vi "MAIN.vi"() -> ()   [LabVIEW 2015]
doc: "Use this template to create an application that executes repeatedly until you click the Stop button. This template polls the state of the Stop button and does not use events. Use the Top-Level Application template (not available in the Base package) to create a single-loop application with event handling."
uses:
  Control-CDC data.ctl
  Control-IMU data.ctl
  Control-Operation Test State FTS.ctl
  Lib_Bled112 toolkit/type_def/connection_status_bundle.ctl
  Lib_Bled112 toolkit/type_def/address_type.ctl
  Control-BLED Rx (EVENT-Attribute Client).ctl
  Lib_Bled112 toolkit/type_def/message_type.ctl
  Lib_Bled112 toolkit/type_def/message_class.ctl
  sub/Operation mode.ctl
  sub/Linerity State.ctl
  Cluster Type/Cal information.ctl
  Cluster Type/Device information.ctl
  <vilib>/Utility/miscctls.llb/LVPointTypeDef.ctl
  SUB_Load and Save Controls.llb/RWC_Actions.ctl
  <vilib>/Utility/miscctls.llb/LVRowAndColumnTypeDef.ctl
  Cluster Type/Acclerometer value(90, 180).ctl
  Type definition/write_mode.ctl
  Control-Operation State Mark10.ctl
  <vilib>/event_ctls.llb/eventvkey.ctl
  sub/File Control/File_Control_mode.ctl
  <vilib>/Analysis/baseanly.llb/Mean (DBL).vi
  <vilib>/Utility/config.llb/Read Key (String).vi
  <vilib>/Utility/config.llb/Read Key (I32).vi
  Lib_Bled112 toolkit/ble_functions/ble_write_by_handle_uint8array.vi
  global 3.vi
  global 4.vi
  Global 1.vi
  <vilib>/Utility/config.llb/Write Key (String).vi
  <vilib>/Utility/config.llb/Write Key (U32).vi
  <vilib>/Utility/config.llb/NI_LVConfig.lvlib
  <vilib>/Analysis/NI_AALBase.lvlib
  <vilib>/Utility/sysdir.llb/System Directory Type.ctl
  <vilib>/Utility/NIReport.llb/NI_report.lvclass
  <vilib>/addons/_office/NI_ReportGenerationToolkit.lvlib
  <vilib>/addons/_office/excel.llb/Excel Easy Table (str).vi
  <vilib>/Utility/NIReport.llb/Excel/NI_Excel.lvclass
  <vilib>/addons/_office/_exclsub.llb/font.ctl
panel:
  out "scale A,B check":u8
  out "scale A,B":T1 {"Check sum 2" format="%x"; "Device Type L" format="%x"; "Device Type H" format="%x"; "Check sum" format="%x"; "Scale B" format="%x"; "Scale A" format="%x"; "Manufacturer Lot ID 4" format="%x"; "Manufacturer Lot ID 3" format="%x"; "Manufacturer Lot ID 2" format="%x"; "Manufacturer Lot ID 1" format="%x"; "Day" format="%x"; "Month" format="%x"; "Year" format="%x"; "Device ID 4" format="%x"; "Device ID 3" format="%x"; "Device ID 2" format="%x"; "Device ID 1" format="%x"; "Packet ID" format="%x"}
  out "A3 rx":bool
  in  "A3 tx":bool
  out "A1 rx":bool
  in  "A1 tx":bool
  out "Port-act 1":refnum<visa-resource-name>="COM8"
  out "cal factor B":u8
  out "cal factor A":u8
  out "scale B":dbl format="%.2f"
  out "scale A":dbl format="%.2f"
  in  "PWR OFF":bool
  in  "File Path Done":bool
  in  "Linerity State":T2
  in  "Mode":bool=TRUE
  out "Bat(raw)":u16 format="%04x"
  out "Disconnection ocurrence":refnum<k4>
  out "Test Data table for Load Accuarcy Test":string[][](table)=[["-", "-", "-", "-", "-", "-", "-"], ["-", "-", "-", "-", "-", "-", "-"], ["-", "-", "-", "-", "-", "-", "-"], ["-", "-", "-", "-", "-", "-", "-"], ["-", "-", "-", "-", "-", "-", "-"], ["-", "-", "-", "-", "-", "-", "-"], ["-", "-", "-", "-", "-", "-", "-"], ["-", "-", "-", "-", "-", "-", "-"], ["-", "-", "-", "-", "-", "-", "-"]]
  out "Packet No.":u16
  out "Rx-debug":bool
  out "FTS table index":i32
  out "ms timer 5":u32=38996702
  out "ms timer 4":u32=27271323
  out "ms timer 3":u32=38996702
  in  "Update(ms)":u16=100
  out "ms timer 2":u32=38996702
  out "Rx-ROM":bool
  out "BLE Packet (mon)":u8[](array[numeric])=[119, 32, 48, 163, 32, 0, 45, 32, 53, 143, 30, 162, 83, 32, 86, 151, 32, 67, 185, 208, 89, 94, 66, 75, 91, 193, 107, 187, 98, 158, 102, 165, 208]
  out "Timer-ble log":u32=38996556
  in  "log data1":bool
  out "log ble buf":string
  out "Packet Detect":bool
  out "Disconnected":bool
  out "Rx buf 1":string
  out "Rx Cnt":i32
  out "Rx Packet Structure":T3={"Message Type (Response)"=128, "Payload length"=25, "Command Class (System)"=4, "Message ID"=5, "Connection handle"=0, "Attribute handle"=11, "Attribute type"=1, "Attribute value (data)"=[119, 32, 48, 110, 31, 255, 217, 32, 53, 83, 30, 161, 69, 32, 87, 130, 32, 68, 21, 209]} {"Attribute type" format="%02x" items=["read", "notify", "indicate", "read_by_type", "read_blob", "indicate_rsp_req"]; "Attribute value (data)" format="%02x"; "Attribute handle" format="%04x"; "Connection handle" format="%02x"; "Message ID" format="%02x"; "Message Type (Response)" format="%02x" items=["Command / Response"=0, "Event"=128]; "Command Class (System)" format="%02x" items=["System", "Persistent Store", "Attribute database", "Connection", "Attribute client", "Security Manager", "Generic Access Profile", "Hardware"]}
  out "Device Name":string="GEN4_PERSONA_3rd_jun"
  out "Connection Status":T6={"MAC Address"="F8:B8:54:EF:76:8D", "cnx handle"=0, "cnx flags"=5, "Address Type"=1, "Connection Interval (ms)"=8, "Timeout(ms)"=1000, "Latency"=0, "bonding handle"=255} {"Address Type" items=["Public", "Random"]}
  in  "Log no":string="1" caption="No."
  in  "FTS OP status":T8="Test_Start"
  out "Test profile":string[][](array[string])=[["Load(1)-0lb", "0", "1000", "0", "0"], ["Init(1)-70lb", "70", "1000", "0", "0"], ["Init(2)-140lb", "140", "1000", "0", "0"], ["Init(1)-70lb", "70", "1000", "0", "0"], ["Init(2)-140lb", "140", "1000", "0", "0"], ["Load(1)-0lb", "0", "10000", "1", "1"], ["Load(2)-10lb", "10", "3000", "0", "1"], ["Load(3)-20lb", "20", "3000", "0", "1"], ["Load(4)-40lb", "40", "3000", "0", "1"], ["Load(5)-60lb", "60", "3000", "0", "1"], ["Load(6)-80lb", "80", "3000", "0", "1"]]
  out "log refnum":refnum<file> caption="참조 번호 복제"
  out "ms timer":u32=38996556
  out "Logging No.":u32
  in  "Data Logging":bool caption="Data Logging (Desktop folder)"
  out "RxD":string
  out "Graph timer 2":u32=38996702
  out "Maximize window":bool
  out "Comm err cnt 1":i32
  out "Graph timer 1":u32=38996702
  in  "Setting load":bool=TRUE
  out "ACT-Comm":bool
  in  "Comm con 1":bool
  in  "Port close 1":bool
  in  "Port open 1":bool
  in  "탭-Top":T9(tab)
  out "recall-2":bool
  in  "CDC Graph plot":bool
  in  "Offset Souce":enum32{"Normal", "Raw"}(radio)
  out "CDC Offet":T10 caption="CDC Offset data" {"Right Wing-C, C6/C0" format="%#.9f"; "Right Wing-B, C5/C0" format="%#.9f"; "Right Wing-A, C4/C0" format="%#.9f"; "Left Wing-C, C3/C0" format="%#.9f"; "Left Wing-B, C2/C0" format="%#.9f"; "Left Wing-A, C1/C0" format="%#.9f"}
  in  "Export graph 1":bool
  in  "Clear graph 1":bool
  out "CDC(PCAP02) Graph":waveform(dbl)[](graph)=[{"t0"=timestamp(3566271640.952271 s since 1904-01-01), "dt"=0.10400000000000001, "Y"=[22878.0]}, {"t0"=timestamp(3566271640.952271 s since 1904-01-01), "dt"=0.10400000000000001, "Y"=[16971.0]}, {"t0"=timestamp(3566271640.952271 s since 1904-01-01), "dt"=0.10400000000000001, "Y"=[23489.0]}, {"t0"=timestamp(3566271640.952271 s since 1904-01-01), "dt"=0.10400000000000001, "Y"=[27579.0]}, {"t0"=timestamp(3566271640.952271 s since 1904-01-01), "dt"=0.10400000000000001, "Y"=[25246.0]}, {"t0"=timestamp(3566271640.952271 s since 1904-01-01), "dt"=0.10400000000000001, "Y"=[26279.0]}, {"t0"=timestamp(3566271640.952271 s since 1904-01-01), "dt"=0.10400000000000001, "Y"=[1.0058650970458984]}, {"t0"=timestamp(3566271640.952271 s since 1904-01-01), "dt"=0.10400000000000001, "Y"=[0.9999599456787109]}, {"t0"=timestamp(3566271640.952271 s since 1904-01-01), "dt"=0.10400000000000001, "Y"=[1.0064787864685059]}, {"t0"=timestamp(3566271640.952271 s since 1904-01-01), "dt"=0.10400000000000001, "Y"=[0.9571785926818848]}, {"t0"=timestamp(3566271640.952271 s since 1904-01-01), "dt"=0.10400000000000001, "Y"=[1.0106620788574219]}, {"t0"=timestamp(3566271640.952271 s since 1904-01-01), "dt"=0.10400000000000001, "Y"=[1.0083107948303223]}]
  out "CDC data":T10 caption="CDC Monitoring data" {"Right Wing-C, C6/C0" format="%#.9f"; "Right Wing-B, C5/C0" format="%#.9f"; "Right Wing-A, C4/C0" format="%#.9f"; "Left Wing-C, C3/C0" format="%#.9f"; "Left Wing-B, C2/C0" format="%#.9f"; "Left Wing-A, C1/C0" format="%#.9f"}
  in  "Offset 1":bool
  out "FTS 42 Rx":bool
  out "IMU Offet":T11 caption="IMU Offset data" {"Accelerometer Z" format="%#.9f"; "Accelerometer Y" format="%#.9f"; "Accelerometer X" format="%#.9f"; "Gyroscope Z" format="%#.9f"; "Gyroscope Y" format="%#.9f"; "Gyroscope X" format="%#.9f"}
  out "IMU Graph":waveform(dbl)[](graph)=[{"t0"=timestamp(3566271136.852438 s since 1904-01-01), "dt"=0.108, "Y"=[-1.063125]}, {"t0"=timestamp(3566271136.852438 s since 1904-01-01), "dt"=0.108, "Y"=[0.118125]}, {"t0"=timestamp(3566271136.852438 s since 1904-01-01), "dt"=0.108, "Y"=[0.20125]}, {"t0"=timestamp(3566271136.852438 s since 1904-01-01), "dt"=0.108, "Y"=[-0.014029999999999999]}, {"t0"=timestamp(3566271136.852438 s since 1904-01-01), "dt"=0.108, "Y"=[-0.00366]}, {"t0"=timestamp(3566271136.852438 s since 1904-01-01), "dt"=0.108, "Y"=[1.0149789999999999]}]
  in  "Clear graph 2":bool
  in  "Export graph2":bool
  out "IMU data":T11 caption="IMU Monitoring data" {"Accelerometer Z" format="%#.9f"; "Accelerometer Y" format="%#.9f"; "Accelerometer X" format="%#.9f"; "Gyroscope Z" format="%#.9f"; "Gyroscope Y" format="%#.9f"; "Gyroscope X" format="%#.9f"}
  in  "Offset 2":bool
  out "Full ROM data":bool
  in  "Flash Map":enum32{"Data Map", "Raw Data"}(tab)
  out "ROM Table":string[][](table)=[["Serial number", "-", "-"], ["YEAR", "-", "-"], ["Month", "-", "-"], ["Day", "-", "-"], ["Device ID", "-", "-"], ["Manufacturer ID", "-", "-"], ["Cal_Scale A", "-", "-"], ["Cal_Scale B", "-", "-"], ["Cal_Acc. X", "-", "-"], ["Cal_Acc. Y", "-", "-"], ["Cal_Acc. Z", "-", "-"], ["Cal_Gy. X", "-", "-"], ["Cal_Gy. Y", "-", "-"], ["Cal_Gy. Z", "-", "-"], ["Cal_Vol H", "-", "-"], ["Cal_Vol L", "-", "-"], ["Cal_CDC Off 1", "-", "-"], ["Cal_CDC Off 2", "-", "-"], ["Cal_CDC Off 3", "-", "-"], ["Cal_CDC Off 4", "-", "-"], ["Cal_CDC Off 5", "-", "-"], ["Cal_CDC Off 6", "-", "-"], ["Cal_CDC Off 7", "-", "-"], ["Cal_CDC Off 8", "-", "-"], ["Firmware Revision", "-", "-"], ["Operative Side", "-", "-"], ["Cal_Compart. A_10", "-", "-"], ["Cal_Compart. B_10", "-", "-"], ["Reserved", "-", "-"], ["Cal_Compart. A_11", "-", "-"], ["Cal_Compart. B_11", "-", "-"], ["Cal_Compart. A_12", "-", "-"], ["Cal_Compart. B_12", "-", "-"], ["Cal_Compart. A_13", "-", "-"], ["Cal_Compart. B_13", "-", "-"], ["Cal_Compart. A_14", "-", "-"], ["Cal_Compart. B_14", "-", "-"], ["Cal_Compart. A_16", "-", "-"], ["Cal_Compart. B_16", "-", "-"], ["Reserved", "-", "-"], ["Acc. X_0 value", "-", "-"], ["Acc. Y_0 value", "-", "-"], ["Acc. Z_0 value", "-", "-"], ["Acc. X_45 value", "-", "-"], ["Acc. Y_45 value", "-", "-"], ["Acc. Z_45 value", "-", "-"], ["Reserved", "-", "-"], ["Acc. X_90 value", "-", "-"], ["Acc. Y_90 value", "-", "-"], ["Acc. Z_90 value", "-", "-"], ["Acc. X_180 value", "-", "-"], ["Acc. Y_180 value", "-", "-"], ["Acc. Z_180 value", "-", "-"], ["Second counter", "-", "-"], ["Reserved", "-", "-"], ["", "", ""], ["", "", ""], ["", "", ""], ["", "", ""], ["", "", ""], ["", "", ""], ["", "", ""], ["", "", ""], ["", "", ""], ["", "", ""], ["", "", ""], ["", "", ""], ["", "", ""], ["", "", ""], ["", "", ""]]
  out "Rx ROM-log":string
  out "ROM Data":T12(array[cluster]) {"Index" format="%02x"; "ROM Data" format="%02x"}
  in  "Re-call":bool
  in  "Operation Mode":T13
  in  "Mode Selection":bool
  in  "Data Log":string
  out "Data_mon(h)":string
  in  "Data(h)":string="\u0001"
  in  "Send":bool
  in  "Handle":u8=15 format="%02x"
  in  "Mode Protocol":enum32{"Normal", "Debugging 1", "Debugging 2"}(tab)
  out "data out":u8[](array[numeric])
  in  "Reset Avg":bool caption="Reset"
  out "BLE RSSI Avg(dBm)":dbl format="%.1f"
  out "BLE Interval Time Avg(ms)":dbl format="%.1f"
  in  "File path":path
  in  "All Graph data save":bool
  in  "Set Inverval Time":bool
  in  "Grahp Clear":bool
  out "BLE RSSI buf":i16(graph)=-63
  out "BLE RSSI Graph":dbl(graph)=-65.56666666666666
  out "BLE RSSI (dBm)":dbl format="%.1f"
  out "BLE AVG-Interval Graph":dbl(graph)=11.355
  out "BLE Interval Time(ms)":dbl format="%.1f"
  out "BLE Interval buf":u32(graph)=11
  in  "Interval Time":enum16{"10ms", "33ms", "50ms"}(ring)
  out "second counter Rx":bool
  out "42 Rx":bool
  out "42 Tx":bool
  out "Battery cal Rx":bool
  out "Error":bool
  in  "battery cal Tx":bool
  out "battery cal complete boolean":bool
  out "Battery(V)":dbl format="%#_3g"
  out "inspection boolean":bool
  out "Linearity monitoring graph":cluster{dbl[], dbl[]}(graph)
  in  "ADC Linearity Start":bool
  out "battery cal value":dbl[](array[numeric])
  out "Status":string
  out "x/y":dbl
  out "Cal information":T14 {"Check sum" format="%x"; "Voltage L 2.8V" format="%x"; "Voltage H 2.8V" format="%x"; "Voltage L 3.1V" format="%x"; "Acc Z_L_Cal" format="%x"; "Voltage H 3.1V" format="%x"; "Gyro Z_L_Cal" format="%x"; "Gyro Z_H_Cal" format="%x"; "Gyro Y_L_Cal" format="%x"; "Gyro Y_H_Cal" format="%x"; "Gyro X_L_Cal" format="%x"; "Gyro X_H_Cal" format="%x"; "Acc Z_H_Cal" format="%x"; "Acc Y_L_Cal" format="%x"; "Acc Y_H_Cal" format="%x"; "Acc X_L_Cal" format="%x"; "Acc X_H_Cal" format="%x"; "Packet ID" format="%x"}
  out "cluster":T14 {"Check sum" format="%x"; "Voltage L 2.8V" format="%x"; "Voltage H 2.8V" format="%x"; "Voltage L 3.1V" format="%x"; "Acc Z_L_Cal" format="%x"; "Voltage H 3.1V" format="%x"; "Gyro Z_L_Cal" format="%x"; "Gyro Z_H_Cal" format="%x"; "Gyro Y_L_Cal" format="%x"; "Gyro Y_H_Cal" format="%x"; "Gyro X_L_Cal" format="%x"; "Gyro X_H_Cal" format="%x"; "Acc Z_H_Cal" format="%x"; "Acc Y_L_Cal" format="%x"; "Acc Y_H_Cal" format="%x"; "Acc X_L_Cal" format="%x"; "Acc X_H_Cal" format="%x"; "Packet ID" format="%x"}
  out "FTS start":bool
  out "FTS device out":bool
  out "scale A,B Rx":bool
  out "scale A.B Tx":bool
  out "second counter Tx":bool
  in  "Cal/Test select":bool=TRUE
  in  "Head Up":bool
  in  "Load(lb)":dbl=10.0 min=0.0 max=150.0 step=0.1
  in  "Test name":string="Noname"
  out "Load Graph":cluster{dbl[], dbl[]}(graph)
  out "Mark10 Gauge (lb)":dbl format="%.2f"
  out "Test Status":string
  out "Test Data table":string[][](table)=[["-", "-", "-", "-", "-", "-", "-"], ["-", "-", "-", "-", "-", "-", "-"], ["-", "-", "-", "-", "-", "-", "-"], ["-", "-", "-", "-", "-", "-", "-"], ["-", "-", "-", "-", "-", "-", "-"], ["-", "-", "-", "-", "-", "-", "-"], ["-", "-", "-", "-", "-", "-", "-"], ["-", "-", "-", "-", "-", "-", "-"], ["-", "-", "-", "-", "-", "-", "-"]]
  in  "Test Start":bool
  in  "Port-FTS":refnum<visa-resource-name>="COM6" caption="FTS \nCOM port"
  in  "FTS Testing":bool
  out "FTS comm.":bool
  in  "Force Set":bool
  out "FTS 42 Tx":bool
  out "88 rx":bool
  out "83 rx":bool
  in  "88 tx":bool
  in  "83 tx":bool
  out "81 rx":bool
  in  "Save":bool
  in  "ROM Table 2":string[][](table)=[["Serial number", "1", "MAX Value: 4294967295 (FFFFFFFFh)"], ["YEAR", "2", "Year: 2002, MAX Value: 255 (FFh)"], ["Month", "3", "Month:  3, MAX Value: 255 (FFh)"], ["Day", "4", "Day:  4, MAX Value: 255 (FFh)"], ["Device ID", "5", "-"], ["Manufacturer ID", "6", "MAX Value: 4294967295 (FFFFFFFFh)"], ["Cal_Scale A", "7", "MAX Value: 255 (FF)"], ["Cal_Scale B", "8", "MAX Value: 255 (FF)"], ["Cal_Acc. X", "9", "-"], ["Cal_Acc. Y", "10", "-"], ["Cal_Acc. Z", "11", "-"], ["Cal_Gy. X", "12", "-"], ["Cal_Gy. Y", "13", "-"], ["Cal_Gy. Z", "14", "-"], ["Cal_Vol H", "2910", "-"], ["Cal_Vol L", "16", "-"], ["Cal_CDC Off 1", "17", "-"], ["Cal_CDC Off 2", "18", "-"], ["Cal_CDC Off 3", "19", "-"], ["Cal_CDC Off 4", "20", "-"], ["Cal_CDC Off 5", "21", "-"], ["Cal_CDC Off 6", "22", "-"], ["Cal_CDC Off 7", "23", "-"], ["Cal_CDC Off 8", "24", "-"], ["Firmware Revision", "25", "-"], ["Operative Side", "26", "-"], ["Cal_Compart. A_10", "27", "-"], ["Cal_Compart. B_10", "28", "-"], ["Reserved", "29", "-"], ["Cal_Compart. A_11", "30", "-"], ["Cal_Compart. B_11", "31", "-"], ["Cal_Compart. A_12", "32", "-"], ["Cal_Compart. B_12", "33", "-"], ["Cal_Compart. A_13", "34", "-"], ["Cal_Compart. B_13", "35", "-"], ["Cal_Compart. A_14", "36", "-"], ["Cal_Compart. B_14", "37", "-"], ["Cal_Compart. A_16", "38", "-"], ["Cal_Compart. B_16", "39", "-"], ["Reserved", "40", "-"], ["Acc. X_0 value", "41", "-"], ["Acc. Y_0 value", "42", "-"], ["Acc. Z_0 value", "43", "-"], ["Acc. X_45 value", "44", "-"], ["Acc. Y_45 value", "45", "-"], ["Acc. Z_45 value", "46", "-"], ["Reserved", "47", "-"], ["Acc. X_90 value", "48", "-"], ["Acc. Y_90 value", "49", "-"], ["Acc. Z_90 value", "50", "-"], ["Acc. X_180 value", "51", "-"], ["Acc. Y_180 value", "52", "-"], ["Acc. Z_180 value", "53", "-"], ["Second counter", "17454", "-"], ["Reserved", "8", "-"], ["", "", ""], ["", "", ""], ["", "", ""], ["", "", ""], ["", "", ""], ["", "", ""], ["", "", ""], ["", "", ""], ["", "", ""], ["", "", ""], ["", "", ""], ["", "", ""], ["", "", ""], ["", "", ""], ["", "", ""]] caption="ROM Table"
  out "x-y":u8 format="%x"
  out "81 checksum":u8
  out "91 checksum":u8
  out "83 checksum":u8
  out "88 checksum":u8
  out "bat cal_check sum":u8
  out "sec coun_check sum":u8
  in  "91 tx":bool
  out "91 rx":bool
  out "A3 checksum":u8
  out "A1 checksum":u8
  out "98 checksum":u8
  out "94 checksum":u8
  out "92 checksum":u8
  in  "92 tx":bool
  out "92 rx":bool
  in  "94 tx":bool
  out "94 rx":bool
  in  "98 tx":bool
  out "98 rx":bool
  out "Rx-mon":bool
  out "Comm con status 1":bool caption="Status"
  out "*Board ID1":string="None...." caption="S/N"
  in  "Port-set 1":refnum<visa-resource-name>="COM8" caption="COM port"
  in  "stop":bool=TRUE
  out "Data trx(led)":bool
  in  "Setting load(led)":bool
  out "status string":string="Ready (available after the communication connection)"
  # "GEN4 PP4 - GUI Program"
  # "Ver. 170823A"
  # "Comm. Connection"
  # "(Connection)"
  # "Serial port"
  # "Reserved"
  # "Gyroscope X"
  # "Gyroscope Y"
  # "Gyro. (dps)"
  # "Gyroscope Z"
  # "Accelerometer X"
  # "Accelerometer Y"
  # "Acc. (g)"
  # "Accelerometer Z"
  # "Unless otherwise specified, Maximum value is 65535(FFFFh)."
  # "* Normal Operation Mode\nHandler : 0x000B\nWrite : 0x69 0x6D 0x74"
  # "* Debugging Mode 1\nHandler : 0x000B\nWrite : 0x4A 0x73 0x50"
  # "* Debugging Mode 2\nHandler : 0x000B\nWrite : 0x4E 0x46 0x54"
  # "Battery Calibration"
  # "ESM301: 115200bps\nMARK10: 9600bps"
  # "Unless otherwise specified, Maximum value is 65535 (FFFFh)."
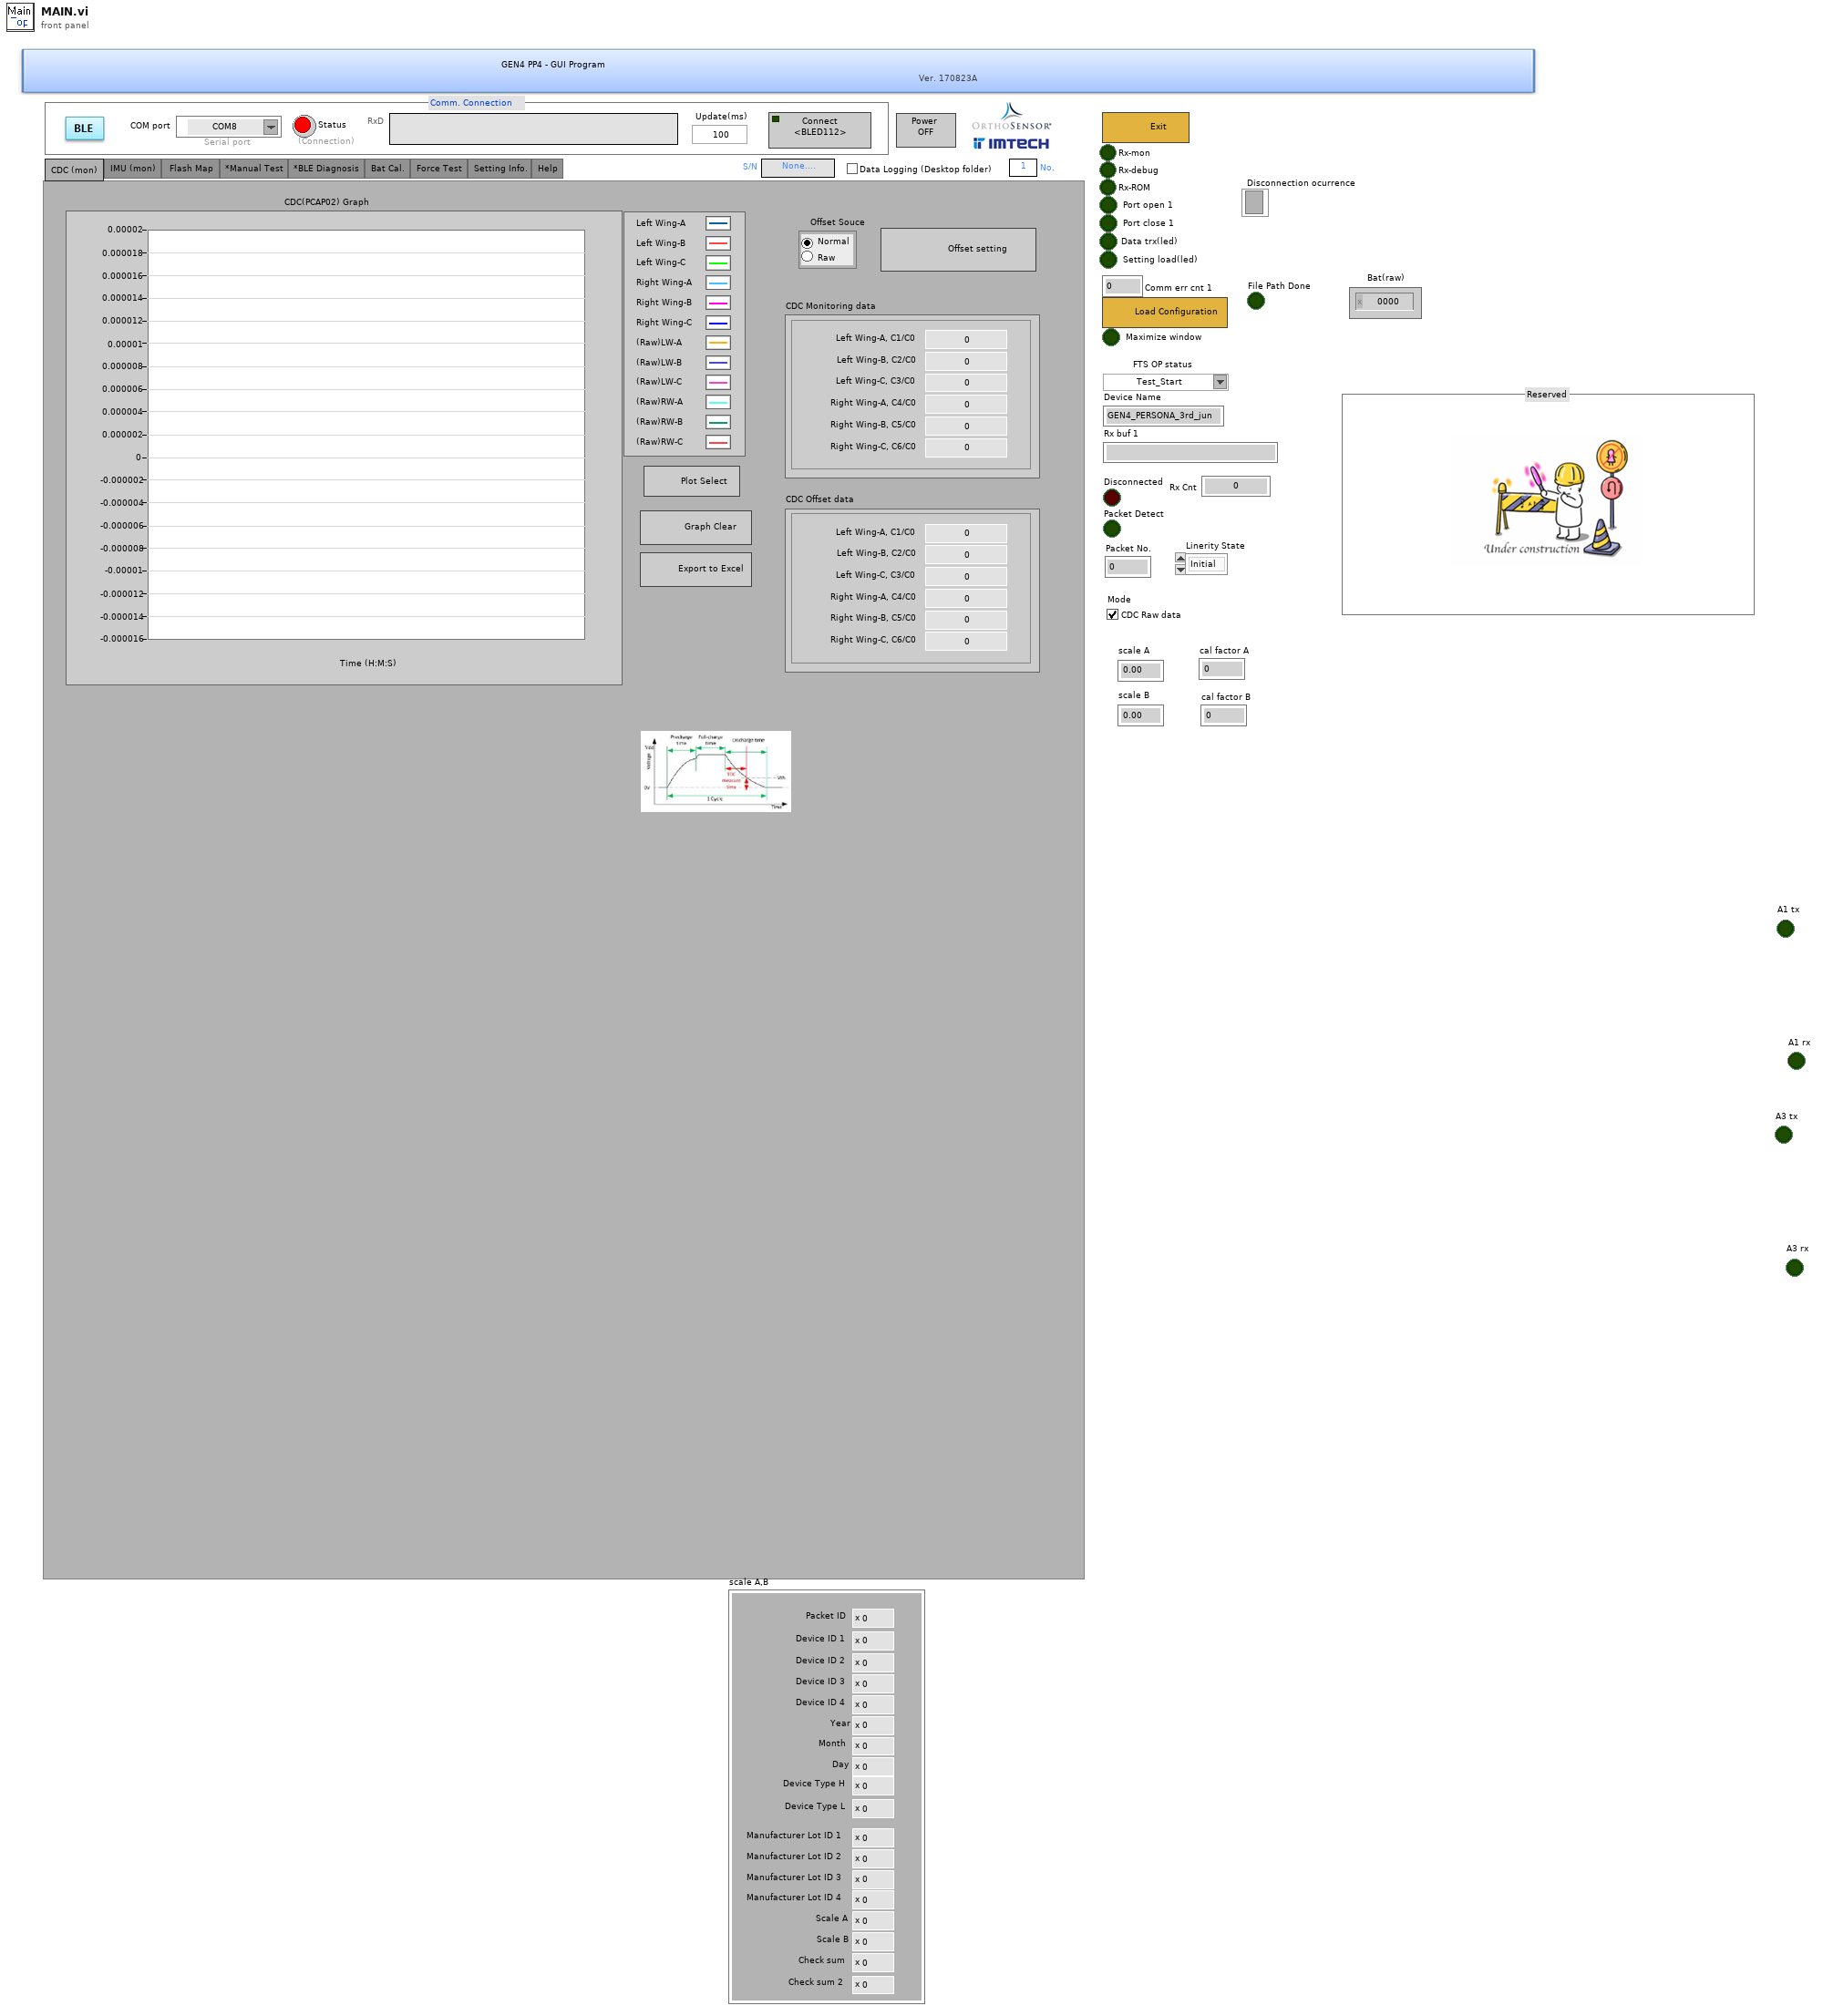
[diagram p1: front panel]
types:
  T1 = typedef "Device information.ctl" = cluster{"Packet ID":u8, "Device ID 1":u8, "Device ID 2":u8, "Device ID 3":u8, "Device ID 4":u8, "Year":u8, "Month":u8, "Day":u8, "Device Type H":u8, "Device Type L":u8, "Manufacturer Lot ID 1":u8, "Manufacturer Lot ID 2":u8, "Manufacturer Lot ID 3":u8, "Manufacturer Lot ID 4":u8, "Scale A":u8, "Scale B":u8, "Check sum":u8, "Check sum 2":u8}
  T2 = typedef "Linerity State.ctl" = enum16{"Initial", "Measurement", "End"}
  T3 = typedef "Control-BLED Rx (EVENT-Attribute Client).ctl" = cluster{"Message Type (Response)":T4, "Payload length":u8, "Command Class (System)":T5, "Message ID":u8, "Connection handle":u8, "Attribute handle":u16, "Attribute type":T5, "Attribute value (data)":u8[]}
  T4 = typedef "message_type.ctl" = u8
  T5 = typedef "message_class.ctl" = u8
  T6 = typedef "connection_status_bundle.ctl" = cluster{"MAC Address":string, "cnx handle":u8, "cnx flags":u8, "Address Type":T7, "Connection Interval (ms)":u16, "Timeout(ms)":u16, "Latency":u16, "bonding handle":u8}
  T7 = typedef "address_type.ctl" = u8
  T8 = typedef "Control-Operation Test State FTS.ctl" = string
  T9 = enum32{"CDC (mon)", "IMU (mon)", "Flash Map ", "*Manual Test", "*BLE Diagnosis", "Bat Cal.", "Force Test", "Setting Info.", "Help"}
  T10 = typedef "Control-CDC data.ctl" = cluster{"Left Wing-A, C1/C0":dbl, "Left Wing-B, C2/C0":dbl, "Left Wing-C, C3/C0":dbl, "Right Wing-A, C4/C0":dbl, "Right Wing-B, C5/C0":dbl, "Right Wing-C, C6/C0":dbl}
  T11 = typedef "Control-IMU data.ctl" = cluster{"Gyroscope X":dbl, "Gyroscope Y":dbl, "Gyroscope Z":dbl, "Accelerometer X":dbl, "Accelerometer Y":dbl, "Accelerometer Z":dbl}
  T12 = cluster{"RxOK":bool, "ROM Data":u8[], "Index":u8}[]
  T13 = typedef "Operation mode.ctl" = enum16{"Normal Operation", "Debugging 1", "Debugging 2"}
  T14 = typedef "Cal information.ctl" = cluster{"Packet ID":u8, "Acc X_H_Cal":u8, "Acc X_L_Cal":u8, "Acc Y_H_Cal":u8, "Acc Y_L_Cal":u8, "Acc Z_H_Cal":u8, "Acc Z_L_Cal":u8, "Gyro X_H_Cal":u8, "Gyro X_L_Cal":u8, "Gyro Y_H_Cal":u8, "Gyro Y_L_Cal":u8, "Gyro Z_H_Cal":u8, "Gyro Z_L_Cal":u8, "Voltage H 3.1V":u8, "Voltage L 3.1V":u8, "Voltage H 2.8V":u8, "Voltage L 2.8V":u8, "Check sum":u8}
  T15 = enum8{"Enabled", "Disabled", "Disabled and Grayed Out"}
  T16 = typedef "RWC_Actions.ctl" = enum16{"Read", "Write", "Read and Create"}
  T17 = enum16{"Always On", "Always Off", "Off While Running"}
  T18 = typedef "LVPointTypeDef.ctl" = cluster{"Horizontal":i16, "Vertical":i16}
  T19 = cluster{"RxOK":bool, "ROM Data":u8[], "Index":u8}
  T20 = typedef "LVRowAndColumnTypeDef.ctl" = cluster{"Row":i32, "Column":i32}
  T21 = enum16{"Standard Report", "HTML", "Word", "Excel"}
  T22 = enum16{"maximized", "minimized", "normal", "no change"}
  T23 = typedef "NI_ReportGenerationToolkit.lvlib/font.ctl" = cluster{"font name":string, "font size":dbl, "bold":u16, "italic":u16, "underline":u16, "strike through":u16, "font color":u32}
  T24 = cluster{"on/off":bool, "weight":i32, "color":u32}
  T25 = typedef "Acclerometer value(90, 180).ctl" = cluster{"Packet ID":u8, "Acc. X_90 val_H":u8, "Acc. X_90 val_L":u8, "Acc. Y_90 val_H":u8, "Acc. Y_90 val_L":u8, "Acc. Z_90 val_H":u8, "Acc. Z_90 val_L":u8, "Acc. X_180 val_H":u8, "Acc. X_180 val_L":u8, "Acc. Y_180 val_H":u8, "Acc. Y_180 val_L":u8, "Acc. Z_180 val_H":u8, "Acc. Z_180 val_L":u8, "second counter_1":u8, "second counter_2":u8, "Reserved_1":u8, "Reserved_2":u8, "Check sum":u8}
  T26 = typedef "write_mode.ctl" = enum16{"Save Flash", "Visa save", "Interval Change"}
  T27 = typedef "Control-Operation State Mark10.ctl" = string
  T28 = typedef "eventvkey.ctl" = enum16{"ASCII", "Enter", "Return", "Shift", "Ctrl", "Alt", "Cmd", "Opt", "Caps", "NumLock", "Clear", "Break", "Up", "Down", "Left", "Right", "Insert", "Delete", "Home", "End", "PageUp", "PageDown", "Escape", "Help", "Pause", "ScrollLock", "F1", "F2", "F3", "F4", "F5", "F6", "F7", "F8", "F9", "F10", "F11", "F12", "F13", "F14", "F15", "F16", "F17", "F18", "F19", "F20", "F21", "F22", "F23", "F24", "Play", "VolumeUp", "VolumeDown", "Mute", "Two Byte Char"}
  T29 = typedef "File_Control_mode.ctl" = enum16{"Open", "Write", "Close"}
  T30 = cluster{"LWA":dbl[], "LWB":dbl[], "LWC":dbl[], "RWA":dbl[], "RWB":dbl[], "RWC":dbl[], "Bat":u16[]}
  T31 = enum16{"open", "replace", "create", "open or create", "replace or create", "replace or create with confirmation"}
  T32 = typedef "NI_LVConfig.lvlib/Config Data RefNum.ctl" = refnum<k1>
  T33 = typedef "System Directory Type.ctl" = i32
  T34 = typedef "PCAP zero information.ctl" = cluster{"Packet ID":u8, "Sensor 1_H":u8, "Sensor 1_L":u8, "Sensor 2_H":u8, "Sensor 2_L ":u8, "Sensor 3_H":u8, "Sensor 3_L":u8, "Sensor 4_H":u8, "Sensor 4_L":u8, "Sensor 5_H":u8, "Sensor 5_L":u8, "Sensor 6_H":u8, "Sensor 6_L":u8, "Sensor 7_H":u8, "Sensor 7_L":u8, "Sensor 8_H":u8, "Sensor 8_L":u8, "Check sum":u8}
  T35 = typedef "add data1.ctl" = cluster{"Packet ID":u8, "Firmware Revision":u8, "Operative Side":u8, "Cal_Compart. A_10_1":u8, "Cal_Compart. A_10_2":u8, "Cal_Compart. A_10_3":u8, "Cal_Compart. A_10_4":u8, "Cal_Compart. B_10_1":u8, "Cal_Compart. B_10_2":u8, "Cal_Compart. B_10_3":u8, "Cal_Compart. B_10_4":u8, "Reserved_1":u8, "Reserved_2":u8, "Reserved_3":u8, "Reserved_4":u8, "Reserved_5":u8, "Reserved_6":u8, "Check sum":u8}
  T36 = typedef "add data3.ctl" = cluster{"Packet ID":u8, "Cal_Compart. A_13_1":u8, "Cal_Compart. A_13_2":u8, "Cal_Compart. A_13_3":u8, "Cal_Compart. A_13_4":u8, "Cal_Compart. B_13_1":u8, "Cal_Compart. B_13_2":u8, "Cal_Compart. B_13_3":u8, "Cal_Compart. B_13_4":u8, "Cal_Compart. A_14_1":u8, "Cal_Compart. A_14_2":u8, "Cal_Compart. A_14_3":u8, "Cal_Compart. A_14_4":u8, "Cal_Compart. B_14_1":u8, "Cal_Compart. B_14_2":u8, "Cal_Compart. B_14_3":u8, "Cal_Compart. B_14_4":u8, "Check sum":u8}
  T37 = typedef "add data4.ctl" = cluster{"Packet ID":u8, "Cal_Compart. A_16_1":u8, "Cal_Compart. A_16_2":u8, "Cal_Compart. A_16_3":u8, "Cal_Compart. A_16_4":u8, "Cal_Compart. B_16_1":u8, "Cal_Compart. B_16_2":u8, "Cal_Compart. B_16_3":u8, "Cal_Compart. B_16_4":u8, "Reserved_1":u8, "Reserved_2":u8, "Reserved_3":u8, "Reserved_4":u8, "Reserved_5":u8, "Reserved_6":u8, "Reserved_7":u8, "Reserved_8":u8, "Check sum":u8}
  T38 = typedef "Acclerometer value(0, 45).ctl" = cluster{"Packet ID":u8, "Acc. X_0 val_H":u8, "Acc. X_0 val_L":u8, "Acc. Y_0 val_H":u8, "Acc. Y_0 val_L":u8, "Acc. Z_0 val_H":u8, "Acc. Z_0 val_L":u8, "Acc. X_45 val_H":u8, "Acc. X_45 val_L":u8, "Acc. Y_45 val_H":u8, "Acc. Y_45 val_L":u8, "Acc. Z_45 val_H":u8, "Acc. Z_45 val_L":u8, "Reserved_1":u8, "Reserved_2":u8, "Reserved_3":u8, "Reserved_4":u8, "Check sum":u8}
  T39 = typedef "add data2.ctl" = cluster{"Packet ID":u8, "Cal_Compart. A_11_1":u8, "Cal_Compart. A_11_2":u8, "Cal_Compart. A_11_3":u8, "Cal_Compart. A_11_4":u8, "Cal_Compart. B_11_1":u8, "Cal_Compart. B_11_2":u8, "Cal_Compart. B_11_3":u8, "Cal_Compart. B_11_4":u8, "Cal_Compart. A_12_1":u8, "Cal_Compart. A_12_2":u8, "Cal_Compart. A_12_3":u8, "Cal_Compart. A_12_4":u8, "Cal_Compart. B_12_1":u8, "Cal_Compart. B_12_2":u8, "Cal_Compart. B_12_3":u8, "Cal_Compart. B_12_4":u8, "Check sum":u8}
  T40 = typedef "Control-BLED Rx (EVENT-Connection status).ctl" = cluster{"Message Type (Response)":T4, "Payload length":u8, "Command Class (System)":T5, "Message ID":u8, "Connection handle":u8, "flags":u8, "Bluetooth address":u8[], "address type":T5, "conn_interval(ms)":dbl, "timeout(ms)":dbl, "latency":u16, "bonding(0xFF)":u8}
  T41 = typedef "Control-BLED Rx (Get RSSI).ctl" = cluster{"Message Type (Response)":T4, "Payload length":u8, "Message class":u8, "Message ID":u8, "connection":u8, "rssi":i16}
  T42 = typedef "LVRectTypeDef.ctl" = cluster{"Left":i16, "Top":i16, "Right":i16, "Bottom":i16}
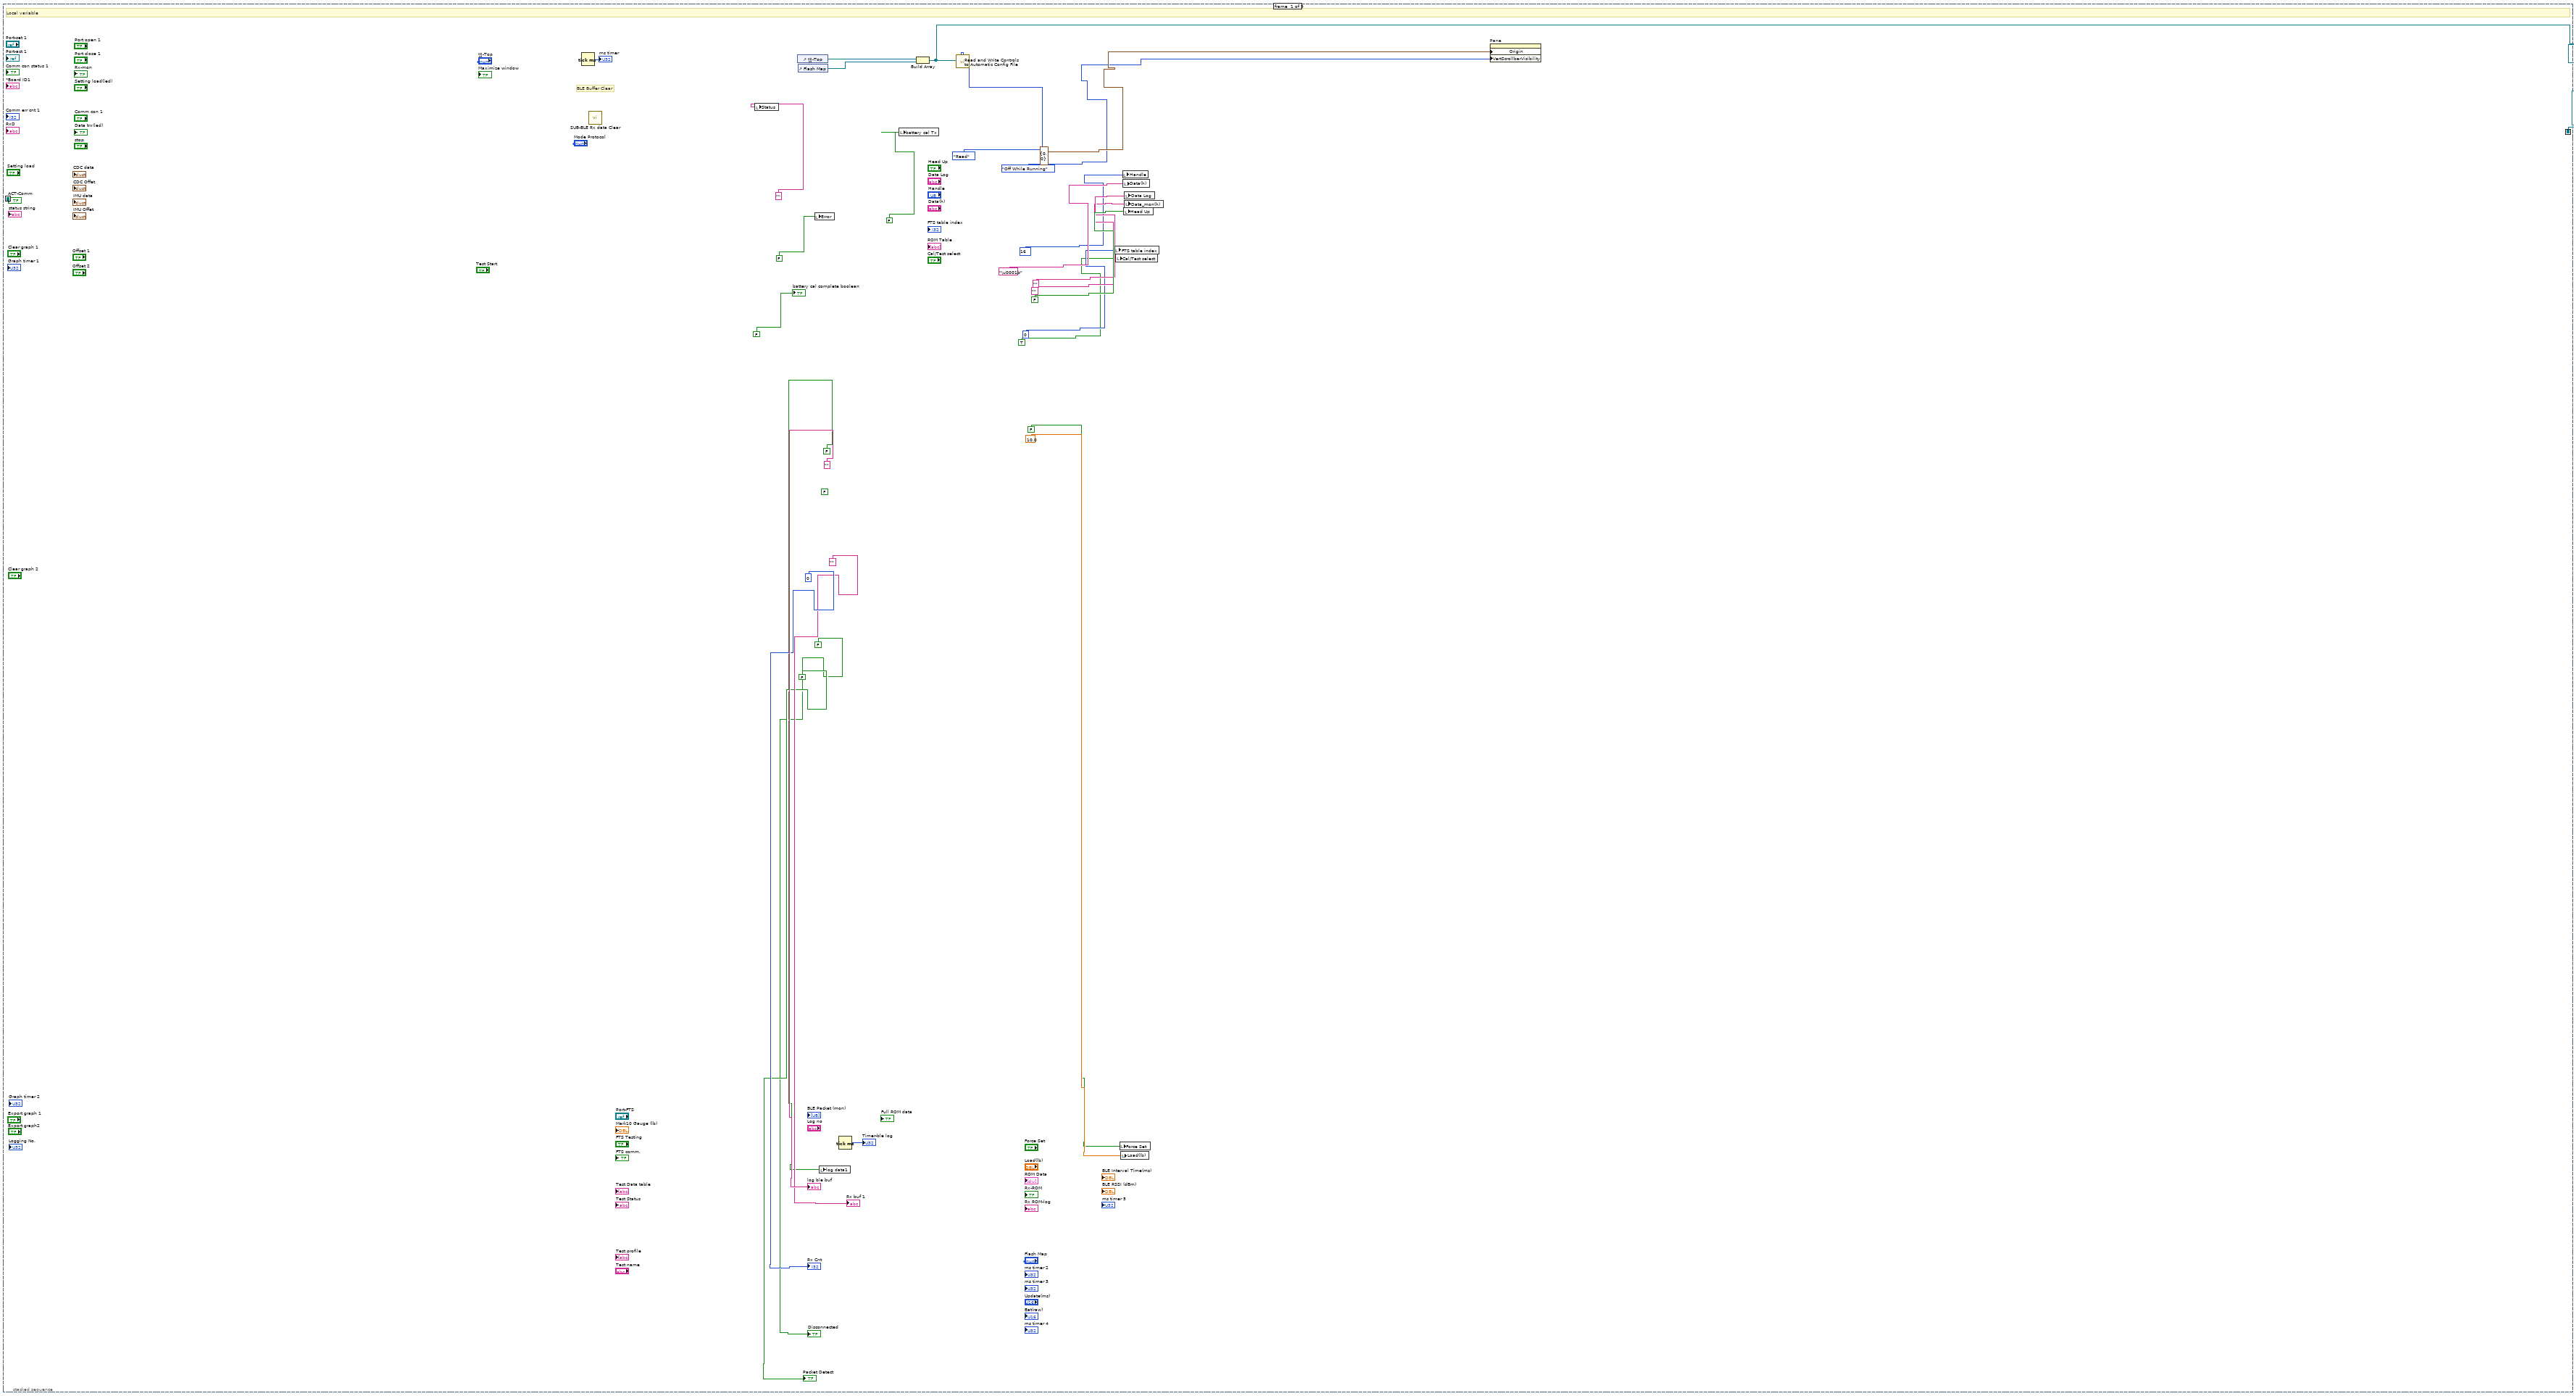
[diagram p2: hidden frame]
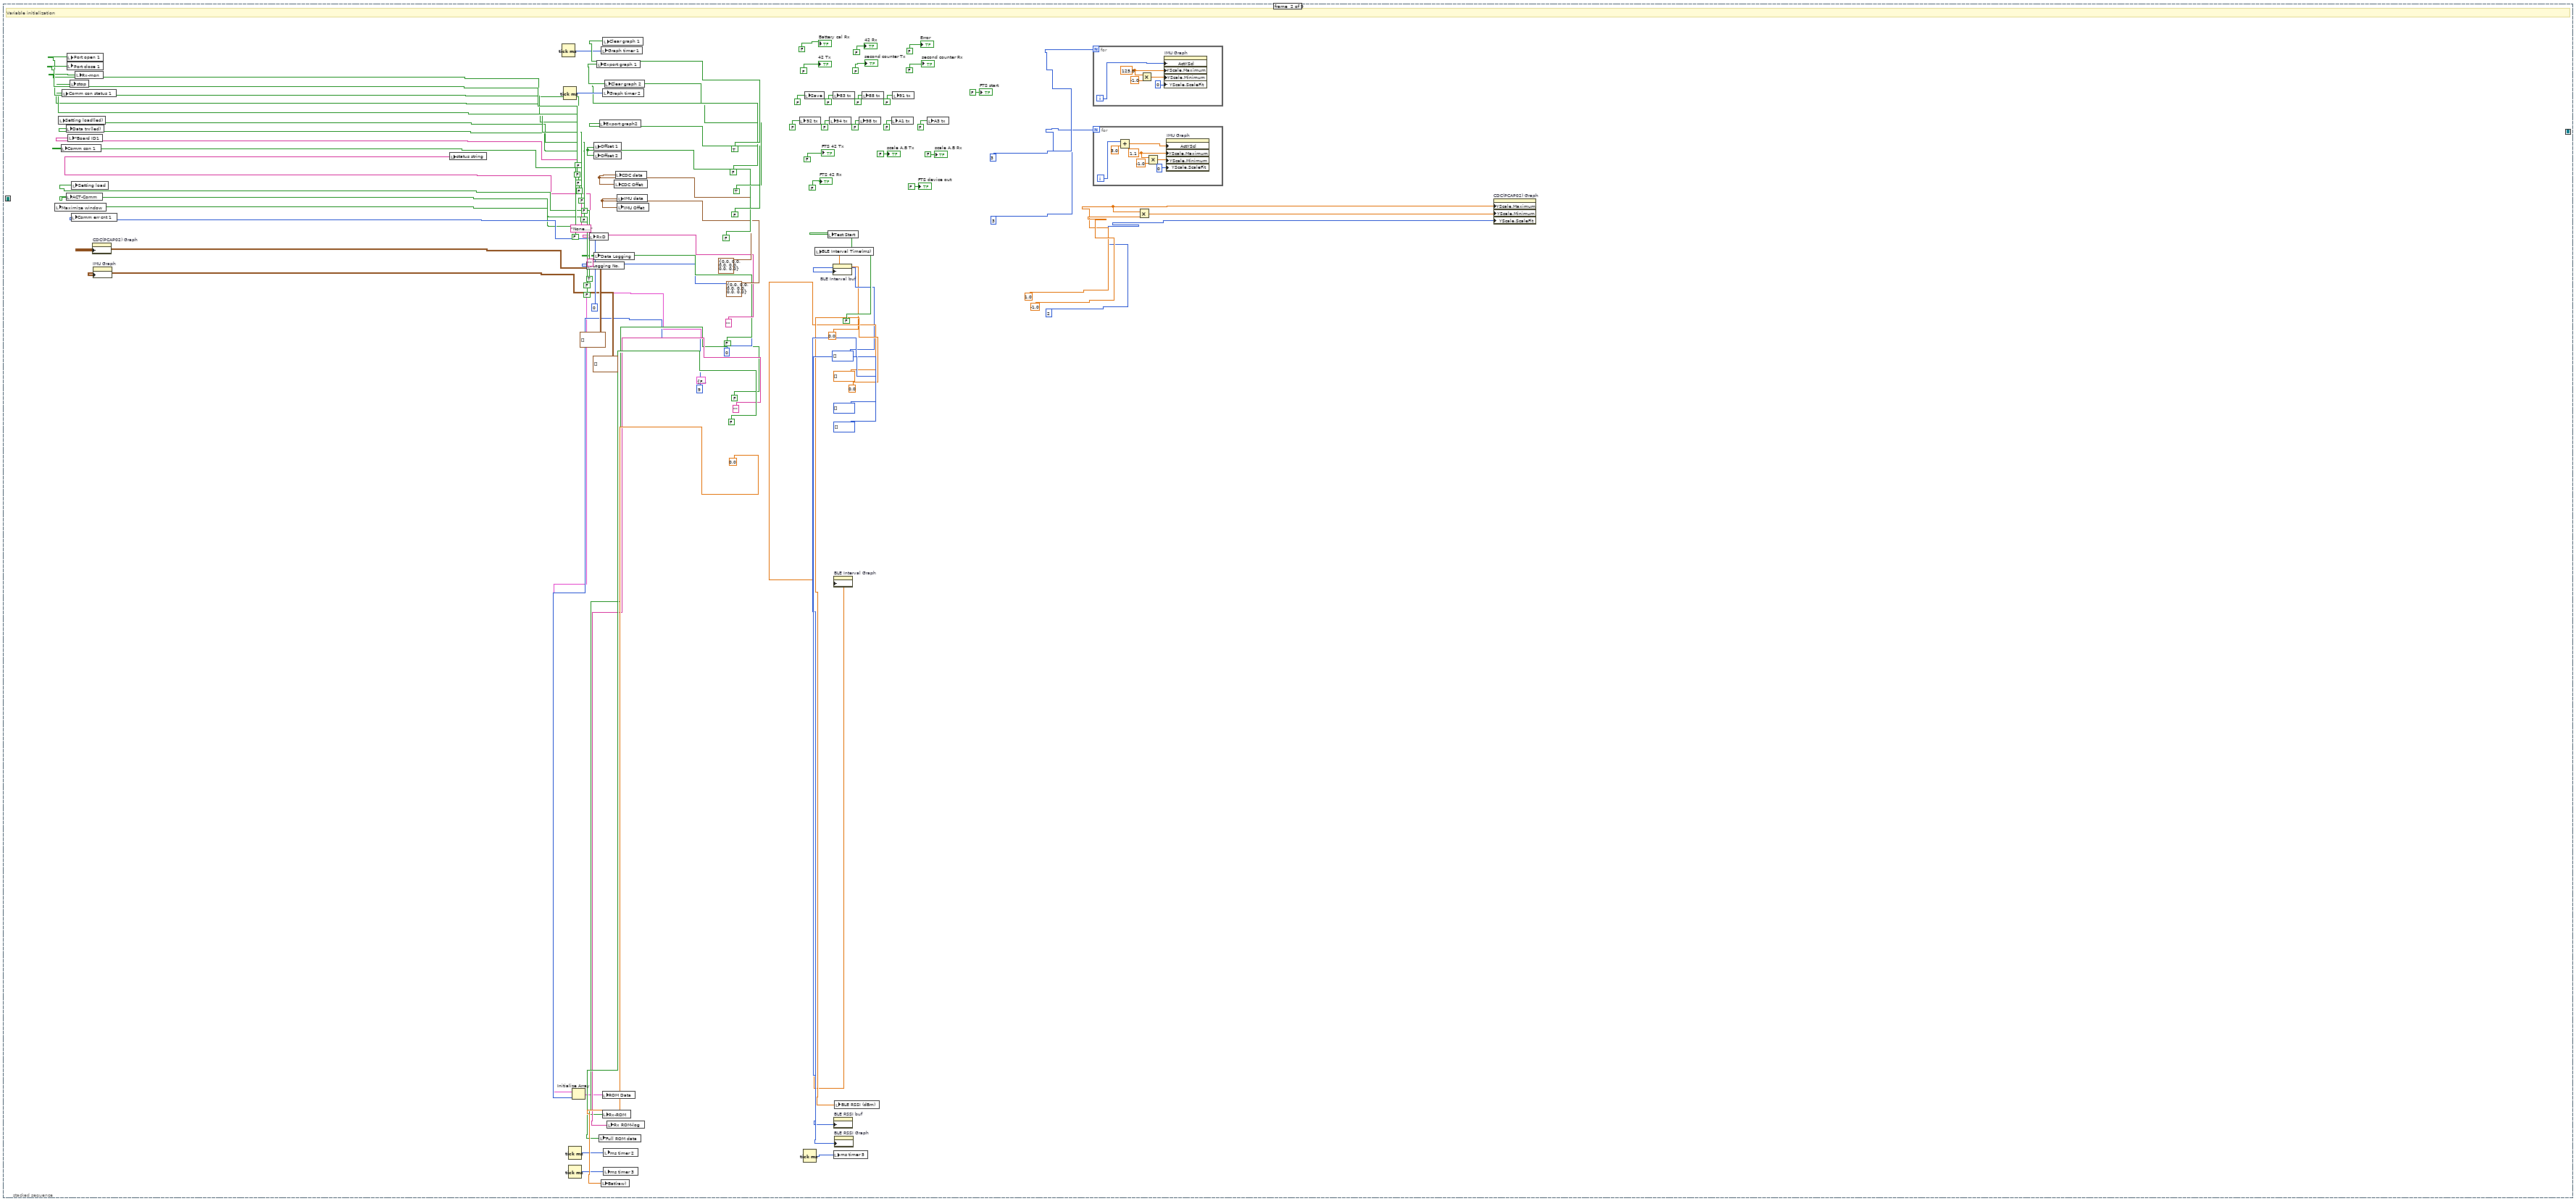
[diagram p3: hidden frame]
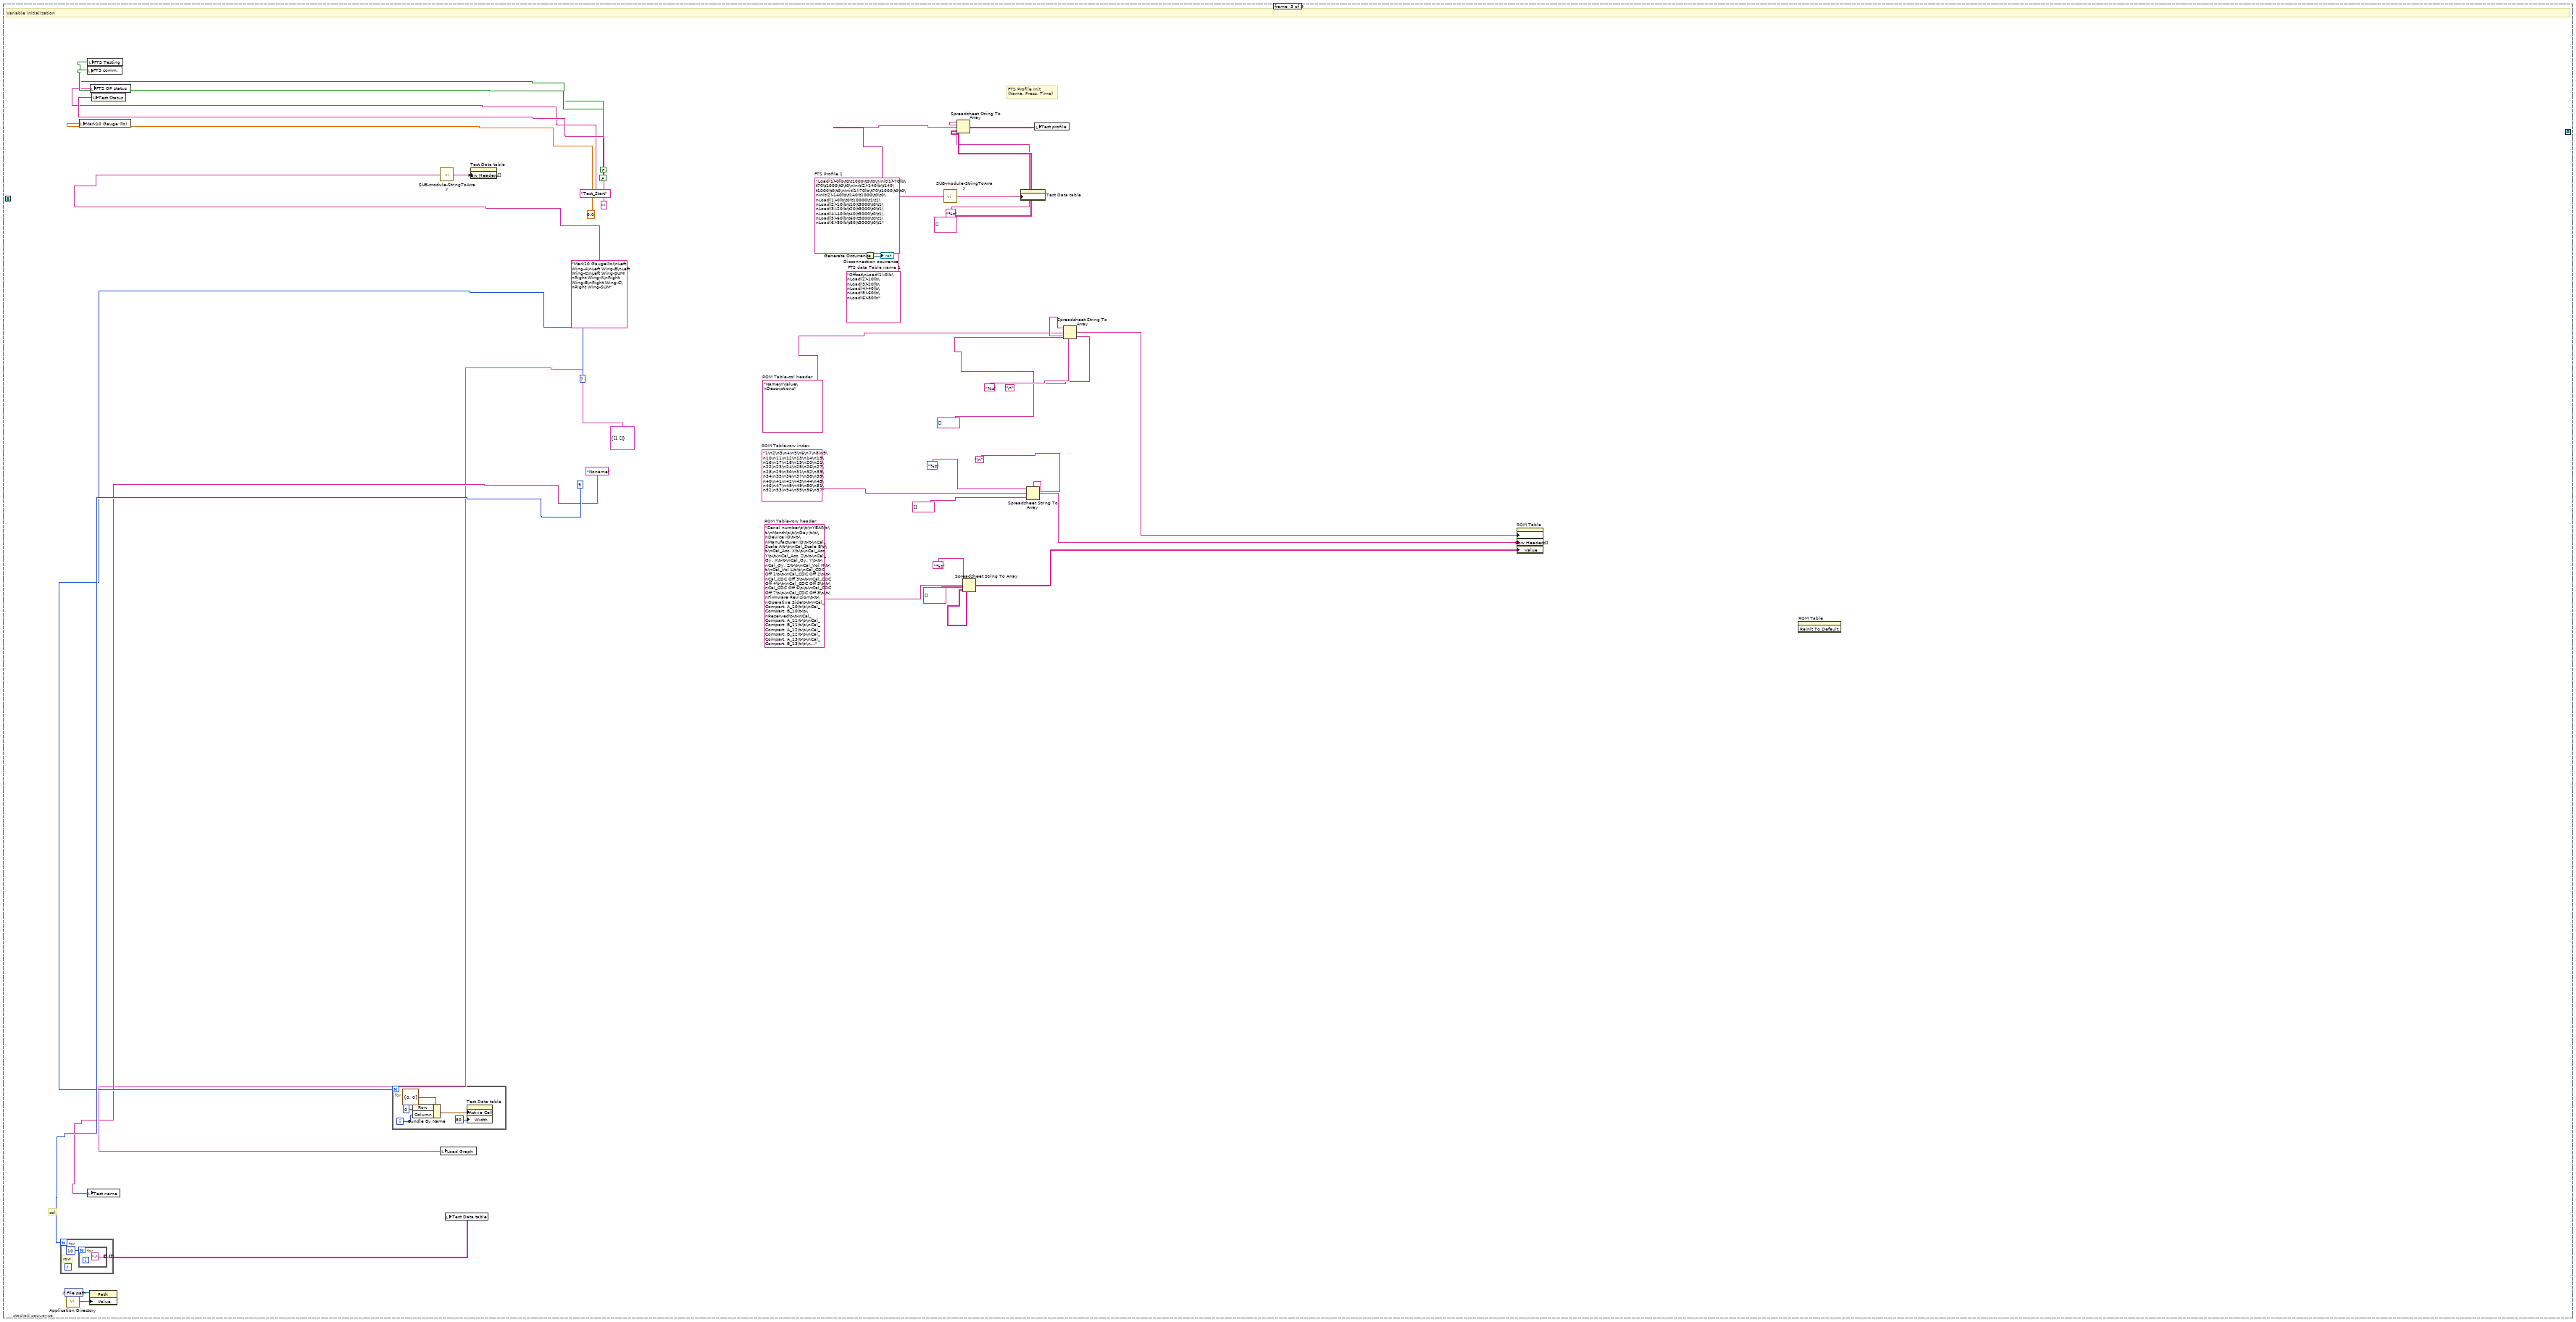
[diagram p4: hidden frame]
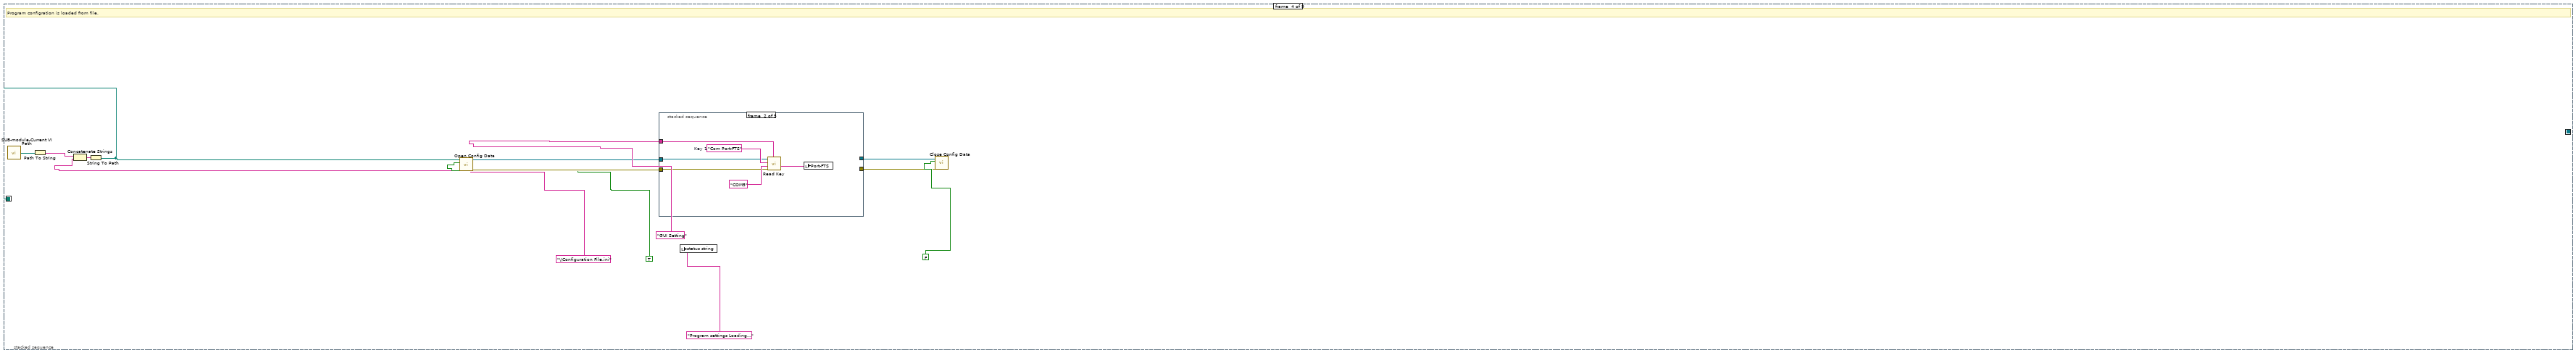
[diagram p5: hidden frame]
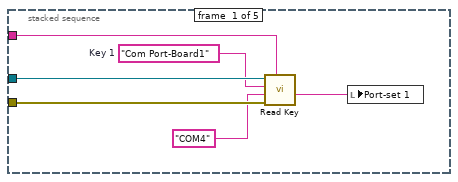
[diagram p6: hidden frame]
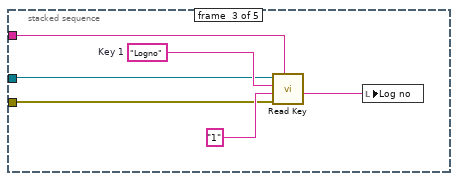
[diagram p7: hidden frame]
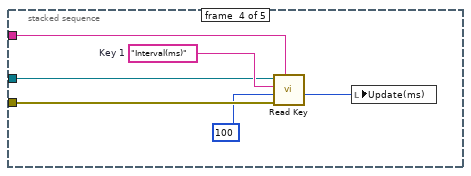
[diagram p8: hidden frame]
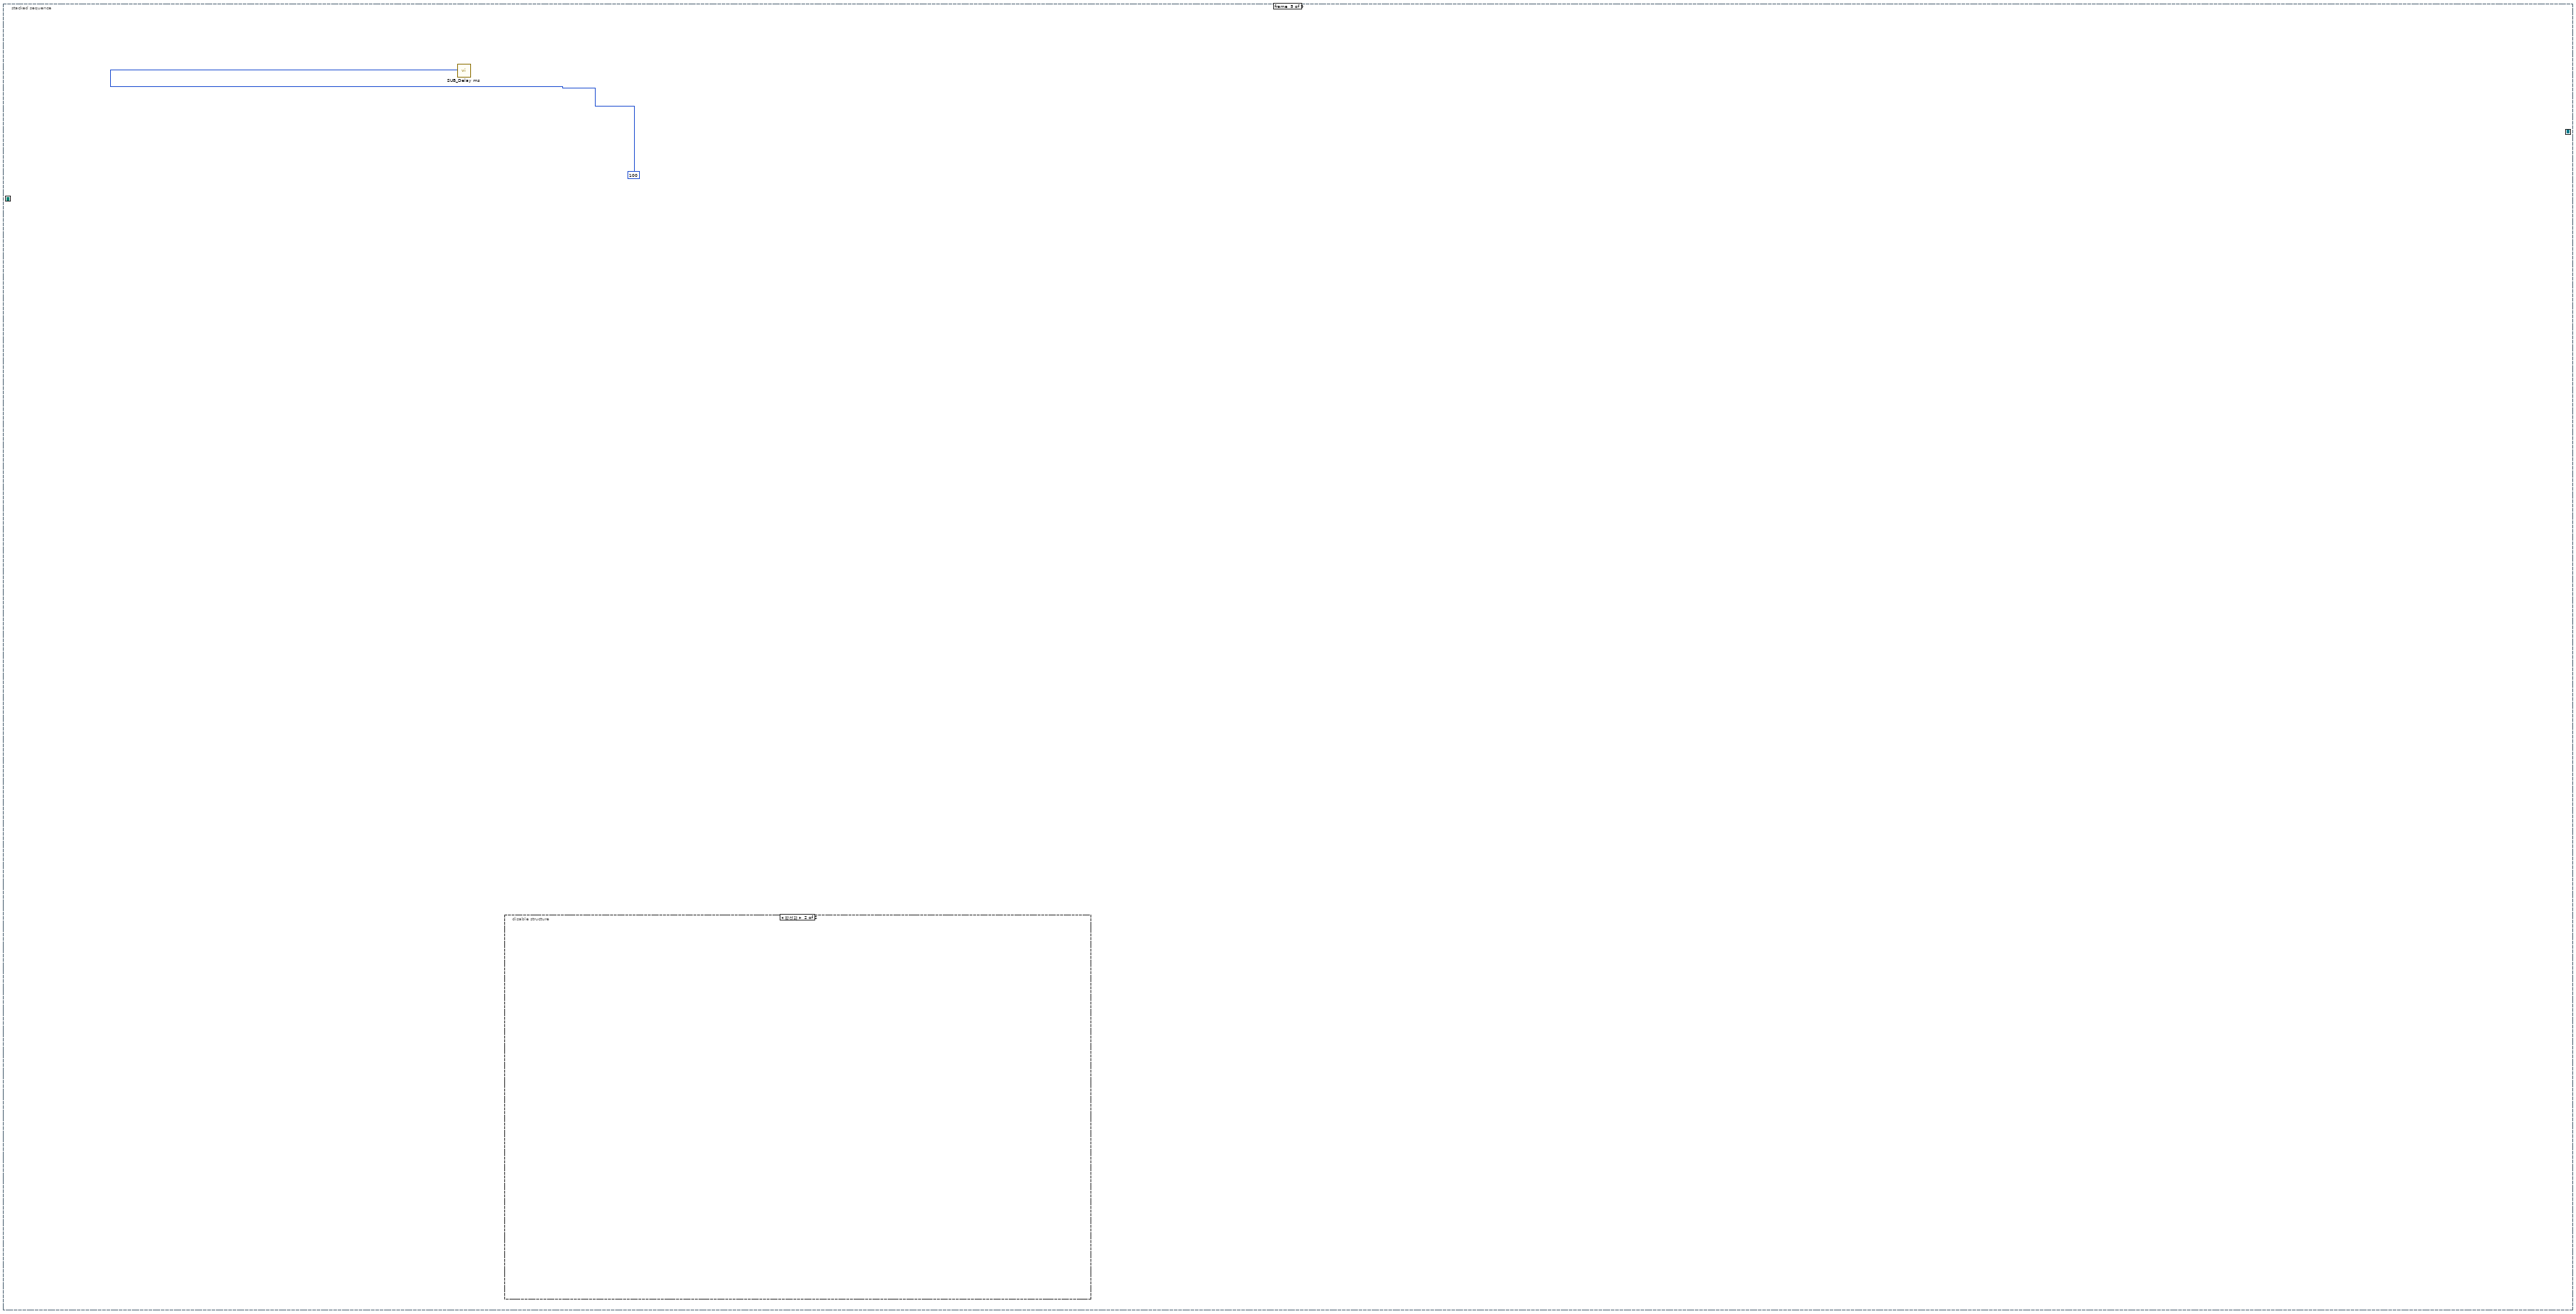
[diagram p10: hidden frame]
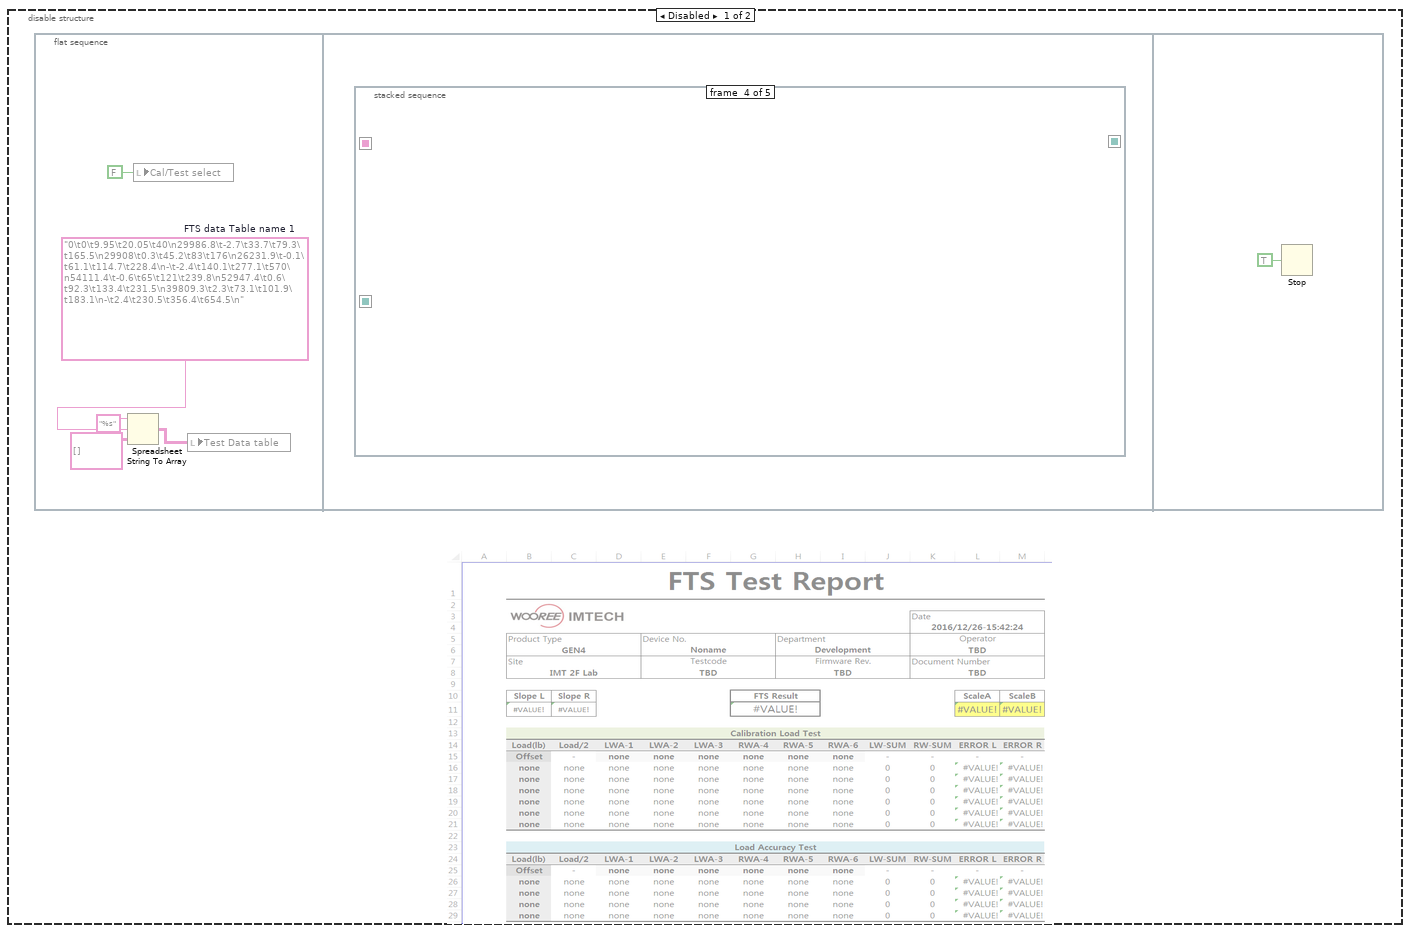
[diagram p11: hidden frame]
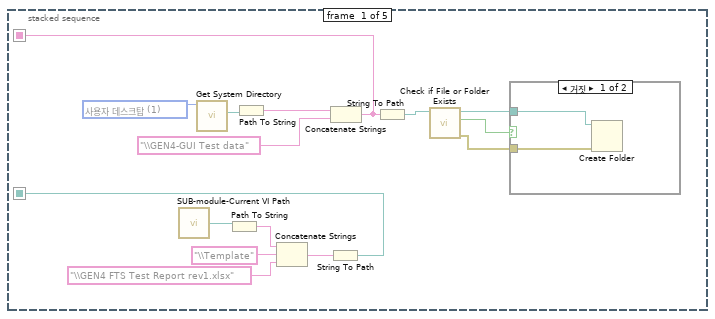
[diagram p12: hidden frame]
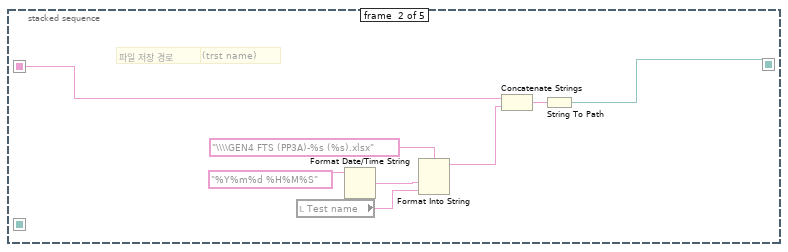
[diagram p14: hidden frame]
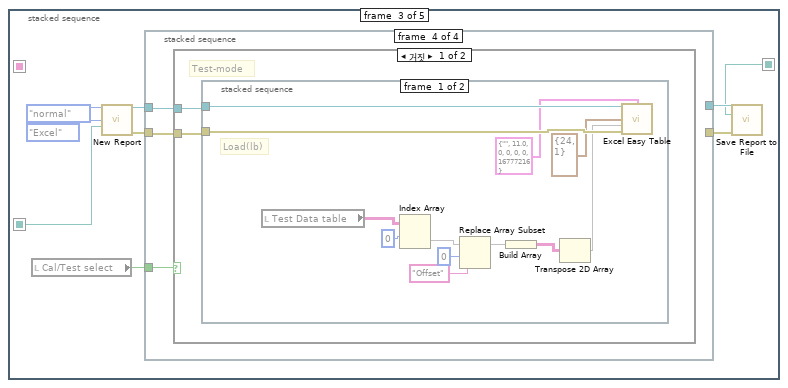
[diagram p15: hidden frame]
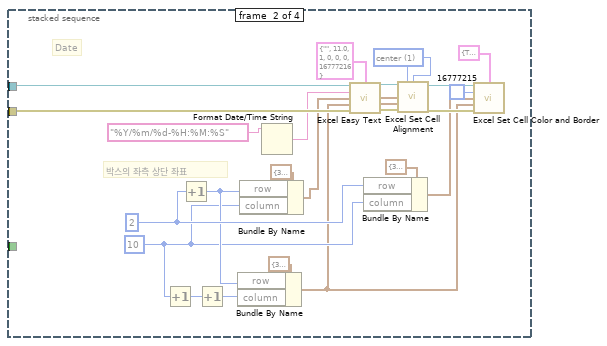
[diagram p17: hidden frame]
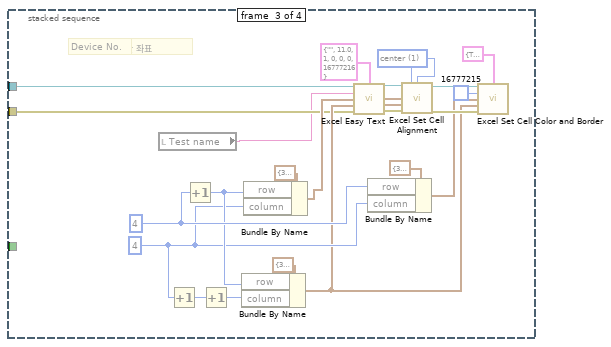
[diagram p18: hidden frame]
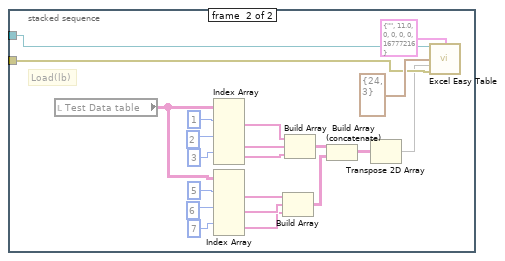
[diagram p19: hidden frame]
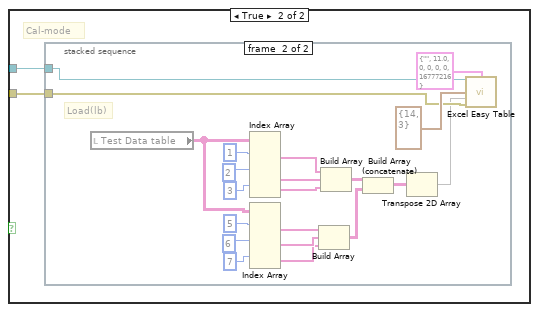
[diagram p20: hidden frame]
diagram:
  n1 = stacked-sequence {
    seq-local: [_ _ _ w167 _ _ _ _ _] -> [_ _ _ _ _ _ _ w2772 _]
    seq-local: [w33 _ _ _ _ _ _ _ _] -> [_ _ _ _ _ _ _ w2768 _]
    frame #0 {
      (unwired) FALSE ("Rx OK")
      # "BLE Buffer Clear"
      # "Local variable"
      n2 = Tick Count (ms)() -> (millisecond timer value=→"ms timer":u32)
      n3 = call "SUB-BLE Rx data Clear.vi"() -> ()  [unwired: 6 in]
      n4 = local write "Status"("" ("문자열")) -> ()
      n5 = control-ref of="탭-Top"() -> (w31:refnum<vi>)
      n6 = control-ref of="Flash Map"() -> (w16:refnum<vi>)
      n7 = local write "Error"(FALSE ("불리언 2")) -> ()
      n8 = local write "log data1"(FALSE ("log data1")) -> ()
      n9 = Tick Count (ms)() -> (millisecond timer value=→"Timer-ble log":u32)
      n10 = local write "battery cal Tx"(FALSE ("불리언 2")) -> ()
      n11 = Build Array(w31, w16) -> (w33:refnum<vi>[])
      n12 = call "Read and Write Controls to Automatic Config File.vi"("Action"=RWC_Actions."Read", "Control References"=w33) -> ()  [unwired: 9 in, 1 out]
      n13 = local write "FTS table index"(0 ("FTS table index")) -> ()
      n14 = local write "Cal/Test select"(TRUE ("Cal select")) -> ()
      n15 = local write "Force Set"(FALSE ("Force Set")) -> ()
      n16 = local write "Load(lb)"(10.0 ("Load(lb)")) -> ()
      n17 = local write "Handle"(u16 16 ("Handle")) -> ()
      n18 = local write "Data(h)"("\u0001þ" ("Data")) -> ()
      n19 = local write "Head Up"(FALSE ("Head Up")) -> ()
      n20 = local write "Data Log"("" ("Data Log")) -> ()
      n21 = local write "Data_mon(h)"("" ("Data_mon")) -> ()
      n22 = property on="Pane" class="Pane"("Origin"=T18 {"Horizontal"=0, "Vertical"=0} ("원점"), "VertScrollbarVisibility"=T17."Off While Running" ("수직 스크롤 막대 보이기")) -> ()  [unwired: 2 in, 2 out]
      "Rx Cnt" <- 0 ("Rx Cnt")
      "Rx buf 1" <- "" ("Rx 문자열 1")
      "Disconnected" <- FALSE ("Disconnected")
      "Packet Detect" <- FALSE ("Packet Detect")
      "log ble buf" <- "" ("log ble buf")
      "battery cal complete boolean" <- FALSE ("불리언 2")
    }
    frame #1 {
      w78 = 1.0 ("Y 스케일.범위:최대값")
      w84 = T11 {"Gyroscope X"=0.0, "Gyroscope Y"=0.0, "Gyroscope Z"=0.0, "Accelerometer X"=0.0, "Accelerometer Y"=0.0, "Accelerometer Z"=0.0} ("IMU data")
      w85 = T10 {"Left Wing-A, C1/C0"=0.0, "Left Wing-B, C2/C0"=0.0, "Left Wing-C, C3/C0"=0.0, "Right Wing-A, C4/C0"=0.0, "Right Wing-B, C5/C0"=0.0, "Right Wing-C, C6/C0"=0.0} ("CDC data")
      w86 = FALSE ("Offset 1")
      # "Variable initialization"
      n23 = local write "Maximize window"(FALSE ("창크게")) -> ()
      n24 = local write "Setting load(led)"(FALSE ("Power On Flag")) -> ()
      n25 = local write "Comm con 1"(FALSE ("포트 연결")) -> ()
      n26 = local write "Comm con status 1"(FALSE ("Connected")) -> ()
      n27 = local write "Data trx(led)"(FALSE ("Rx")) -> ()
      n28 = local write "ACT-Comm"(FALSE ("ACT-RS422")) -> ()
      n29 = local write "Port open 1"(FALSE) -> ()
      n30 = local write "Port close 1"(FALSE) -> ()
      n31 = local write "*Board ID1"("None...." ("*Board ID")) -> ()
      n32 = local write "stop"(FALSE ("stop")) -> ()
      n33 = local write "Comm err cnt 1"(0 ("통신에러카운트")) -> ()
      n34 = local write "Setting load"(TRUE ("설정값 불러오기")) -> ()
      n35 = local write "Rx-mon"(FALSE) -> ()
      n36 = property on="CDC(PCAP02) Graph" class="WFChart (엄격한)"("History Data"=waveform(dbl)[][] [] ("히스토리 데이터")) -> ()  [unwired: 2 in, 2 out]
      n37 = property on="IMU Graph" class="WFChart (엄격한)"("History Data"=waveform(dbl)[][] [] ("히스토리 데이터")) -> ()  [unwired: 2 in, 2 out]
      n38 = local write "status string"("" ("status string")) -> ()
      n39 = Tick Count (ms)() -> (millisecond timer value=w95:u32)
      n40 = Tick Count (ms)() -> (millisecond timer value=w88:u32)
      n41 = Tick Count (ms)() -> (millisecond timer value=w70:u32)
      n42 = Tick Count (ms)() -> (millisecond timer value=w71:u32)
      n43 = Initialize Array(T19 {"RxOK"=FALSE, "ROM Data"=[], "Index"=0} ("클러스터"), 9 ("차원 크기")) -> (w66:T12)
      n44 = local write "Logging No."(u32 0 ("Logging No.")) -> ()
      n45 = local write "RxD"("" ("RxD")) -> ()
      n46 = local write "Offset 1"(w86) -> ()
      n47 = local write "Offset 2"(w86) -> ()
      n48 = local write "Data Logging"(FALSE ("Data Logging")) -> ()
      n49 = local write "Export graph 1"(FALSE ("그래프 반출")) -> ()
      n50 = local write "Full ROM data"(FALSE ("Full ROM data")) -> ()
      n51 = local write "Export graph2"(FALSE ("그래프 반출")) -> ()
      n52 = local write "Graph timer 1"(w95) -> ()
      n53 = local write "Bat(raw)"(0.0 ("Bat(raw)")) -> ()
      n54 = local write "ROM Data"(w66) -> ()
      n55 = local write "Rx-ROM"(FALSE ("Rx-ROM")) -> ()
      n56 = local write "Clear graph 1"(TRUE ("그래프 지우기")) -> ()
      n57 = local write "Graph timer 2"(w88) -> ()
      n58 = local write "ms timer 2"(w70) -> ()
      n59 = local write "ms timer 3"(w71) -> ()
      n60 = local write "Clear graph 2"(TRUE ("그래프 지우기")) -> ()
      n61 = local write "Rx ROM-log"("" ("문자열-Rx ROM")) -> ()
      n62 = local write "CDC Offet"(w85) -> ()
      n63 = local write "CDC data"(w85) -> ()
      n64 = local write "IMU data"(w84) -> ()
      n65 = local write "IMU Offet"(w84) -> ()
      n66 = local write "92 tx"(FALSE ("92 tx")) -> ()
      n67 = Tick Count (ms)() -> (millisecond timer value=w63:u32)
      n68 = local write "Save"(FALSE ("Save")) -> ()
      n69 = local write "BLE Interval Time(ms)"(0.0 ("BLE Interval Time(ms)")) -> ()
      n70 = local write "Test Start"(FALSE ("Test Start")) -> ()
      n71 = local write "94 tx"(FALSE ("94 tx")) -> ()
      n72 = local write "83 tx"(FALSE ("83 tx")) -> ()
      n73 = property on="BLE Interval buf" class="WFChart (엄격한)"("History Data"=u32[] [] ("히스토리 데이터")) -> ()  [unwired: 2 in, 2 out]
      n74 = local write "ms timer 5"(w63) -> ()
      n75 = property on="BLE Interval Graph" class="WFChart (엄격한)"("History Data"=dbl[] [] ("히스토리 데이터")) -> ()  [unwired: 2 in, 2 out]
      n76 = property on="BLE RSSI buf" class="WFChart (엄격한)"("History Data"=i16[] [] ("히스토리 데이터")) -> ()  [unwired: 2 in, 2 out]
      n77 = local write "BLE RSSI (dBm)"(0.0 ("BLE RSSI (dBm)")) -> ()
      n78 = property on="BLE RSSI Graph" class="WFChart (엄격한)"("History Data"=i16[] [] ("히스토리 데이터")) -> ()  [unwired: 2 in, 2 out]
      n79 = local write "98 tx"(FALSE ("98 tx")) -> ()
      n80 = local write "88 tx"(FALSE ("88 tx")) -> ()
      n81 = local write "A1 tx"(FALSE ("A1 tx")) -> ()
      n82 = local write "91 tx"(FALSE ("91 tx")) -> ()
      n83 = local write "A3 tx"(FALSE ("A3 tx")) -> ()
      n84 = for {
        N: 3 -> [_]
        i -> [w116]
        w117 = 125.0 ("Y 스케일.범위:최대값")
        n85 = Multiply(x=w117, y=-1.0 ("Y 스케일.범위:최대값")) -> (x*y=w119:dbl)
        n86 = property on="IMU Graph" class="WFChart (엄격한)"("ActYScl"=w116, "YScale.Maximum"=w117, "YScale.Minimum"=w119, "YScale.ScaleFit"=u8 0 ("Y 스케일.스케일 맞춤")) -> ()  [unwired: 2 in, 2 out]
      }
      n87 = for {
        N: 3 -> [_]
        i -> [w111]
        w112 = 1.1 ("Y 스케일.범위:최대값")
        n88 = Add(x=w111, y=3.0 ("Y 스케일.범위:최대값")) -> (x+y=w109:dbl)
        n89 = Multiply(x=w112, y=-1.0 ("Y 스케일.범위:최대값")) -> (x*y=w114:dbl)
        n90 = property on="IMU Graph" class="WFChart (엄격한)"("ActYScl"=w109, "YScale.Maximum"=w112, "YScale.Minimum"=w114, "YScale.ScaleFit"=u8 0 ("Y 스케일.스케일 맞춤")) -> ()  [unwired: 2 in, 2 out]
      }
      n91 = Multiply(x=w78, y=-1.0 ("Y 스케일.범위:최대값")) -> (x*y=w77:dbl)
      n92 = property on="CDC(PCAP02) Graph" class="WFChart (엄격한)"("YScale.Maximum"=w78, "YScale.Minimum"=w77, "YScale.ScaleFit"=u8 2 ("Y 스케일.스케일 맞춤")) -> ()  [unwired: 2 in, 2 out]
      "second counter Tx" <- FALSE ("불리언 4")
      "Battery cal Rx" <- FALSE ("불리언 5")
      "42 Tx" <- FALSE ("불리언 6")
      "42 Rx" <- FALSE ("불리언 7")
      "Error" <- FALSE ("불리언 4")
      "second counter Rx" <- FALSE ("불리언 4")
      "scale A.B Tx" <- FALSE ("scale A.B Tx")
      "scale A,B Rx" <- FALSE ("scale A,B Rx")
      "FTS 42 Tx" <- FALSE ("불리언 6")
      "FTS 42 Rx" <- FALSE ("불리언 7")
      "FTS device out" <- FALSE ("FTS device out")
      "FTS start" <- FALSE ("FTS start")
    }
    frame #2 {
      w125 = "Serial number\t-\t-\nYEAR\t-\t-\nMonth\t-\t-\nDay\t-\t-\nDevice ID\t-\t-\nManufacturer ID\t-\t-\nCal_Scale A\t-\t-\nCal_Scale B\t-\t-\nCal_Acc. X\t-\t-\nCal_Acc. Y\t-\t-\nCal_Acc. Z\t-\t-\nCal_Gy. X\t-\t-\nCal_Gy. Y\t-\t-\nCal_Gy. Z\t-\t-\nCal_Vol H\t-\t-\nCal_Vol L\t-\t-\nCal_CDC Off 1\t-\t-\nCal_CDC Off 2\t-\t-\nCal_CDC Off 3\t-\t-\nCal_CDC Off 4\t-\t-\nCal_CDC Off 5\t-\t-\nCal_CDC Off 6\t-\t-\nCal_CDC Off 7\t-\t-\nCal_CDC Off 8\t-\t-\nFirmware Revision\t-\t-\nOperative Side\t-\t-\nCal_Compart. A_10\t-\t-\nCal_Compart. B_10\t-\t-\nReserved\t-\t-\nCal_Compart. A_11\t-\t-\nCal_Compart. B_11\t-\t-\nCal_Compart. A_12\t-\t-\nCal_Compart. B_12\t-\t-\nCal_Compart. A_13\t-\t-\nCal_Compart. B_13\t-\t-\nCal_Compart. A_14\t-\t-\nCal_Compart. B_14\t-\t-\nCal_Compart. A_16\t-\t-\nCal_Compart. B_16\t-\t-\nReserved\t-\t-\nAcc. X_0 value\t-\t-\nAcc. Y_0 value\t-\t-\nAcc. Z_0 value\t-\t-\nAcc. X_45 value\t-\t-\nAcc. Y_45 value\t-\t-\nAcc. Z_45 value\t-\t-\nReserved\t-\t-\nAcc. X_90 value\t-\t-\nAcc. Y_90 value\t-\t-\nAcc. Z_90 value\t-\t-\nAcc. X_180 value\t-\t-\nAcc. Y_180 value\t-\t-\nAcc. Z_180 value\t-\t-\nSecond counter\t-\t-\nReserved\t-\t-\n\n\n\n\n\n\n\n\n\n\n\n\n\n\n\n"  # ROM Table-row header
      w132 = "1\n2\n3\n4\n5\n6\n7\n8\n9\n10\n11\n12\n13\n14\n15\n16\n17\n18\n19\n20\n21\n22\n23\n24\n25\n26\n27\n28\n29\n30\n31\n32\n33\n34\n35\n36\n37\n38\n39\n40\n41\n42\n43\n44\n45\n46\n47\n48\n49\n50\n51\n52\n53\n54\n55\n56\n57"  # ROM Table-row index
      w136 = "Name\nValue\nDescriptions"  # ROM Table-col header
      w139 = "Load(1)-0lb\t0\t1000\t0\t0\nInit(1)-70lb\t70\t1000\t0\t0\nInit(2)-140lb\t140\t1000\t0\t0\nInit(1)-70lb\t70\t1000\t0\t0\nInit(2)-140lb\t140\t1000\t0\t0\nLoad(1)-0lb\t0\t10000\t1\t1\nLoad(2)-10lb\t10\t3000\t0\t1\nLoad(3)-20lb\t20\t3000\t0\t1\nLoad(4)-40lb\t40\t3000\t0\t1\nLoad(5)-60lb\t60\t3000\t0\t1\nLoad(6)-80lb\t80\t3000\t0\t1"  # FTS Profile 1
      w144 = "Offset\nLoad(1)-0lb\nLoad(2)-10lb\nLoad(3)-20lb\nLoad(4)-40lb\nLoad(5)-60lb\nLoad(6)-80lb"  # FTS data Table name 1
      # "FTS Profile Init\n(Name, Press, Time)"
      # "col"
      # "Variable initialization"
      n93 = for {
        N: 9 -> [_]
        tunnel: [w155] -> w146 mode=indexing
        # "row"
        n94 = for {
          N: 10 -> [_]
          tunnel: ["-"] -> w155 mode=indexing
        }
      }
      n95 = control-ref of="File path"() -> (w123:refnum<vi>)
      n96 = call <vilib>:"Application Directory.vi"() -> ("Application Directory"=w122:path)
      n97 = local write "Mark10 Gauge (lb)"(0.0 ("Mark10 Gauge")) -> ()
      n98 = local write "FTS comm."(FALSE ("FTS 수신 정상")) -> ()
      n99 = local write "Test name"("Noname" ("Test name")) -> ()
      n100 = local write "FTS Testing"(FALSE ("FTS 시험 진행")) -> ()
      n101 = property class="Path"(reference=w123, "Value"=w122) -> ()  [unwired: 1 in, 2 out]
      n102 = local write "FTS OP status"(T8 "Test_Start" ("FTS OP status")) -> ()
      n103 = local write "Test Status"("" ("Force Test Status")) -> ()
      n104 = for {
        N: 7 -> [_]
        i -> [w159]
        n105 = Bundle By Name(cluster=T20 {"Row"=0, "Column"=0} ("활성 셀:활성 셀"), "Row"=0, "Column"=w159) -> (w161:T20)
        n106 = property on="Test Data table" class="Tbl (엄격한)"("Active Cell"=w161, "Width"=u32 80 ("활성 셀:셀 크기:폭")) -> ()  [unwired: 2 in, 2 out]
      }
      n107 = call "SUB-module-StringToArray.vi"("String"="Mark10 Gauge(lb)\nLeft Wing-A\nLeft Wing-B\nLeft Wing-C\nLeft Wing-SUM\nRight Wing-A\nRight Wing-B\nRight Wing-C\nRight Wing-SUM" ("문자열")) -> ("Arrary"=w141:string[])
      n108 = local write "Load Graph"(cluster{dbl[], dbl[]} {[], []} ("Load Graph")) -> ()
      n109 = local write "Test Data table"(w146) -> ()
      n110 = property on="Test Data table" class="Tbl (엄격한)"("Row Headers[]"=w141) -> ()  [unwired: 2 in, 2 out]
      n111 = Generate Occurrence() -> (→"Disconnection ocurrence":refnum<k4>)
      n112 = call "SUB-module-StringToArray.vi"("String"=w144) -> ("Arrary"=w143:string[])
      n113 = Spreadsheet String To Array(format string="%s" ("포맷 문자열"), spreadsheet string=w139, array type (2D Dbl)=string[][] [] ("배열 타입(2D Dbl)")) -> (array=w150:string[][])  [unwired: 1 in]
      n114 = Spreadsheet String To Array(format string="%s" ("포맷 문자열"), spreadsheet string=w125, array type (2D Dbl)=string[][] [] ("배열 타입(2D Dbl)")) -> (array=w126:string[][])  [unwired: 1 in]
      n115 = property on="Test Data table" class="Tbl (엄격한)"("Column Headers[]"=w143) -> ()  [unwired: 2 in, 2 out]
      n116 = Spreadsheet String To Array(delimiter (Tab)="\n", format string="%s" ("포맷 문자열"), spreadsheet string=w132, array type (2D Dbl)=string[] [] ("배열 타입(2D Dbl)")) -> (array=w131:string[])
      n117 = local write "Test profile"(w150) -> ()
      n118 = Spreadsheet String To Array(delimiter (Tab)="\n", format string="%s" ("포맷 문자열"), spreadsheet string=w136, array type (2D Dbl)=string[] [] ("배열 타입(2D Dbl)")) -> (array=w135:string[])
      n119 = property on="ROM Table" class="Tbl (엄격한)"("Column Headers[]"=w135, "Row Headers[]"=w131, "Value"=w126) -> ()  [unwired: 2 in, 2 out]
      n120 = invoke on="ROM Table" class="Tbl (엄격한)" method="Reinit To Default"() -> ()  [unwired: 3 in, 3 out]
    }
    frame #3 {
      # "Program configration is loaded from file."
      n121 = call "SUB-module-Current VI Path.vi"() -> ("현재 VI 경로"=w168:path)
      n122 = Path To String(path=w168) -> (string=w170:string)
      n123 = Concatenate Strings(w170, "\\Configuration File.ini") -> (w169:string)
      n124 = String To Path(string=w169) -> (path=w167:path)
      n125 = call <vilib>:"Open Config Data.vi"("create file if necessary (T)"=TRUE, "configuration file path"=w167) -> ("error out"=w174:errorcluster, "refnum"=w173:T32)  [unwired: 7 in, 1 out]
      n126 = stacked-sequence {
        tunnel: w173 -> [w181 w183 w189 w196 w201]
        tunnel: w174 -> [w180 w182 w188 w195 w200]
        tunnel: "GUI Setting" ("section") -> [w179 w184 w190 w197 _]
        tunnel: [_ _ _ _ w201] -> w165
        tunnel: [_ _ _ _ w200] -> w164
        frame #0 {
          w178 = "Com Port-Board1"  # Key 1
          n127 = call-poly <vilib>:"Read Key.vi"("section"=w179, "error in (no error)"=w180, "default value"="COM4" ("output string"), "key"=w178, "refnum"=w181) -> ("value"=w177:string)  [unwired: 3 in, 3 out]
          n128 = local write "Port-set 1"(w177) -> ()
        }
        frame #1 {
          w187 = "Com Port-FTS"  # Key 1
          n129 = call-poly <vilib>:"Read Key.vi"("section"=w184, "error in (no error)"=w182, "default value"="COM5" ("output string"), "key"=w187, "refnum"=w183) -> ("value"=w186:string)  [unwired: 3 in, 3 out]
          n130 = local write "Port-FTS"(w186) -> ()
        }
        frame #2 {
          w193 = "Logno"  # Key 1
          n131 = call-poly <vilib>:"Read Key.vi"("section"=w190, "error in (no error)"=w188, "default value"="1" ("output string"), "key"=w193, "refnum"=w189) -> ("value"=w192:string)  [unwired: 3 in, 3 out]
          n132 = local write "Log no"(w192) -> ()
        }
        frame #3 {
          w199 = "Interval(ms)"  # Key 1
          n133 = call-poly <vilib>:"Read Key.vi"("section"=w197, "error in (no error)"=w195, "default value"=100, "key"=w199, "refnum"=w196) -> ("value"=w198:i32)  [unwired: 3 in, 3 out]
          n134 = local write "Update(ms)"(w198) -> ()
        }
        frame #4 {
        }
      }
      n135 = local write "status string"("Program settings Loading..." ("status string")) -> ()
      n136 = call <vilib>:"Close Config Data.vi"("error in (no error)"=w164, "write file if changed (T)"=FALSE ("write configuration file? (T)"), "refnum"=w165) -> ()  [unwired: 9 out]
    }
    frame #4 {
      n137 = call "SUB_Delay ms.vi"("delay(ms)"=u32 100 ("ms 타이머 값")) -> ()  [unwired: 3 in]
      n138 = disable-structure shown="활성화" {
        frame Disabled {
          n139 = flat-sequence {
            frame #0 {
              w205 = "0\t0\t9.95\t20.05\t40\n29986.8\t-2.7\t33.7\t79.3\t165.5\n29908\t0.3\t45.2\t83\t176\n26231.9\t-0.1\t61.1\t114.7\t228.4\n-\t-2.4\t140.1\t277.1\t570\n54111.4\t-0.6\t65\t121\t239.8\n52947.4\t0.6\t92.3\t133.4\t231.5\n39809.3\t2.3\t73.1\t101.9\t183.1\n-\t2.4\t230.5\t356.4\t654.5\n"  # FTS data Table name 1
              n140 = Spreadsheet String To Array(format string="%s" ("포맷 문자열"), spreadsheet string=w205, array type (2D Dbl)=string[][] [] ("배열 타입(2D Dbl)")) -> (array=w204:string[][])  [unwired: 1 in]
              n141 = local write "Cal/Test select"(FALSE ("Cal/Test select")) -> ()
              n142 = local write "Test Data table"(w204) -> ()
            }
            frame #1 {
              n143 = stacked-sequence {
                seq-local: [_ w226 _ _ _] -> [_ _ w235 _ _]
                seq-local: [w214 _ _ _ _] -> [_ w225 _ _ _]
                seq-local: [w208 _ _ _ _] -> [_ _ w234 _ _]
                frame #0 {
                  w222 = T33 1 items=["사용자 홈"=0, "사용자 데스크탑"=1, "사용자 문서"=2, "사용자 어플리케이션 데이터"=3, "사용자 환경"=4, "사용자 임시"=5, "퍼블릭 문서"=6, "퍼블릭 어플리케이션 데이터"=7, "퍼블릭 환경"=8, "퍼블릭 캐시"=13, "시스템 코어 라이브러리"=9, "시스템 설치된 라이브러리"=10, "어플리케이션 파일"=11, "부팅 볼륨 루트"=12] ("system directory type")
                  n144 = call "SUB-module-Current VI Path.vi"() -> ("현재 VI 경로"=w211:path)
                  n145 = call <vilib>:"Get System Directory.vi"("system directory type"=w222) -> ("system directory"=w221:path)  [unwired: 10 in]
                  n146 = Path To String(path=w211) -> (string=w210:string)
                  n147 = Path To String(path=w221) -> (string=w220:string)
                  n148 = Concatenate Strings(w210, "\\Template" ("이름 또는 상대 경로"), "\\GEN4 FTS Test Report rev1.xlsx" ("이름 또는 상대 경로")) -> (w209:string)
                  n149 = String To Path(string=w209) -> (path=w208:path)
                  n150 = Concatenate Strings(w220, "\\GEN4-GUI Test data" ("상태")) -> (w214:string)
                  n151 = String To Path(string=w214) -> (path=w218:path)
                  n152 = call <vilib>:"Check if File or Folder Exists.vi"("path"=w218) -> ("error out"=w215:errorcluster, "file or folder exists?"=w217:bool, "dup path"=w216:path)  [unwired: 8 in]
                  n153 = case shown="거짓" w217 {
                    tunnel: w216 -> [w224 _]
                    tunnel: w215 -> [w223 _]
                    frame False {
                      n154 = Create Folder(path (use dialog)=w224, error in=w223) -> ()  [unwired: 1 in, 3 out]
                    }
                    frame True {
                    }
                  }
                }
                frame #1 {
                  # "* 파일명(rev)-date (trst name)"
                  # "파일 저장 경로"
                  n155 = local read "Test name"() -> (w231:string)
                  n156 = Format Date/Time String(time format string (%c)="%Y%m%d %H%M%S" ("상태")) -> (date/time string=w230:string)  [unwired: 2 in]
                  n157 = Format Into String(format string="\\\\GEN4 FTS (PP3A)-%s (%s).xlsx" ("상태"), w230, w231) -> (resulting string=w227:string)  [unwired: 2 in, 1 out]
                  n158 = Concatenate Strings(w225, w227) -> (w232:string)
                  n159 = String To Path(string=w232) -> (path=w226:path)
                }
                frame #2 {
                  n160 = local read "Cal/Test select"() -> (w233:bool)
                  n161 = call <vilib>:"New Report.vi"("window state (normal)"=T22."normal", "report type"=T21."Excel", "template (empty)"=w234) -> ("report out"=w238:refnum<class "NI_report.lvclass">, "error out"=w239:errorcluster)  [unwired: 11 in]
                  n162 = stacked-sequence {
                    tunnel: w238 -> [w243 w268 w270 w295]
                    tunnel: w239 -> [w242 w267 w271 w294]
                    tunnel: [w243 _ _ _] -> w241
                    tunnel: [w242 _ _ _] -> w240
                    tunnel: w233 -> [_ _ _ w293]
                    frame #0 {
                    }
                    frame #1 {
                      w246 = 10 ("column")
                      w253 = 2 ("row")
                      w260 = 1 items=["top", "center", "bottom"] ("vertical alignment (top)")
                      # "Date"
                      # "박스의 좌측 상단 좌표"
                      n163 = Increment(x=w246) -> (x+1=w245:i32)
                      n164 = Increment(x=w253) -> (x+1=w248:i32)
                      n165 = Increment(x=w245) -> (x+1=w247:i32)
                      n166 = Bundle By Name(cluster=cluster{"row":i32, "column":i32} {"row"=3, "column"=10} ("start (-1, -1)"), "row"=w248, "column"=w247) -> (w244:cluster{"row":i32, "column":i32})
                      n167 = Bundle By Name(cluster=cluster{"row":i32, "column":i32} {"row"=3, "column"=10} ("start (-1, -1)"), "row"=w248, "column"=w246) -> (w254:cluster{"row":i32, "column":i32})
                      n168 = Format Date/Time String(time format string (%c)="%Y/%m/%d-%H:%M:%S" ("상태")) -> (date/time string=w266:string)  [unwired: 2 in]
                      n169 = call <vilib>:"Excel Easy Text.vi"("report in"=w268, "font"=T23 {"font name"="", "font size"=11.0, "bold"=1, "italic"=0, "underline"=0, "strike through"=0, "font color"=16777216}, "text"=w266, "start (-1, -1)"=w254, "end (-1, -1)"=w244, "error in (no error)"=w267) -> ("report out"=w264:refnum<class "NI_report.lvclass">, "next cell bottom-left"=w262:cluster{"row":i32, "column":i32}, "next cell top-right"=w261:cluster{"row":i32, "column":i32}, "error out"=w263:errorcluster)  [unwired: 5 in, 1 out]
                      n170 = Bundle By Name(cluster=cluster{"row":i32, "column":i32} {"row"=3, "column"=10} ("start (-1, -1)"), "row"=w253, "column"=w246) -> (w252:cluster{"row":i32, "column":i32})
                      n171 = call <vilib>:"Excel Set Cell Alignment.vi"("report in"=w264, "vertical alignment (top)"=w260, "horizontal alignment (left)"=w260, "start (-1, -1)"=w262, "end (-1, -1)"=w261, "error in (no error)"=w263) -> ("report out"=w259:refnum<class "NI_report.lvclass">, "error out"=w258:errorcluster)  [unwired: 8 in]
                      n172 = call <vilib>:"Excel Set Cell Color and Border.vi"("report in"=w259, "outside border"=T24 {"on/off"=TRUE, "weight"=2, "color"=0}, "background color (w)"=u32 16777215, "start (-1, -1)"=w252, "end (-1, -1)"=w244, "error in (no error)"=w258) -> ()  [unwired: 8 in, 2 out]
                    }
                    frame #2 {
                      w274 = 4 ("column")
                      w281 = 4 ("row")
                      w288 = 1 items=["top", "center", "bottom"] ("vertical alignment (top)")
                      # "Device No."
                      # "박스의 좌측 상단 좌표"
                      n173 = local read "Test name"() -> (w269:string)
                      n174 = Increment(x=w274) -> (x+1=w273:i32)
                      n175 = Increment(x=w281) -> (x+1=w276:i32)
                      n176 = Increment(x=w273) -> (x+1=w275:i32)
                      n177 = Bundle By Name(cluster=cluster{"row":i32, "column":i32} {"row"=3, "column"=10} ("start (-1, -1)"), "row"=w276, "column"=w275) -> (w272:cluster{"row":i32, "column":i32})
                      n178 = Bundle By Name(cluster=cluster{"row":i32, "column":i32} {"row"=3, "column"=10} ("start (-1, -1)"), "row"=w276, "column"=w274) -> (w282:cluster{"row":i32, "column":i32})
                      n179 = call <vilib>:"Excel Easy Text.vi"("report in"=w270, "font"=T23 {"font name"="", "font size"=11.0, "bold"=1, "italic"=0, "underline"=0, "strike through"=0, "font color"=16777216}, "text"=w269, "start (-1, -1)"=w282, "end (-1, -1)"=w272, "error in (no error)"=w271) -> ("report out"=w292:refnum<class "NI_report.lvclass">, "next cell bottom-left"=w290:cluster{"row":i32, "column":i32}, "next cell top-right"=w289:cluster{"row":i32, "column":i32}, "error out"=w291:errorcluster)  [unwired: 5 in, 1 out]
                      n180 = Bundle By Name(cluster=cluster{"row":i32, "column":i32} {"row"=3, "column"=10} ("start (-1, -1)"), "row"=w281, "column"=w274) -> (w280:cluster{"row":i32, "column":i32})
                      n181 = call <vilib>:"Excel Set Cell Alignment.vi"("report in"=w292, "vertical alignment (top)"=w288, "horizontal alignment (left)"=w288, "start (-1, -1)"=w290, "end (-1, -1)"=w289, "error in (no error)"=w291) -> ("report out"=w287:refnum<class "NI_report.lvclass">, "error out"=w286:errorcluster)  [unwired: 8 in]
                      n182 = call <vilib>:"Excel Set Cell Color and Border.vi"("report in"=w287, "outside border"=T24 {"on/off"=TRUE, "weight"=2, "color"=0}, "background color (w)"=u32 16777215, "start (-1, -1)"=w280, "end (-1, -1)"=w272, "error in (no error)"=w286) -> ()  [unwired: 8 in, 2 out]
                    }
                    frame #3 {
                      n183 = case shown="거짓" w293 {
                        tunnel: w295 -> [w297 w332]
                        tunnel: w294 -> [w296 w331]
                        frame False {
                          # "Test-mode"
                          n184 = stacked-sequence {
                            tunnel: w297 -> [w309 w328]
                            tunnel: w296 -> [w308 w327]
                            frame #0 {
                              # "Load(lb)"
                              n185 = local read "Test Data table"() -> (w307:string[][])
                              n186 = Index Array(array=w307, index (row)=0 ("인덱스 (행)")) -> (element=w304:string[])  [unwired: 1 in]
                              n187 = Replace Array Subset(array=w304, new element="Offset" ("새 원소/부분배열"), index=0 ("인덱스")) -> (w301:string[])
                              n188 = Build Array(w301) -> (w300:string[][])
                              n189 = Transpose 2D Array(2D array=w300) -> (transposed array=w299:string[][])
                              n190 = call-poly <vilib>:"Excel Easy Table.vi"("report in"=w309, "font"=T23 {"font name"="", "font size"=11.0, "bold"=0, "italic"=0, "underline"=0, "strike through"=0, "font color"=16777216}, "start (0, 0)"=cluster{"row":i32, "column":i32} {"row"=24, "column"=1}, "text data"=w299, "error in (no error)"=w308) -> ()  [unwired: 6 in, 5 out]
                            }
                            frame #1 {
                              # "Load(lb)"
                              n191 = local read "Test Data table"() -> (w321:string[][])
                              n192 = Index Array(array=w321, index (row) #1=1 ("인덱스 (행)"), index (row) #2=2 ("인덱스 (행)"), index (row) #3=3 ("인덱스 (행)")) -> (element #1=w320:string[], element #2=w319:string[], element #3=w318:string[])  [unwired: 3 in]
                              n193 = Index Array(array=w321, index (row) #1=5 ("인덱스 (행)"), index (row) #2=6 ("인덱스 (행)"), index (row) #3=7 ("인덱스 (행)")) -> (element #1=w317:string[], element #2=w316:string[], element #3=w315:string[])  [unwired: 3 in]
                              n194 = Build Array(w317, w316, w315) -> (w313:string[][])
                              n195 = Build Array(w320, w319, w318) -> (w314:string[][])
                              n196 = Build Array (concatenate)(w314, w313) -> (w312:string[][])
                              n197 = Transpose 2D Array(2D array=w312) -> (transposed array=w311:string[][])
                              n198 = call-poly <vilib>:"Excel Easy Table.vi"("report in"=w328, "font"=T23 {"font name"="", "font size"=11.0, "bold"=0, "italic"=0, "underline"=0, "strike through"=0, "font color"=16777216}, "start (0, 0)"=cluster{"row":i32, "column":i32} {"row"=24, "column"=3}, "text data"=w311, "error in (no error)"=w327) -> ()  [unwired: 6 in, 5 out]
                            }
                          }
                        }
                        frame True {
                          # "Cal-mode"
                          n199 = stacked-sequence {
                            tunnel: w332 -> [w344 w363]
                            tunnel: w331 -> [w343 w362]
                            frame #0 {
                              # "Load(lb)"
                              n200 = local read "Test Data table"() -> (w342:string[][])
                              n201 = Index Array(array=w342, index (row)=0 ("인덱스 (행)")) -> (element=w339:string[])  [unwired: 1 in]
                              n202 = Replace Array Subset(array=w339, new element="Offset" ("새 원소/부분배열"), index=0 ("인덱스")) -> (w336:string[])
                              n203 = Build Array(w336) -> (w335:string[][])
                              n204 = Transpose 2D Array(2D array=w335) -> (transposed array=w334:string[][])
                              n205 = call-poly <vilib>:"Excel Easy Table.vi"("report in"=w344, "font"=T23 {"font name"="", "font size"=11.0, "bold"=0, "italic"=0, "underline"=0, "strike through"=0, "font color"=16777216}, "start (0, 0)"=cluster{"row":i32, "column":i32} {"row"=14, "column"=1}, "text data"=w334, "error in (no error)"=w343) -> ()  [unwired: 6 in, 5 out]
                            }
                            frame #1 {
                              # "Load(lb)"
                              n206 = local read "Test Data table"() -> (w356:string[][])
                              n207 = Index Array(array=w356, index (row) #1=1 ("인덱스 (행)"), index (row) #2=2 ("인덱스 (행)"), index (row) #3=3 ("인덱스 (행)")) -> (element #1=w355:string[], element #2=w354:string[], element #3=w353:string[])  [unwired: 3 in]
                              n208 = Index Array(array=w356, index (row) #1=5 ("인덱스 (행)"), index (row) #2=6 ("인덱스 (행)"), index (row) #3=7 ("인덱스 (행)")) -> (element #1=w352:string[], element #2=w351:string[], element #3=w350:string[])  [unwired: 3 in]
                              n209 = Build Array(w352, w351, w350) -> (w348:string[][])
                              n210 = Build Array(w355, w354, w353) -> (w349:string[][])
                              n211 = Build Array (concatenate)(w349, w348) -> (w347:string[][])
                              n212 = Transpose 2D Array(2D array=w347) -> (transposed array=w346:string[][])
                              n213 = call-poly <vilib>:"Excel Easy Table.vi"("report in"=w363, "font"=T23 {"font name"="", "font size"=11.0, "bold"=0, "italic"=0, "underline"=0, "strike through"=0, "font color"=16777216}, "start (0, 0)"=cluster{"row":i32, "column":i32} {"row"=14, "column"=3}, "text data"=w346, "error in (no error)"=w362) -> ()  [unwired: 6 in, 5 out]
                            }
                          }
                        }
                      }
                    }
                  }
                  n214 = call-dynamic "Save Report to File.vi"("report in"=w241, "report file path"=w235, "error in (no error)"=w240) -> ()  [unwired: 11 in, 2 out]
                }
                frame #3 {
                }
                frame #4 {
                }
              }
            }
            frame #2 {
              n215 = Stop(stop? (T)=TRUE ("정지? (참)")) -> ()
            }
          }
        }
        frame Enabled {
        }
      }
    }
    frame #5 {
      # "Main Loop"
      n216 = local read "Disconnection ocurrence"() -> (w367:refnum<k4>)
      n217 = while {
        tunnel: w367 -> [w370]
        stop <- w368 stop-if-true
        # "Auto Reconneciton"
        n218 = Wait on Occurrence(2:w370) -> (0:w369:bool)  [unwired: 2 in]
        n219 = stacked-sequence {
          seq-local: [w371 _] -> [_ w377]
          tunnel: w369 -> [_ _]
          tunnel: [_ w377] -> w368
          frame #0 {
            n220 = local read "stop"() -> (w371:bool)
            n221 = case shown="참" w371 {
              frame False {
                n222 = Wait (ms)(milliseconds to wait=u32 100 ("대기 시간(ms)")) -> ()  [unwired: 1 out]
                n223 = call "SUB-Text_Blink.vi"("Timeout"=3.0, "text color"=u32 16711680, "Message"="\nDisconnected") -> ()  [unwired: 9 in]
              }
              frame True {
              }
            }
          }
          frame #1 {
            n224 = Or(x="PWR OFF", y=w377) -> (x .or. y?=w378:bool)
            n225 = case shown="거짓" w378 {
              frame False {
                n226 = control-ref of="Connection Status"() -> (w387:refnum<vi>)
                n227 = property class="Clust (엄격한)"(reference=w387) -> ("Value"=w386:T6)  [unwired: 1 in, 2 out]
                n228 = Unbundle By Name(w386) -> ("MAC Address"=w384:string, "Address Type"=w383:T7)
                n229 = local read "Port-act 1"() -> (w385:refnum<visa-resource-name>)
                n230 = call "BLED1112_auto-connection.vi"("COM Bluegiga in"=w385, "MAC Address"=w384, "Address Type"=w383) -> ("Connection Ok"=w382:bool, "Device Name"=w380:string, "Connection Status"=w379:T6)  [unwired: 7 in, 3 out]
                n231 = Not(x=w382) -> (.not. x?=w381:bool)
                n232 = local write "Rx-mon"(w381) -> ()
                n233 = case shown="참" w381 {
                  tunnel: w380 -> [_ w394]
                  tunnel: w379 -> [_ w393]
                  frame True {
                    # "Received data error status"
                    n234 = local read "Port-act 1"() -> (w391:refnum<visa-resource-name>)
                    n235 = VISA Close(VISA resource name=w391) -> ()  [unwired: 1 in, 1 out]
                    n236 = local write "Comm con status 1"(FALSE ("Connected")) -> ()
                    n237 = local write "*Board ID1"("None...." ("*Board ID")) -> ()
                    n238 = local write "Comm con 1"(FALSE ("보드 통신 연결 1")) -> ()
                    n239 = local write "Rx-mon"(TRUE ("수신 실패(T) 2")) -> ()
                  }
                  frame False {
                    n240 = local write "Connection Status"(w393) -> ()
                    n241 = local write "Device Name"(w394) -> ()
                    n242 = stacked-sequence {
                      frame #0 {
                        # "BLE 버퍼 클리어"
                        n243 = call "SUB-BLE Rx data Clear.vi"() -> ()  [unwired: 6 in]
                        n244 = Wait Until Next ms Multiple(millisecond multiple=u32 200 ("ms 타이머 값")) -> ()  [unwired: 1 out]
                      }
                      frame #1 {
                        n245 = local write "Comm con status 1"(TRUE ("Connected")) -> ()
                      }
                    }
                    n246 = local write "*Board ID1"("" ("*Board ID")) -> ()
                    n247 = local write "Setting load(led)"(FALSE ("Power On Flag")) -> ()
                    n248 = local write "Comm err cnt 1"(0 ("통신에러카운트")) -> ()
                    n249 = local write "Clear graph 1"(FALSE ("그래프 지우기")) -> ()
                    n250 = local write "Clear graph 2"(FALSE ("그래프 지우기")) -> ()
                    n251 = local write "Comm con 1"(TRUE ("포트 연결")) -> ()
                    n252 = local write "RxD"("Connection. OK....." ("status string")) -> ()
                    n253 = disable-structure shown="비활성화" {
                      frame Disabled {
                        w405 = T10 {"Left Wing-A, C1/C0"=0.0, "Left Wing-B, C2/C0"=0.0, "Left Wing-C, C3/C0"=0.0, "Right Wing-A, C4/C0"=0.0, "Right Wing-B, C5/C0"=0.0, "Right Wing-C, C6/C0"=0.0} ("CDC data")
                        w404 = T11 {"Gyroscope X"=0.0, "Gyroscope Y"=0.0, "Gyroscope Z"=0.0, "Accelerometer X"=0.0, "Accelerometer Y"=0.0, "Accelerometer Z"=0.0} ("IMU data")
                        n254 = local write "Data Log"("" ("Data Log")) -> ()
                        n255 = local write "Data_mon(h)"("" ("Data_mon")) -> ()
                        n256 = local write "CDC Offet"(w405) -> ()
                        n257 = local write "CDC data"(w405) -> ()
                        n258 = local write "IMU data"(w404) -> ()
                        n259 = local write "IMU Offet"(w404) -> ()
                      }
                      frame Enabled {
                      }
                    }
                  }
                }
              }
              frame True {
                n260 = control-ref of="PWR OFF"() -> (w408:refnum<vi>)
                n261 = property class="Bool (엄격한)"(reference=w408, "Value"=FALSE ("값(신호)")) -> ()  [unwired: 1 in, 2 out]
                n262 = disable-structure shown="비활성화" {
                  frame Disabled {
                    n263 = control-ref of="Comm con 1"() -> (w410:refnum<vi>)
                    n264 = property class="Bool (엄격한)"(reference=w410, "Val(Sgnl)"=FALSE ("값(신호)")) -> ()  [unwired: 1 in, 2 out]
                  }
                  frame Enabled {
                  }
                }
              }
            }
          }
        }
      }
      n265 = while {
        stop <- w414 stop-if-true
        # "BLE RxD handle"
        n266 = local read "Comm con status 1"() -> (w413:bool)
        n267 = local read "Port-act 1"() -> (w412:refnum<visa-resource-name>)
        n268 = case shown="참" w413 {
          tunnel: w412 -> [_ w419]
          frame False {
          }
          frame True {
            n269 = property class="Instr"(reference=w419) -> (reference out=w418:refnum<visa-resource-name>, error out=w417:errorcluster, "Serial Settings:Number of Bytes at Serial Port"=w416:u32)  [unwired: 1 in]
            n270 = case shown="0, 기본" w416 {
              tunnel: w418 -> [_ w788]
              tunnel: w417 -> [_ w787]
              frame 0, Default {
                # "91 tx"
                # "88 tx"
                # "A3 tx"
                # "A1 tx"
                # "98 tx"
                # "94 tx"
                # "92 tx"
                # "83 tx"
                # "81 tx"
                # "BLE Tx sender"
                n271 = local read "second counter Tx"() -> (w469:bool)
                n272 = local read "scale A.B Tx"() -> (w432:bool)
                n273 = global read "global 3.vi" "배열"() -> (w459:u8[])
                n274 = local read "42 Tx"() -> (w458:bool)
                n275 = local read "Comm con status 1"() -> (w428:bool)
                n276 = And(x=w469, y=w428) -> (x .and. y?=w468:bool)
                n277 = And(x=w432, y=w428) -> (x .and. y?=w431:bool)
                n278 = And(x="battery cal Tx", y=w428) -> (x .and. y?=w474:bool)
                n279 = And(x=w458, y=w428) -> (x .and. y?=w457:bool)
                n280 = local read "FTS 42 Tx"() -> (w429:bool)
                n281 = Index Array(array=w459, index=12 ("인덱스")) -> (element=w464:u8)
                n282 = Index Array(array=w459, index=13 ("인덱스")) -> (element=w463:u8)
                n283 = local read "recall-2"() -> (w472:bool)
                n284 = control-ref of="ROM Table 2"() -> (w461:refnum<vi>)
                n285 = property on="프로퍼티 노드" class="Tbl (엄격한)"(reference=w461) -> ("Value"=w460:string[][])  [unwired: 1 in, 2 out]
                n286 = And(x=w429, y=w428) -> (x .and. y?=w430:bool)
                n287 = call "SUB_Parsing_from_table_to_cluster.vi"("ROM Table"=w460) -> ("Acclerometer value(90, 180)"=w462:T25)  [unwired: 10 in, 8 out]
                n288 = Bundle By Name(cluster=w462, "second counter_1"=w464, "second counter_2"=w463) -> (w465:T25)
                n289 = local read "Connection Status"() -> (w455:T6)
                n290 = And(x=w428, y=w472) -> (x .and. y?=w471:bool)
                n291 = And(x=w428, y="Re-call") -> (x .and. y?=w476:bool)
                n292 = And(x=w428, y="Set Inverval Time") -> (x .and. y?=w477:bool)
                n293 = case shown="참" w468 {
                  tunnel: w465 -> [_ w651]
                  frame False {
                  }
                  frame True {
                    n294 = flat-sequence {
                      tunnel: w653 -> [w657]
                      tunnel: w652 -> [w656]
                      tunnel: w651 -> [w654]
                      frame #0 {
                        n295 = Cluster To Array(cluster=w654) -> (array=w659:u8[])
                        n296 = Index Array(array=w659, index #2=1 ("인덱스"), index #6=5 ("인덱스"), index #11=10 ("인덱스"), index #16=15 ("인덱스")) -> (element #1=w667:u8, element #2=w668:u8, element #3=w669:u8, element #4=w670:u8, element #5=w671:u8, element #6=w672:u8, element #7=w673:u8, element #8=w674:u8, element #9=w675:u8, element #10=w676:u8, element #11=w677:u8, element #12=w678:u8, element #13=w679:u8, element #14=w680:u8, element #15=w681:u8, element #16=w682:u8, element #17=w683:u8)  [unwired: 14 in, 1 out]
                        n297 = Compound Arithmetic op=ADD(w668, w669, w670, w671, w672, w673, w674, w675, w676, w677, w678, w679, w680, w681, w682, w683) -> (w666:u8)
                        n298 = Subtract(x=u8 255, y=w666) -> (x-y=w655:u8)
                        "sec coun_check sum" <- w655
                        n299 = Bundle By Name(cluster=T25 {"Packet ID"=0, "Acc. X_90 val_H"=0, "Acc. X_90 val_L"=0, "Acc. Y_90 val_H"=0, "Acc. Y_90 val_L"=0, "Acc. Z_90 val_H"=0, "Acc. Z_90 val_L"=0, "Acc. X_180 val_H"=0, "Acc. X_180 val_L"=0, "Acc. Y_180 val_H"=0, "Acc. Y_180 val_L"=0, "Acc. Z_180 val_H"=0, "Acc. Z_180 val_L"=0, "second counter_1"=0, "second counter_2"=0, "Reserved_1"=0, "Reserved_2"=0, "Check sum"=0} ("Cal information"), "Packet ID"=w667, "Acc. X_90 val_H"=w668, "Acc. X_90 val_L"=w669, "Acc. Y_90 val_H"=w670, "Acc. Y_90 val_L"=w671, "Acc. Z_90 val_H"=w672, "Acc. Z_90 val_L"=w673, "Acc. X_180 val_H"=w674, "Acc. X_180 val_L"=w675, "Acc. Y_180 val_H"=w676, "Acc. Y_180 val_L"=w677, "Acc. Z_180 val_H"=w678, "Acc. Z_180 val_L"=w679, "second counter_1"=w680, "second counter_2"=w681, "Reserved_1"=w682, "Reserved_2"=w683, "Check sum"=w655) -> (w684:T25)
                        n300 = Cluster To Array(cluster=w684) -> (array=w685:u8[])
                        n301 = call-poly "ble_write_by_handle.vi"("Connection Status"=w656, "Handle"=u16 15, "data (uint8array)"=w685, "COM Bluegiga in"=w657) -> ()  [unwired: 6 in, 2 out]
                      }
                      frame #1 {
                        n302 = local write "second counter Rx"(TRUE ("불리언 8")) -> ()
                        n303 = local write "second counter Tx"(FALSE ("불리언 4")) -> ()
                        n304 = Wait (ms)(milliseconds to wait=u32 100 ("대기 시간(ms)")) -> ()  [unwired: 1 out]
                      }
                    }
                    n305 = local read "Port-act 1"() -> (w653:refnum<visa-resource-name>)
                    n306 = local read "Connection Status"() -> (w652:T6)
                  }
                }
                n307 = local read "Connection Status"() -> (w424:T6)
                n308 = And(x=w428, y="83 tx") -> (x .and. y?=w453:bool)
                n309 = And(x=w428, y="91 tx") -> (x .and. y?=w433:bool)
                n310 = And(x=w428, y="88 tx") -> (x .and. y?=w436:bool)
                n311 = And(x="Send", y=w428) -> (x .and. y?=w480:bool)
                n312 = And(x=w428, y="Mode Selection") -> (x .and. y?=w479:bool)
                n313 = And(x=w428, y="Save") -> (x .and. y?=w470:bool)
                n314 = case shown="참" w470 {
                  frame False {
                  }
                  frame True {
                    n315 = flat-sequence {
                      frame #0 {
                        n316 = local write "A1 tx"(FALSE ("A1 tx")) -> ()
                        n317 = local write "83 tx"(FALSE ("83 tx")) -> ()
                        n318 = local write "94 tx"(FALSE ("94 tx")) -> ()
                        n319 = local write "91 tx"(FALSE ("91 tx")) -> ()
                        n320 = local write "98 tx"(FALSE ("98 tx")) -> ()
                        n321 = local write "A3 tx"(FALSE ("A3 tx")) -> ()
                        n322 = local write "88 tx"(FALSE ("88 tx")) -> ()
                        n323 = local write "92 tx"(FALSE ("92 tx")) -> ()
                      }
                      frame #1 {
                        n324 = property on="ROM Table 2" class="Tbl (엄격한)"() -> ("Value"=w764:string[][])  [unwired: 2 in, 2 out]
                        n325 = call "SUB_Parsing_from_table_to_cluster.vi"("ROM Table"=w764) -> ("Device information"=w759:T1)  [unwired: 10 in, 8 out]
                        n326 = Cluster To Array(cluster=w759) -> (array=w762:u8[])
                        n327 = local read "Port-act 1"() -> (w757:refnum<visa-resource-name>)
                        n328 = local read "Connection Status"() -> (w758:T6)
                        n329 = Index Array(array=w762, index=17 ("인덱스")) -> (element=→"81 checksum":u8)
                        n330 = call-poly "ble_write_by_handle.vi"("Connection Status"=w758, "Handle"=u16 15, "data (uint8array)"=w762, "COM Bluegiga in"=w757) -> ()  [unwired: 6 in, 2 out]
                      }
                      frame #2 {
                        n331 = Wait (ms)(milliseconds to wait=u32 100 ("대기 시간(ms)")) -> ()  [unwired: 1 out]
                        n332 = local write "Save"(FALSE ("Save")) -> ()
                        "81 rx" <- TRUE ("81 rx")
                      }
                    }
                  }
                }
                n333 = local read "Port-act 1"() -> (w456:refnum<visa-resource-name>)
                n334 = case shown="참" w457 {
                  tunnel: w456 -> [_ w641]
                  tunnel: w455 -> [_ w640]
                  frame False {
                  }
                  frame True {
                    n335 = flat-sequence {
                      tunnel: w641 -> [w647]
                      tunnel: w640 -> [w646]
                      frame #0 {
                        n336 = Build Array(u16 66 ("Handle"), u16 189 ("Handle")) -> (w643:u16[])
                        n337 = call-poly "ble_write_by_handle.vi"("Connection Status"=w646, "Handle"=u16 15, "data (uint8array)"=w643, "COM Bluegiga in"=w647) -> ()  [unwired: 6 in, 2 out]
                      }
                      frame #1 {
                        n338 = Wait (ms)(milliseconds to wait=u32 100 ("대기 시간(ms)")) -> ()  [unwired: 1 out]
                        n339 = local write "42 Rx"(TRUE ("불리언 7")) -> ()
                        n340 = local write "42 Tx"(FALSE ("불리언 6")) -> ()
                      }
                    }
                  }
                }
                n341 = case shown="참" w474 {
                  tunnel: w456 -> [_ w699]
                  tunnel: w455 -> [_ w698]
                  frame False {
                  }
                  frame True {
                    n342 = flat-sequence {
                      tunnel: w698 -> [w730]
                      tunnel: w699 -> [w700]
                      frame #0 {
                        n343 = local read "Cal information"() -> (w702:T14)
                        n344 = Cluster To Array(cluster=w702) -> (array=w729:u8[])
                        n345 = Index Array(array=w729, index #2=1 ("인덱스"), index #6=5 ("인덱스"), index #11=10 ("인덱스"), index #16=15 ("인덱스")) -> (element #1=w721:u8, element #2=w720:u8, element #3=w719:u8, element #4=w718:u8, element #5=w717:u8, element #6=w716:u8, element #7=w715:u8, element #8=w714:u8, element #9=w713:u8, element #10=w712:u8, element #11=w711:u8, element #12=w710:u8, element #13=w709:u8, element #14=w708:u8, element #15=w707:u8, element #16=w706:u8, element #17=w705:u8)  [unwired: 14 in, 1 out]
                        n346 = Compound Arithmetic op=ADD(w720, w719, w718, w717, w716, w715, w714, w713, w712, w711, w710, w709, w708, w707, w706, w705) -> (w723:u8)
                        n347 = Subtract(x=u8 255, y=w723) -> (x-y=w701:u8)
                        "bat cal_check sum" <- w701
                        n348 = Bundle By Name(cluster=T14 {"Packet ID"=0, "Acc X_H_Cal"=0, "Acc X_L_Cal"=0, "Acc Y_H_Cal"=0, "Acc Y_L_Cal"=0, "Acc Z_H_Cal"=0, "Acc Z_L_Cal"=0, "Gyro X_H_Cal"=0, "Gyro X_L_Cal"=0, "Gyro Y_H_Cal"=0, "Gyro Y_L_Cal"=0, "Gyro Z_H_Cal"=0, "Gyro Z_L_Cal"=0, "Voltage H 3.1V"=0, "Voltage L 3.1V"=0, "Voltage H 2.8V"=0, "Voltage L 2.8V"=0, "Check sum"=0} ("Cal information"), "Packet ID"=w721, "Acc X_H_Cal"=w720, "Acc X_L_Cal"=w719, "Acc Y_H_Cal"=w718, "Acc Y_L_Cal"=w717, "Acc Z_H_Cal"=w716, "Acc Z_L_Cal"=w715, "Gyro X_H_Cal"=w714, "Gyro X_L_Cal"=w713, "Gyro Y_H_Cal"=w712, "Gyro Y_L_Cal"=w711, "Gyro Z_H_Cal"=w710, "Gyro Z_L_Cal"=w709, "Voltage H 3.1V"=w708, "Voltage L 3.1V"=w707, "Voltage H 2.8V"=w706, "Voltage L 2.8V"=w705, "Check sum"=w701) -> (w704:T14)
                        "cluster" <- w704
                        n349 = Cluster To Array(cluster=w704) -> (array=w703:u8[])
                        n350 = call-poly "ble_write_by_handle.vi"("Connection Status"=w730, "Handle"=u16 15, "data (uint8array)"=w703, "COM Bluegiga in"=w700) -> ()  [unwired: 6 in, 2 out]
                      }
                      frame #1 {
                        n351 = Wait (ms)(milliseconds to wait=u32 100 ("대기 시간(ms)")) -> ()  [unwired: 1 out]
                        n352 = local write "battery cal Tx"(FALSE ("불리언 3")) -> ()
                        n353 = local write "Battery cal Rx"(TRUE ("불리언 5")) -> ()
                      }
                    }
                  }
                }
                n354 = case shown="참" w477 {
                  frame False {
                  }
                  frame True {
                    n355 = local read "Connection Status"() -> (w746:T6)
                    n356 = call "SUB_Write_GEN4_Init_data_V2_0_1.vi"("Connection Status"=w746, "Mode"=write_mode."Interval Change", "Interval Time"="Interval Time") -> ()  [unwired: 24 in, 1 out]
                    n357 = property on="BLE Interval Graph" class="WFChart (엄격한)"("History Data"=dbl[] [] ("히스토리 데이터")) -> ()  [unwired: 2 in, 2 out]
                    n358 = property on="BLE Interval buf" class="WFChart (엄격한)"("History Data"=u32[] [] ("히스토리 데이터")) -> ()  [unwired: 2 in, 2 out]
                  }
                }
                n359 = case shown="참" w476 {
                  frame False {
                  }
                  frame True {
                    (unwired) u16 12 ("Handle")
                    # "데이터 전송\n- 핸들/0x01"
                    n360 = control-ref of="Re-call"() -> (w739:refnum<vi>)
                    n361 = property class="Bool (엄격한)"(reference=w739, "Value"=FALSE ("값(신호)")) -> ()  [unwired: 1 in, 2 out]
                    n362 = local read "Connection Status"() -> (w742:T6)
                    n363 = String To Byte Array(string="ARECAll") -> (unsigned byte array=w738:u8[])
                    n364 = local read "Port-act 1"() -> (w743:refnum<visa-resource-name>)
                    n365 = Build Array (concatenate)(w738, u8 12) -> (w736:u8[])
                    n366 = call-poly "ble_write_by_handle.vi"("Connection Status"=w742, "Handle"=u8 15, "data (uint8array)"=w736, "COM Bluegiga in"=w743) -> ()  [unwired: 6 in, 2 out]
                  }
                }
                n367 = case shown="참" w453 {
                  frame False {
                  }
                  frame True {
                    n368 = flat-sequence {
                      frame #0 {
                      }
                      frame #1 {
                        n369 = local read "Connection Status"() -> (w632:T6)
                        n370 = property on="ROM Table 2" class="Tbl (엄격한)"() -> ("Value"=w636:string[][])  [unwired: 2 in, 2 out]
                        n371 = local read "Port-act 1"() -> (w633:refnum<visa-resource-name>)
                        n372 = call "SUB_Parsing_from_table_to_cluster.vi"("ROM Table"=w636) -> ("Cal information"=w634:T14)  [unwired: 10 in, 8 out]
                        n373 = Cluster To Array(cluster=w634) -> (array=w631:u8[])
                        n374 = Index Array(array=w631, index=17 ("인덱스")) -> (element=→"83 checksum":u8)
                        n375 = call-poly "ble_write_by_handle.vi"("Connection Status"=w632, "Handle"=u16 15, "data (uint8array)"=w631, "COM Bluegiga in"=w633) -> ()  [unwired: 6 in, 2 out]
                      }
                      frame #2 {
                        n376 = Wait (ms)(milliseconds to wait=u32 100 ("대기 시간(ms)")) -> ()  [unwired: 1 out]
                        n377 = local write "83 tx"(FALSE ("83 tx start")) -> ()
                        "83 rx" <- TRUE ("83 rx")
                      }
                    }
                  }
                }
                n378 = case shown="참" w436 {
                  frame False {
                  }
                  frame True {
                    n379 = flat-sequence {
                      frame #0 {
                      }
                      frame #1 {
                        n380 = local read "Connection Status"() -> (w564:T6)
                        n381 = property on="ROM Table 2" class="Tbl (엄격한)"() -> ("Value"=w570:string[][])  [unwired: 2 in, 2 out]
                        n382 = local read "Port-act 1"() -> (w566:refnum<visa-resource-name>)
                        n383 = call "SUB_Parsing_from_table_to_cluster.vi"("ROM Table"=w570) -> ("PCAP zero information"=w565:T34)  [unwired: 10 in, 8 out]
                        n384 = Cluster To Array(cluster=w565) -> (array=w563:u8[])
                        n385 = Index Array(array=w563, index=17 ("인덱스")) -> (element=→"88 checksum":u8)
                        n386 = call-poly "ble_write_by_handle.vi"("Connection Status"=w564, "Handle"=u16 15, "data (uint8array)"=w563, "COM Bluegiga in"=w566) -> ()  [unwired: 6 in, 2 out]
                      }
                      frame #2 {
                        n387 = Wait (ms)(milliseconds to wait=u32 100 ("대기 시간(ms)")) -> ()  [unwired: 1 out]
                        n388 = local write "88 tx"(FALSE ("83 tx start")) -> ()
                        "88 rx" <- TRUE ("88 rx")
                      }
                    }
                  }
                }
                n389 = case shown="참" w433 {
                  frame False {
                  }
                  frame True {
                    n390 = flat-sequence {
                      frame #0 {
                        n391 = Wait (ms)(milliseconds to wait=u32 200 ("대기 시간(ms)")) -> ()  [unwired: 1 out]
                      }
                      frame #1 {
                        n392 = local read "Connection Status"() -> (w554:T6)
                        n393 = property on="ROM Table 2" class="Tbl (엄격한)"() -> ("Value"=w559:string[][])  [unwired: 2 in, 2 out]
                        n394 = local read "Port-act 1"() -> (w555:refnum<visa-resource-name>)
                        n395 = call "SUB_Parsing_from_table_to_cluster.vi"("ROM Table"=w559) -> ("data1"=w552:T35)  [unwired: 10 in, 8 out]
                        n396 = Cluster To Array(cluster=w552) -> (array=w553:u8[])
                        n397 = Index Array(array=w553, index=17 ("인덱스")) -> (element=→"91 checksum":u8)
                        n398 = call-poly "ble_write_by_handle.vi"("Connection Status"=w554, "Handle"=u16 15, "data (uint8array)"=w553, "COM Bluegiga in"=w555) -> ()  [unwired: 6 in, 2 out]
                      }
                      frame #2 {
                        n399 = Wait (ms)(milliseconds to wait=u32 100 ("대기 시간(ms)")) -> ()  [unwired: 1 out]
                        n400 = local write "91 tx"(FALSE ("83 tx start")) -> ()
                        "91 rx" <- TRUE ("88 rx")
                      }
                    }
                  }
                }
                n401 = case shown="참" w471 {
                  frame False {
                  }
                  frame True {
                    (unwired) u16 12 ("Handle")
                    # "데이터 전송\n- 핸들/0x01"
                    n402 = control-ref of="recall-2"() -> (w693:refnum<vi>)
                    n403 = property class="Bool (엄격한)"(reference=w693, "Value"=FALSE ("값(신호)")) -> ()  [unwired: 1 in, 2 out]
                    n404 = local read "Connection Status"() -> (w696:T6)
                    n405 = String To Byte Array(string="ARECAll") -> (unsigned byte array=w692:u8[])
                    n406 = local read "Port-act 1"() -> (w697:refnum<visa-resource-name>)
                    n407 = Build Array (concatenate)(w692, u8 12) -> (w690:u8[])
                    n408 = call-poly "ble_write_by_handle.vi"("Connection Status"=w696, "Handle"=u8 15, "data (uint8array)"=w690, "COM Bluegiga in"=w697) -> ()  [unwired: 6 in, 2 out]
                  }
                }
                n409 = case shown="참" w480 {
                  frame False {
                  }
                  frame True {
                    (unwired) u16 12 ("Handle")
                    # "데이터 전송\n- 핸들/0x01"
                    n410 = control-ref of="Send"() -> (w780:refnum<vi>)
                    n411 = property class="Bool (엄격한)"(reference=w780, "Value"=FALSE ("값(신호)")) -> ()  [unwired: 1 in, 2 out]
                    n412 = local read "Data(h)"() -> (w782:string)
                    n413 = local read "Connection Status"() -> (w783:T6)
                    n414 = local read "Port-act 1"() -> (w784:refnum<visa-resource-name>)
                    n415 = String To Byte Array(string=w782) -> (unsigned byte array=w781:u8[])
                    n416 = local read "Handle"() -> (w785:u8)
                    n417 = call-poly "ble_write_by_handle.vi"("Connection Status"=w783, "Handle"=w785, "data (uint8array)"=w781, "COM Bluegiga in"=w784) -> ()  [unwired: 6 in, 2 out]
                  }
                }
                n418 = case shown="참" w479 {
                  frame False {
                  }
                  frame True {
                    # "데이터 전송\n- 핸들 0x0B"
                    n419 = control-ref of="Mode Selection"() -> (w771:refnum<vi>)
                    n420 = property class="Bool (엄격한)"(reference=w771, "Value"=FALSE) -> ()  [unwired: 1 in, 2 out]
                    n421 = case shown="\"Debugging 1\"" "Operation Mode" {
                      tunnel: ["imt" ("문자열") "JsP" ("문자열") "NFT" ("문자열")] -> w768
                      frame "Normal Operation", Default {
                      }
                      frame "Debugging 1" {
                      }
                      frame "Debugging 2" {
                      }
                    }
                    n422 = local read "Connection Status"() -> (w774:T6)
                    n423 = local read "Port-act 1"() -> (w775:refnum<visa-resource-name>)
                    n424 = String To Byte Array(string=w768) -> (unsigned byte array=w773:u8[])
                    n425 = call-poly "ble_write_by_handle.vi"("Connection Status"=w774, "Handle"=u16 11, "data (uint8array)"=w773, "COM Bluegiga in"=w775) -> ()  [unwired: 6 in, 2 out]
                  }
                }
                n426 = local read "Port-act 1"() -> (w423:refnum<visa-resource-name>)
                n427 = case shown="참" w430 {
                  tunnel: w423 -> [_ w504]
                  tunnel: w424 -> [_ w503]
                  frame False {
                  }
                  frame True {
                    n428 = flat-sequence {
                      tunnel: w504 -> [w510]
                      tunnel: w503 -> [w509]
                      frame #0 {
                        n429 = Build Array(u16 66 ("Handle"), u16 189 ("Handle")) -> (w506:u16[])
                        n430 = call-poly "ble_write_by_handle.vi"("Connection Status"=w509, "Handle"=u16 15, "data (uint8array)"=w506, "COM Bluegiga in"=w510) -> ()  [unwired: 6 in, 2 out]
                      }
                      frame #1 {
                        n431 = Wait (ms)(milliseconds to wait=u32 100 ("대기 시간(ms)")) -> ()  [unwired: 1 out]
                        n432 = local write "FTS 42 Rx"(TRUE ("불리언 7")) -> ()
                        n433 = local write "FTS 42 Tx"(FALSE ("불리언 6")) -> ()
                      }
                    }
                  }
                }
                n434 = case shown="참" w431 {
                  tunnel: w424 -> [_ w515]
                  tunnel: w423 -> [_ w514]
                  frame False {
                  }
                  frame True {
                    n435 = flat-sequence {
                      tunnel: w515 -> [w517]
                      tunnel: w514 -> [w516]
                      frame #0 {
                        n436 = local read "scale A,B"() -> (w519:T1)
                        n437 = Cluster To Array(cluster=w519) -> (array=w546:u8[])
                        n438 = Index Array(array=w546, index #2=1 ("인덱스"), index #6=5 ("인덱스"), index #11=10 ("인덱스"), index #16=15 ("인덱스")) -> (element #1=w539:u8, element #2=w538:u8, element #3=w537:u8, element #4=w536:u8, element #5=w535:u8, element #6=w534:u8, element #7=w533:u8, element #8=w532:u8, element #9=w531:u8, element #10=w530:u8, element #11=w529:u8, element #12=w528:u8, element #13=w527:u8, element #14=w526:u8, element #15=w525:u8, element #16=w524:u8, element #17=w523:u8)  [unwired: 14 in, 1 out]
                        n439 = Compound Arithmetic op=ADD(w538, w537, w536, w535, w534, w533, w532, w531, w530, w529, w528, w527, w526, w525, w524, w523) -> (w540:u8)
                        n440 = Subtract(x=u8 255, y=w540) -> (x-y=w518:u8)
                        "scale A,B check" <- w518
                        n441 = Bundle By Name(cluster=T1 {"Packet ID"=0, "Device ID 1"=0, "Device ID 2"=0, "Device ID 3"=0, "Device ID 4"=0, "Year"=0, "Month"=0, "Day"=0, "Device Type H"=0, "Device Type L"=0, "Manufacturer Lot ID 1"=0, "Manufacturer Lot ID 2"=0, "Manufacturer Lot ID 3"=0, "Manufacturer Lot ID 4"=0, "Scale A"=0, "Scale B"=0, "Check sum"=0, "Check sum 2"=0} ("Device information"), "Packet ID"=w539, "Device ID 1"=w538, "Device ID 2"=w537, "Device ID 3"=w536, "Device ID 4"=w535, "Year"=w534, "Month"=w533, "Day"=w532, "Device Type H"=w531, "Device Type L"=w530, "Manufacturer Lot ID 1"=w529, "Manufacturer Lot ID 2"=w528, "Manufacturer Lot ID 3"=w527, "Manufacturer Lot ID 4"=w526, "Scale A"=w525, "Scale B"=w524, "Check sum"=w523, "Check sum 2"=w518) -> (w522:T1)
                        n442 = Cluster To Array(cluster=w522) -> (array=w521:u8[])
                        n443 = call-poly "ble_write_by_handle.vi"("Connection Status"=w517, "Handle"=u16 15, "data (uint8array)"=w521, "COM Bluegiga in"=w516) -> ()  [unwired: 6 in, 2 out]
                      }
                      frame #1 {
                        n444 = local write "scale A,B Rx"(TRUE ("scale A,B Rx")) -> ()
                        n445 = local write "scale A.B Tx"(FALSE ("scale A.B")) -> ()
                        n446 = Wait (ms)(milliseconds to wait=u32 100 ("대기 시간(ms)")) -> ()  [unwired: 1 out]
                      }
                    }
                  }
                }
                n447 = local read "Comm con status 1"() -> (w425:bool)
                n448 = local read "FTS device out"() -> (w426:bool)
                n449 = And(x=w426, y=w425) -> (x .and. y?=w427:bool)
                n450 = case shown="참" w427 {
                  frame False {
                  }
                  frame True {
                    n451 = stacked-sequence {
                      frame #0 {
                        n452 = local write "FTS device out"(FALSE ("FTS device out")) -> ()
                      }
                      frame #1 {
                        n453 = local read "Connection Status"() -> (w494:T6)
                        n454 = local read "Port-act 1"() -> (w493:refnum<visa-resource-name>)
                        n455 = String To Byte Array(string="DYSKIMr" ("Data(h)")) -> (unsigned byte array=w497:u8[])
                        n456 = call-poly "ble_write_by_handle.vi"("Connection Status"=w494, "Handle"=u16 15, "data (uint8array)"=w497, "COM Bluegiga in"=w493) -> ()  [unwired: 6 in, 2 out]
                      }
                      frame #2 {
                        n457 = Wait (ms)(milliseconds to wait=u32 100 ("대기 시간(ms)")) -> ()  [unwired: 1 out]
                      }
                      frame #3 {
                        n458 = control-ref of="Comm con 1"() -> (w500:refnum<vi>)
                        n459 = property class="Bool (엄격한)"(reference=w500, "Val(Sgnl)"=FALSE ("값(신호)")) -> ()  [unwired: 1 in, 2 out]
                      }
                      frame #4 {
                        n460 = control-ref of="PWR OFF"() -> (w502:refnum<vi>)
                        n461 = property class="Bool (엄격한)"(reference=w502, "Val(Sgnl)"=FALSE ("값(신호)")) -> ()  [unwired: 1 in, 2 out]
                      }
                    }
                  }
                }
                n462 = local read "Comm con status 1"() -> (w421:bool)
                n463 = local read "Comm con status 1"() -> (w437:bool)
                n464 = local read "Comm con status 1"() -> (w448:bool)
                n465 = local read "Comm con status 1"() -> (w443:bool)
                n466 = local read "Comm con status 1"() -> (w442:bool)
                n467 = local read "Comm con status 1"() -> (w449:bool)
                n468 = local read "Test Start"() -> (w422:bool)
                n469 = And(x=w422, y=w421) -> (x .and. y?=w420:bool)
                n470 = And(x=w437, y="A3 tx") -> (x .and. y?=w439:bool)
                n471 = And(x=w448, y="94 tx") -> (x .and. y?=w446:bool)
                n472 = And(x=w443, y="98 tx") -> (x .and. y?=w445:bool)
                n473 = And(x=w442, y="A1 tx") -> (x .and. y?=w440:bool)
                n474 = And(x=w449, y="92 tx") -> (x .and. y?=w451:bool)
                n475 = case shown="참" w420 {
                  frame False {
                  }
                  frame True {
                    n476 = flat-sequence {
                      frame #0 {
                        n477 = local read "Connection Status"() -> (w483:T6)
                        n478 = local read "Port-act 1"() -> (w484:refnum<visa-resource-name>)
                        n479 = Build Array(u16 72 ("Handle"), u16 183 ("Handle")) -> (w487:u16[])
                        n480 = call-poly "ble_write_by_handle.vi"("Connection Status"=w483, "Handle"=u16 15, "data (uint8array)"=w487, "COM Bluegiga in"=w484) -> ()  [unwired: 6 in, 2 out]
                      }
                      frame #1 {
                        n481 = Wait (ms)(milliseconds to wait=u32 100 ("대기 시간(ms)")) -> ()  [unwired: 1 out]
                      }
                      frame #2 {
                        n482 = local write "FTS start"(TRUE ("FTS start")) -> ()
                        n483 = local write "Test Start"(FALSE ("Test Start")) -> ()
                      }
                    }
                  }
                }
                n484 = case shown="참" w439 {
                  frame False {
                  }
                  frame True {
                    n485 = flat-sequence {
                      frame #0 {
                      }
                      frame #1 {
                        n486 = local read "Connection Status"() -> (w576:T6)
                        n487 = property on="ROM Table 2" class="Tbl (엄격한)"() -> ("Value"=w581:string[][])  [unwired: 2 in, 2 out]
                        n488 = local read "Port-act 1"() -> (w577:refnum<visa-resource-name>)
                        n489 = call "SUB_Parsing_from_table_to_cluster.vi"("ROM Table"=w581) -> ("Acclerometer value(90, 180)"=w574:T25)  [unwired: 10 in, 8 out]
                        n490 = Cluster To Array(cluster=w574) -> (array=w575:u8[])
                        n491 = Index Array(array=w575, index=17 ("인덱스")) -> (element=→"A3 checksum":u8)
                        n492 = call-poly "ble_write_by_handle.vi"("Connection Status"=w576, "Handle"=u16 15, "data (uint8array)"=w575, "COM Bluegiga in"=w577) -> ()  [unwired: 6 in, 2 out]
                      }
                      frame #2 {
                        n493 = Wait (ms)(milliseconds to wait=u32 100 ("대기 시간(ms)")) -> ()  [unwired: 1 out]
                        n494 = local write "A3 tx"(FALSE ("83 tx start")) -> ()
                        "A3 rx" <- TRUE ("88 rx")
                      }
                    }
                  }
                }
                n495 = case shown="참" w446 {
                  frame False {
                  }
                  frame True {
                    n496 = flat-sequence {
                      frame #0 {
                      }
                      frame #1 {
                        n497 = local read "Connection Status"() -> (w609:T6)
                        n498 = property on="ROM Table 2" class="Tbl (엄격한)"() -> ("Value"=w614:string[][])  [unwired: 2 in, 2 out]
                        n499 = local read "Port-act 1"() -> (w610:refnum<visa-resource-name>)
                        n500 = call "SUB_Parsing_from_table_to_cluster.vi"("ROM Table"=w614) -> ("data3"=w607:T36)  [unwired: 10 in, 8 out]
                        n501 = Cluster To Array(cluster=w607) -> (array=w608:u8[])
                        n502 = Index Array(array=w608, index=17 ("인덱스")) -> (element=→"94 checksum":u8)
                        n503 = call-poly "ble_write_by_handle.vi"("Connection Status"=w609, "Handle"=u16 15, "data (uint8array)"=w608, "COM Bluegiga in"=w610) -> ()  [unwired: 6 in, 2 out]
                      }
                      frame #2 {
                        n504 = Wait (ms)(milliseconds to wait=u32 100 ("대기 시간(ms)")) -> ()  [unwired: 1 out]
                        n505 = local write "94 tx"(FALSE ("83 tx start")) -> ()
                        "94 rx" <- TRUE ("88 rx")
                      }
                    }
                  }
                }
                n506 = case shown="참" w445 {
                  frame False {
                  }
                  frame True {
                    n507 = flat-sequence {
                      frame #0 {
                      }
                      frame #1 {
                        n508 = local read "Connection Status"() -> (w598:T6)
                        n509 = property on="ROM Table 2" class="Tbl (엄격한)"() -> ("Value"=w603:string[][])  [unwired: 2 in, 2 out]
                        n510 = local read "Port-act 1"() -> (w599:refnum<visa-resource-name>)
                        n511 = call "SUB_Parsing_from_table_to_cluster.vi"("ROM Table"=w603) -> ("data4"=w596:T37)  [unwired: 10 in, 8 out]
                        n512 = Cluster To Array(cluster=w596) -> (array=w597:u8[])
                        n513 = Index Array(array=w597, index=17 ("인덱스")) -> (element=→"98 checksum":u8)
                        n514 = call-poly "ble_write_by_handle.vi"("Connection Status"=w598, "Handle"=u16 15, "data (uint8array)"=w597, "COM Bluegiga in"=w599) -> ()  [unwired: 6 in, 2 out]
                      }
                      frame #2 {
                        n515 = Wait (ms)(milliseconds to wait=u32 100 ("대기 시간(ms)")) -> ()  [unwired: 1 out]
                        n516 = local write "98 tx"(FALSE ("83 tx start")) -> ()
                        "98 rx" <- TRUE ("88 rx")
                      }
                    }
                  }
                }
                n517 = case shown="참" w440 {
                  frame False {
                  }
                  frame True {
                    n518 = flat-sequence {
                      frame #0 {
                      }
                      frame #1 {
                        n519 = local read "Connection Status"() -> (w587:T6)
                        n520 = property on="ROM Table 2" class="Tbl (엄격한)"() -> ("Value"=w592:string[][])  [unwired: 2 in, 2 out]
                        n521 = local read "Port-act 1"() -> (w588:refnum<visa-resource-name>)
                        n522 = call "SUB_Parsing_from_table_to_cluster.vi"("ROM Table"=w592) -> ("Acclerometer value(0, 45)"=w585:T38)  [unwired: 10 in, 8 out]
                        n523 = Cluster To Array(cluster=w585) -> (array=w586:u8[])
                        n524 = Index Array(array=w586, index=17 ("인덱스")) -> (element=→"A1 checksum":u8)
                        n525 = call-poly "ble_write_by_handle.vi"("Connection Status"=w587, "Handle"=u16 15, "data (uint8array)"=w586, "COM Bluegiga in"=w588) -> ()  [unwired: 6 in, 2 out]
                      }
                      frame #2 {
                        n526 = Wait (ms)(milliseconds to wait=u32 100 ("대기 시간(ms)")) -> ()  [unwired: 1 out]
                        n527 = local write "A1 tx"(FALSE ("83 tx start")) -> ()
                        "A1 rx" <- TRUE ("88 rx")
                      }
                    }
                  }
                }
                n528 = case shown="참" w451 {
                  frame False {
                  }
                  frame True {
                    n529 = flat-sequence {
                      frame #0 {
                      }
                      frame #1 {
                        n530 = local read "Connection Status"() -> (w620:T6)
                        n531 = property on="ROM Table 2" class="Tbl (엄격한)"() -> ("Value"=w625:string[][])  [unwired: 2 in, 2 out]
                        n532 = local read "Port-act 1"() -> (w621:refnum<visa-resource-name>)
                        n533 = call "SUB_Parsing_from_table_to_cluster.vi"("ROM Table"=w625) -> ("data2"=w618:T39)  [unwired: 10 in, 8 out]
                        n534 = Cluster To Array(cluster=w618) -> (array=w619:u8[])
                        n535 = Index Array(array=w619, index=17 ("인덱스")) -> (element=→"92 checksum":u8)
                        n536 = call-poly "ble_write_by_handle.vi"("Connection Status"=w620, "Handle"=u16 15, "data (uint8array)"=w619, "COM Bluegiga in"=w621) -> ()  [unwired: 6 in, 2 out]
                      }
                      frame #2 {
                        n537 = Wait (ms)(milliseconds to wait=u32 100 ("대기 시간(ms)")) -> ()  [unwired: 1 out]
                        n538 = local write "92 tx"(FALSE ("83 tx start")) -> ()
                        "92 rx" <- TRUE ("88 rx")
                      }
                    }
                  }
                }
              }
              frame 4.. {
                # "Rx Packet Data - Process"
                n539 = call "ble_read_message.vi"("error in (no error)"=w787, "COM Bluegiga in"=w788) -> ("message package"=w786:u8[])  [unwired: 7 in, 2 out]
                n540 = stacked-sequence {
                  seq-local: [_ w794 _ _ _ _] -> [_ _ w1067 w1077 w1081 w1092]
                  tunnel: w786 -> [_ w795 _ _ _ _]
                  frame #0 {
                    n541 = local write "Packet Detect"(FALSE ("Packet Detect")) -> ()
                  }
                  frame #1 {
                    # "ble_evt_attclient_attribute_value"
                    n542 = call "BLED1112-Rx Packet parser (EVENT-Attribute Client).vi"("message package"=w795) -> ("message out"=w794:u8[], "Packet OK"=w793:bool, "Data Structure"=w792:T3)  [unwired: 2 in]
                    n543 = case shown="참" w793 {
                      tunnel: w792 -> [_ w796]
                      frame False {
                      }
                      frame True {
                        n544 = stacked-sequence {
                          tunnel: w796 -> [w801 _]
                          frame #0 {
                            n545 = local read "Data Logging"() -> (w800:bool)
                            n546 = Unbundle By Name(w801) -> ("Attribute value (data)"=w802:u8[])
                            n547 = local write "Packet Detect"(TRUE ("Packet Detect")) -> ()
                            n548 = Byte Array To String(unsigned byte array=w802) -> (string=w805:string)
                            n549 = local write "Rx buf 1"(w805) -> ()
                            n550 = call "SUB-BLE Rx data save.vi"("BLE RxD"=w802, "Rx Packet Structure"=w801) -> ("Mon Packet?"=w798:bool, "Full packet"=w797:u8[])  [unwired: 2 in, 3 out]
                            n551 = And(x=w798, y=w800) -> (x .and. y?=w799:bool)
                            n552 = case shown="참" w798 {
                              frame False {
                              }
                              frame True {
                                n553 = local read "ms timer 4"() -> (w809:u32)
                                n554 = Tick Count (ms)() -> (millisecond timer value=w807:u32)
                                n555 = Subtract(x=w807, y=w809) -> (x-y=→"BLE Interval buf":u32)
                                n556 = local write "ms timer 4"(w807) -> ()
                              }
                            }
                            n557 = local read "Rx Cnt"() -> (w803:i32)
                            n558 = case shown="참" w799 {
                              tunnel: w797 -> [_ w814]
                              tunnel: w803 -> [_ w811]
                              frame False {
                              }
                              frame True {
                                # "Save log data"
                                n559 = local read "log ble buf"() -> (w819:string)
                                n560 = Format Into String(format string="%06d," ("포맷 문자열"), w811) -> (resulting string=w812:string)  [unwired: 2 in, 1 out]
                                n561 = Array To Spreadsheet String(delimiter (Tab)="," ("포맷 문자열"), array=w814, 3:"%02X" ("포맷 문자열")) -> (spreadsheet string=w815:string)
                                n562 = Format Date/Time String(time format string (%c)="%H:%M:%S%3u," ("상태")) -> (date/time string=w817:string)  [unwired: 2 in]
                                n563 = Concatenate Strings(w819, w812, w817, w815) -> (w818:string)
                                n564 = local write "log ble buf"(w818) -> ()
                                n565 = local write "log data1"(TRUE ("log data1")) -> ()
                              }
                            }
                            n566 = Increment(x=w803) -> (x+1=w806:i32)
                            n567 = local write "Rx Cnt"(w806) -> ()
                            "Rx Packet Structure" <- w801
                          }
                          frame #1 {
                            # "FTS x42 Rx"
                            # "scale A,B Rx"
                            # "A3 Rx"
                            # "A1 Rx"
                            # "98 Rx"
                            # "94 Rx"
                            # "92 Rx"
                            # "91 Rx"
                            # "88 Rx"
                            # "83 Rx"
                            # "81 Rx"
                            # "second counter Rx"
                            # "x42 Rx"
                            # "battery cal Rx"
                            # "battery calibration"
                            n568 = global read "global 4.vi" "global set packet data out"() -> (w825:u8[])
                            n569 = global read "Global 1.vi" "BLE Set Packet"() -> (w823:bool)
                            n570 = local read "sec coun_check sum"() -> (w873:u8)
                            n571 = local read "scale A,B check"() -> (w838:u8)
                            n572 = local read "A1 checksum"() -> (w947:u8)
                            n573 = local read "98 checksum"() -> (w940:u8)
                            n574 = local read "A3 checksum"() -> (w960:u8)
                            n575 = local read "94 checksum"() -> (w927:u8)
                            n576 = local read "83 checksum"() -> (w882:u8)
                            n577 = local read "91 checksum"() -> (w907:u8)
                            n578 = local read "92 checksum"() -> (w920:u8)
                            n579 = local read "81 checksum"() -> (w901:u8)
                            n580 = local read "88 checksum"() -> (w895:u8)
                            n581 = local read "bat cal_check sum"() -> (w853:u8)
                            n582 = Index Array(array=w825, index=1 ("인덱스")) -> (element=w846:u8)
                            n583 = Index Array(array=w825, index=0 ("인덱스")) -> (element=w847:u8)
                            n584 = Index Array(array=w825, index=1 ("인덱스")) -> (element=w946:u8)
                            n585 = Index Array(array=w825, index=1 ("인덱스")) -> (element=w941:u8)
                            n586 = Index Array(array=w825, index=1 ("인덱스")) -> (element=w961:u8)
                            n587 = Index Array(array=w825, index=1 ("인덱스")) -> (element=w926:u8)
                            n588 = Index Array(array=w825, index=1 ("인덱스")) -> (element=w881:u8)
                            n589 = Index Array(array=w825, index=1 ("인덱스")) -> (element=w906:u8)
                            n590 = Index Array(array=w825, index=1 ("인덱스")) -> (element=w921:u8)
                            n591 = Index Array(array=w825, index=0 ("인덱스")) -> (element=w945:u8)
                            n592 = Index Array(array=w825, index=1 ("인덱스")) -> (element=w868:u8)
                            n593 = Index Array(array=w825, index=1 ("인덱스")) -> (element=w880:u8)
                            n594 = Index Array(array=w825, index=1 ("인덱스")) -> (element=w896:u8)
                            n595 = Index Array(array=w825, index=0 ("인덱스")) -> (element=w942:u8)
                            n596 = Index Array(array=w825, index=0 ("인덱스")) -> (element=w962:u8)
                            n597 = Index Array(array=w825, index=0 ("인덱스")) -> (element=w925:u8)
                            n598 = Index Array(array=w825, index=0 ("인덱스")) -> (element=w857:u8)
                            n599 = Index Array(array=w825, index=1 ("인덱스")) -> (element=w858:u8)
                            n600 = Index Array(array=w825, index=0 ("인덱스")) -> (element=w897:u8)
                            n601 = Index Array(array=w825, index=0 ("인덱스")) -> (element=w905:u8)
                            n602 = Index Array(array=w825, index=0 ("인덱스")) -> (element=w922:u8)
                            n603 = Index Array(array=w825, index=0 ("인덱스")) -> (element=w867:u8)
                            n604 = Index Array(array=w825, index=0 ("인덱스")) -> (element=w898:u8)
                            n605 = Index Array(array=w825, index=0 ("인덱스")) -> (element=w899:u8)
                            n606 = Index Array(array=w825, index=0 ("인덱스")) -> (element=w832:u8)
                            n607 = Index Array(array=w825, index=1 ("인덱스")) -> (element=w831:u8)
                            n608 = Index Array(array=w825, index=1 ("인덱스")) -> (element=w839:u8)
                            n609 = Index Array(array=w825, index=0 ("인덱스")) -> (element=w840:u8)
                            n610 = Equal?(x=w846, y=w853) -> (x = y?=w851:bool)
                            n611 = Equal?(x=w946, y=w947) -> (x = y?=w953:bool)
                            n612 = Equal?(x=w941, y=w940) -> (x = y?=w934:bool)
                            n613 = Equal?(x=w961, y=w960) -> (x = y?=w954:bool)
                            n614 = Equal?(x=w926, y=w927) -> (x = y?=w933:bool)
                            n615 = Equal?(x=w847, y=u8 255) -> (x = y?=w852:bool)
                            n616 = Equal?(x=w881, y=w882) -> (x = y?=w888:bool)
                            n617 = Equal?(x=w906, y=w907) -> (x = y?=w913:bool)
                            n618 = Equal?(x=w921, y=w920) -> (x = y?=w914:bool)
                            n619 = Equal?(x=w868, y=w873) -> (x = y?=w872:bool)
                            n620 = Equal?(x=w880, y=w901) -> (x = y?=w874:bool)
                            n621 = Equal?(x=w896, y=w895) -> (x = y?=w889:bool)
                            n622 = Equal?(x=w858, y=u8 189) -> (x = y?=w863:bool)
                            n623 = Equal?(x=w831, y=u8 189) -> (x = y?=w826:bool)
                            n624 = Equal?(x=w839, y=w838) -> (x = y?=w836:bool)
                            n625 = Equal?(x=w945, y=u8 255 ("y 6")) -> (x = y?=w952:bool)
                            n626 = Equal?(x=w942, y=u8 255 ("y 6")) -> (x = y?=w935:bool)
                            n627 = Equal?(x=w962, y=u8 255 ("y 6")) -> (x = y?=w955:bool)
                            n628 = Equal?(x=w925, y=u8 255 ("y 6")) -> (x = y?=w932:bool)
                            n629 = Equal?(x=w857, y=u8 255 ("y 2")) -> (x = y?=w862:bool)
                            n630 = Equal?(x=w897, y=u8 255 ("y 5")) -> (x = y?=w887:bool)
                            n631 = Equal?(x=w905, y=u8 255 ("y 6")) -> (x = y?=w912:bool)
                            n632 = Equal?(x=w922, y=u8 255 ("y 6")) -> (x = y?=w915:bool)
                            n633 = Equal?(x=w867, y=u8 255 ("y 3")) -> (x = y?=w871:bool)
                            n634 = Equal?(x=w898, y=u8 255 ("y 4")) -> (x = y?=w875:bool)
                            n635 = Equal?(x=w899, y=u8 255 ("y 6")) -> (x = y?=w890:bool)
                            n636 = Equal?(x=w832, y=u8 255 ("y 2")) -> (x = y?=w827:bool)
                            n637 = Equal?(x=w840, y=u8 255 ("y 3")) -> (x = y?=w837:bool)
                            n638 = local read "Battery cal Rx"() -> (w845:bool)
                            n639 = local read "second counter Rx"() -> (w870:bool)
                            n640 = local read "FTS 42 Rx"() -> (w829:bool)
                            n641 = local read "42 Rx"() -> (w860:bool)
                            n642 = local read "scale A,B Rx"() -> (w824:bool)
                            n643 = local read "A1 rx"() -> (w944:bool)
                            n644 = local read "98 rx"() -> (w943:bool)
                            n645 = local read "A3 rx"() -> (w963:bool)
                            n646 = local read "94 rx"() -> (w924:bool)
                            n647 = local read "83 rx"() -> (w902:bool)
                            n648 = local read "91 rx"() -> (w904:bool)
                            n649 = local read "92 rx"() -> (w923:bool)
                            n650 = local read "81 rx"() -> (w900:bool)
                            n651 = local read "88 rx"() -> (w903:bool)
                            n652 = And(x=w845, y=w823) -> (x .and. y?=w844:bool)
                            n653 = And(x=w860, y=w823) -> (x .and. y?=w859:bool)
                            n654 = And(x=w944, y=w823) -> (x .and. y?=w951:bool)
                            n655 = And(x=w943, y=w823) -> (x .and. y?=w936:bool)
                            n656 = And(x=w963, y=w823) -> (x .and. y?=w956:bool)
                            n657 = And(x=w924, y=w823) -> (x .and. y?=w931:bool)
                            n658 = And(x=w829, y=w823) -> (x .and. y?=w830:bool)
                            n659 = And(x=w902, y=w823) -> (x .and. y?=w886:bool)
                            n660 = And(x=w904, y=w823) -> (x .and. y?=w911:bool)
                            n661 = And(x=w923, y=w823) -> (x .and. y?=w916:bool)
                            n662 = And(x=w870, y=w823) -> (x .and. y?=w869:bool)
                            n663 = And(x=w900, y=w823) -> (x .and. y?=w876:bool)
                            n664 = And(x=w903, y=w823) -> (x .and. y?=w891:bool)
                            n665 = case shown="참" w844 {
                              tunnel: w851 -> [_ w1058]
                              tunnel: w852 -> [_ w1057]
                              frame False {
                              }
                              frame True {
                                n666 = And(x=w1057, y=w1058) -> (x .and. y?=w1056:bool)
                                n667 = case shown="거짓" w1056 {
                                frame False {
                                n668 = local write "Battery cal Rx"(FALSE ("Error")) -> ()
                                n669 = local write "Error"(TRUE ("Error")) -> ()
                                n670 = local write "Status"("Wait.." ("문자열")) -> ()
                                n671 = One Button Dialog(message="ACK ERROR!\nReinspection" ("메시지")) -> ()  [unwired: 1 in, 1 out]
                                }
                                frame True {
                                n672 = local write "Battery cal Rx"(FALSE ("Error")) -> ()
                                n673 = local write "Error"(FALSE ("Error")) -> ()
                                n674 = local write "42 Tx"(TRUE ("불리언 6")) -> ()
                                }
                                }
                              }
                            }
                            n675 = And(x=w824, y=w823) -> (x .and. y?=w822:bool)
                            n676 = case shown="참" w951 {
                              tunnel: w952 -> [_ w986]
                              tunnel: w953 -> [_ w985]
                              frame False {
                              }
                              frame True {
                                n677 = And(x=w986, y=w985) -> (x .and. y?=w987:bool)
                                n678 = case shown="참" w987 {
                                frame False {
                                n679 = local write "A1 rx"(FALSE ("불리언 8")) -> ()
                                n680 = One Button Dialog(message=" A1 packet ACK ERROR!" ("메시지")) -> ()  [unwired: 1 in, 1 out]
                                }
                                frame True {
                                n681 = local write "A3 tx"(TRUE ("불리언 6")) -> ()
                                n682 = local write "A1 rx"(FALSE ("불리언 8")) -> ()
                                }
                                }
                              }
                            }
                            n683 = case shown="참" w936 {
                              tunnel: w935 -> [_ w993]
                              tunnel: w934 -> [_ w992]
                              frame False {
                              }
                              frame True {
                                n684 = And(x=w993, y=w992) -> (x .and. y?=w994:bool)
                                n685 = case shown="참" w994 {
                                frame False {
                                n686 = local write "98 rx"(FALSE ("불리언 8")) -> ()
                                n687 = One Button Dialog(message=" 98 packet ACK ERROR!" ("메시지")) -> ()  [unwired: 1 in, 1 out]
                                }
                                frame True {
                                n688 = local write "A1 tx"(TRUE ("불리언 6")) -> ()
                                n689 = local write "98 rx"(FALSE ("불리언 8")) -> ()
                                }
                                }
                              }
                            }
                            n690 = case shown="참" w956 {
                              tunnel: w955 -> [_ w979]
                              tunnel: w954 -> [_ w978]
                              frame False {
                              }
                              frame True {
                                n691 = And(x=w979, y=w978) -> (x .and. y?=w980:bool)
                                n692 = case shown="참" w980 {
                                frame False {
                                n693 = local write "A3 rx"(FALSE ("불리언 8")) -> ()
                                n694 = One Button Dialog(message=" A3 packet ACK ERROR!" ("메시지")) -> ()  [unwired: 1 in, 1 out]
                                }
                                frame True {
                                n695 = local write "42 Tx"(TRUE ("불리언 6")) -> ()
                                n696 = local write "A3 rx"(FALSE ("불리언 8")) -> ()
                                }
                                }
                              }
                            }
                            n697 = case shown="참" w931 {
                              tunnel: w932 -> [_ w1000]
                              tunnel: w933 -> [_ w999]
                              frame False {
                              }
                              frame True {
                                n698 = And(x=w1000, y=w999) -> (x .and. y?=w1001:bool)
                                n699 = case shown="참" w1001 {
                                frame False {
                                n700 = local write "94 rx"(FALSE ("불리언 8")) -> ()
                                n701 = One Button Dialog(message=" 94 packet ACK ERROR!" ("메시지")) -> ()  [unwired: 1 in, 1 out]
                                }
                                frame True {
                                n702 = local write "98 tx"(TRUE ("불리언 6")) -> ()
                                n703 = local write "94 rx"(FALSE ("불리언 8")) -> ()
                                }
                                }
                              }
                            }
                            n704 = case shown="참" w859 {
                              tunnel: w862 -> [_ w1049]
                              tunnel: w863 -> [_ w1048]
                              frame False {
                              }
                              frame True {
                                n705 = And(x=w1049, y=w1048) -> (x .and. y?=w1050:bool)
                                n706 = case shown="참" w1050 {
                                frame False {
                                n707 = local write "42 Rx"(FALSE ("불리언 6")) -> ()
                                n708 = local write "Status"("Wait.." ("문자열")) -> ()
                                n709 = One Button Dialog(message=" 42 packet ACK ERROR!" ("메시지")) -> ()  [unwired: 1 in, 1 out]
                                }
                                frame True {
                                n710 = local write "42 Rx"(FALSE ("불리언 6")) -> ()
                                n711 = local write "Status"("Finish!" ("문자열")) -> ()
                                }
                                }
                              }
                            }
                            n712 = case shown="참" w822 {
                              tunnel: w837 -> [_ w972]
                              tunnel: w836 -> [_ w971]
                              frame False {
                              }
                              frame True {
                                n713 = And(x=w972, y=w971) -> (x .and. y?=w973:bool)
                                n714 = case shown="참" w973 {
                                frame False {
                                n715 = local write "scale A,B Rx"(FALSE ("불리언 8")) -> ()
                                n716 = One Button Dialog(message="81 packet ACK ERROR!" ("메시지")) -> ()  [unwired: 1 in, 1 out]
                                }
                                frame True {
                                n717 = local write "second counter Tx"(TRUE ("불리언 6")) -> ()
                                n718 = local write "scale A,B Rx"(FALSE ("불리언 8")) -> ()
                                }
                                }
                              }
                            }
                            n719 = case shown="참" w886 {
                              tunnel: w887 -> [_ w1028]
                              tunnel: w888 -> [_ w1027]
                              frame False {
                              }
                              frame True {
                                n720 = And(x=w1028, y=w1027) -> (x .and. y?=w1029:bool)
                                n721 = case shown="참" w1029 {
                                frame False {
                                n722 = local write "83 rx"(FALSE ("불리언 8")) -> ()
                                n723 = One Button Dialog(message=" 83 packet ACK ERROR!" ("메시지")) -> ()  [unwired: 1 in, 1 out]
                                }
                                frame True {
                                n724 = local write "88 tx"(TRUE ("불리언 6")) -> ()
                                n725 = local write "83 rx"(FALSE ("불리언 8")) -> ()
                                }
                                }
                              }
                            }
                            n726 = case shown="참" w911 {
                              tunnel: w912 -> [_ w1014]
                              tunnel: w913 -> [_ w1013]
                              frame False {
                              }
                              frame True {
                                n727 = And(x=w1014, y=w1013) -> (x .and. y?=w1015:bool)
                                n728 = case shown="참" w1015 {
                                frame False {
                                n729 = local write "91 rx"(FALSE ("불리언 8")) -> ()
                                n730 = One Button Dialog(message=" 91 packet ACK ERROR!" ("메시지")) -> ()  [unwired: 1 in, 1 out]
                                }
                                frame True {
                                n731 = local write "92 tx"(TRUE ("불리언 6")) -> ()
                                n732 = local write "91 rx"(FALSE ("불리언 8")) -> ()
                                }
                                }
                              }
                            }
                            n733 = case shown="참" w916 {
                              tunnel: w915 -> [_ w1007]
                              tunnel: w914 -> [_ w1006]
                              frame False {
                              }
                              frame True {
                                n734 = And(x=w1007, y=w1006) -> (x .and. y?=w1008:bool)
                                n735 = case shown="참" w1008 {
                                frame False {
                                n736 = local write "92 rx"(FALSE ("불리언 8")) -> ()
                                n737 = One Button Dialog(message=" 92 packet ACK ERROR!" ("메시지")) -> ()  [unwired: 1 in, 1 out]
                                }
                                frame True {
                                n738 = local write "94 tx"(TRUE ("불리언 6")) -> ()
                                n739 = local write "92 rx"(FALSE ("불리언 8")) -> ()
                                }
                                }
                              }
                            }
                            n740 = case shown="참" w869 {
                              tunnel: w871 -> [_ w1042]
                              tunnel: w872 -> [_ w1041]
                              frame False {
                              }
                              frame True {
                                n741 = And(x=w1042, y=w1041) -> (x .and. y?=w1043:bool)
                                n742 = case shown="참" w1043 {
                                frame False {
                                n743 = local write "second counter Rx"(FALSE ("불리언 8")) -> ()
                                n744 = One Button Dialog(message=" A3 packet ACK ERROR!" ("메시지")) -> ()  [unwired: 1 in, 1 out]
                                }
                                frame True {
                                n745 = local write "FTS 42 Tx"(TRUE ("불리언 6")) -> ()
                                n746 = local write "second counter Rx"(FALSE ("불리언 8")) -> ()
                                }
                                }
                              }
                            }
                            n747 = case shown="참" w876 {
                              tunnel: w875 -> [_ w1035]
                              tunnel: w874 -> [_ w1034]
                              frame False {
                              }
                              frame True {
                                n748 = And(x=w1035, y=w1034) -> (x .and. y?=w1036:bool)
                                n749 = case shown="참" w1036 {
                                frame False {
                                n750 = local write "81 rx"(FALSE ("불리언 8")) -> ()
                                n751 = One Button Dialog(message=" 81 packet ACK ERROR!" ("메시지")) -> ()  [unwired: 1 in, 1 out]
                                }
                                frame True {
                                n752 = local write "83 tx"(TRUE ("불리언 6")) -> ()
                                n753 = local write "81 rx"(FALSE ("불리언 8")) -> ()
                                }
                                }
                              }
                            }
                            n754 = case shown="참" w891 {
                              tunnel: w890 -> [_ w1021]
                              tunnel: w889 -> [_ w1020]
                              frame False {
                              }
                              frame True {
                                n755 = And(x=w1021, y=w1020) -> (x .and. y?=w1022:bool)
                                n756 = case shown="참" w1022 {
                                frame False {
                                n757 = local write "88 rx"(FALSE ("불리언 8")) -> ()
                                n758 = One Button Dialog(message=" 88 packet ACK ERROR!" ("메시지")) -> ()  [unwired: 1 in, 1 out]
                                }
                                frame True {
                                n759 = local write "91 tx"(TRUE ("불리언 6")) -> ()
                                n760 = local write "88 rx"(FALSE ("불리언 8")) -> ()
                                }
                                }
                              }
                            }
                            n761 = case shown="참" w830 {
                              tunnel: w827 -> [_ w965]
                              tunnel: w826 -> [_ w964]
                              frame False {
                              }
                              frame True {
                                n762 = And(x=w965, y=w964) -> (x .and. y?=w966:bool)
                                n763 = case shown="참" w966 {
                                frame False {
                                n764 = local write "FTS 42 Rx"(FALSE ("불리언 6")) -> ()
                                n765 = One Button Dialog(message=" 42 packet ACK ERROR!" ("메시지")) -> ()  [unwired: 1 in, 1 out]
                                }
                                frame True {
                                n766 = local write "FTS device out"(TRUE ("불리언")) -> ()
                                n767 = local write "FTS 42 Rx"(FALSE ("불리언 6")) -> ()
                                }
                                }
                              }
                            }
                          }
                        }
                      }
                    }
                  }
                  frame #2 {
                    # "Rx Packet parser (EVENT-Connection status)"
                    n768 = local read "Packet Detect"() -> (w1066:bool)
                    n769 = case shown="거짓" w1066 {
                      tunnel: w1067 -> [w1070 _]
                      frame False {
                        n770 = call "BLED1112-Rx Packet parser (EVENT-Connection status).vi"("message package"=w1070) -> ("Packet OK"=w1069:bool, "Data Structure"=w1068:T40)  [unwired: 2 in, 1 out]
                        n771 = case shown="참" w1069 {
                          tunnel: w1068 -> [_ w1075]
                          frame False {
                          }
                          frame True {
                            n772 = Unbundle By Name(w1075) -> ("bonding(0xFF)"=w1074:u8)
                            n773 = local write "Packet Detect"(TRUE ("Packet Detect")) -> ()
                            n774 = Not Equal?(x=w1074, y=255 ("Rx Cnt")) -> (x != y?=w1072:bool)
                            n775 = local write "Disconnected"(w1072) -> ()
                          }
                        }
                      }
                      frame True {
                      }
                    }
                  }
                  frame #3 {
                    # "Rx Packet parser (RESPONSE GAP)"
                    n776 = local read "Packet Detect"() -> (w1076:bool)
                    n777 = case shown="거짓" w1076 {
                      tunnel: w1077 -> [w1079 _]
                      frame False {
                        n778 = call "BLED1112-Rx Packet parser (RESPONSE-GAP).vi"("message package"=w1079) -> ("Packet OK"=w1078:bool)  [unwired: 2 in, 2 out]
                        n779 = case shown="참" w1078 {
                          frame False {
                          }
                          frame True {
                            n780 = local write "Packet Detect"(TRUE ("Packet Detect")) -> ()
                          }
                        }
                      }
                      frame True {
                      }
                    }
                  }
                  frame #4 {
                    # "Rx Packet parser (EVENT-Disconnected)"
                    n781 = local read "Packet Detect"() -> (w1082:bool)
                    n782 = case shown="거짓" w1082 {
                      tunnel: w1081 -> [w1084 _]
                      frame False {
                        n783 = call "BLED1112-Rx Packet parser (EVENT-Disconnected).vi"("message package"=w1084) -> ("Packet OK"=w1083:bool)  [unwired: 2 in, 2 out]
                        n784 = case shown="참" w1083 {
                          frame False {
                          }
                          frame True {
                            n785 = local write "Packet Detect"(TRUE ("Packet Detect")) -> ()
                            n786 = local write "Disconnected"(TRUE ("Packet Detect")) -> ()
                            n787 = local write "Comm con status 1"(FALSE ("Packet Detect")) -> ()
                            n788 = local write "Comm con 1"(FALSE ("Packet Detect")) -> ()
                            n789 = local write "ACT-Comm"(FALSE ("Packet Detect")) -> ()
                            n790 = local read "Disconnection ocurrence"() -> (w1085:refnum<k4>)
                            n791 = disable-structure shown="비활성화" {
                              frame Disabled {
                                n792 = One Button Dialog(message="BLE Disconnected!" ("메시지")) -> ()  [unwired: 1 in, 1 out]
                              }
                              frame Enabled {
                              }
                            }
                            n793 = Set Occurrence(w1085) -> ()
                          }
                        }
                      }
                      frame True {
                      }
                    }
                  }
                  frame #5 {
                    # "Rx Packet parser (Get Rssi))"
                    n794 = local read "Packet Detect"() -> (w1093:bool)
                    n795 = case shown="거짓" w1093 {
                      tunnel: w1092 -> [w1096 _]
                      frame False {
                        n796 = call "BLED1112-Rx Packet parser (Get Rssi).vi"("message package"=w1096) -> ("Packet OK"=w1095:bool, "Data Structure"=w1094:T41)  [unwired: 2 in, 1 out]
                        n797 = case shown="참" w1095 {
                          tunnel: w1094 -> [_ w1098]
                          frame False {
                          }
                          frame True {
                            n798 = local write "Packet Detect"(TRUE ("Packet Detect")) -> ()
                            n799 = Unbundle By Name(w1098) -> ("rssi"=→"BLE RSSI buf":i16)
                          }
                        }
                      }
                      frame True {
                      }
                    }
                  }
                }
                n800 = disable-structure shown="비활성화" {
                  frame Disabled {
                    n801 = local write "42 Tx"(FALSE ("불리언 6")) -> ()
                    n802 = local write "42 Tx"(FALSE ("불리언 6")) -> ()
                  }
                  frame Enabled {
                  }
                }
              }
            }
          }
        }
        n803 = Wait Until Next ms Multiple(millisecond multiple=u32 1 ("ms 배수")) -> ()  [unwired: 1 out]
        n804 = local read "stop"() -> (w414:bool)
      }
      n805 = while {
        stop <- w1126 stop-if-true
        # "If the value has changed Data Transfer Flag = On"
        # "Event"
        n806 = event shown="[1] \"PWR OFF\": 값 변경" {
          selector: _ -> [_ _ _ _ _ _ _]
          dyn-events: _ -> [_ _ _ _ _ _ _]
          timeout: 50 -> [_ _ _ _ _ _ _]
          event Timeout {
            n807 = event-data() -> ()  [unwired: 3 out]
          }
          event "PWR OFF": Value Change {
            n808 = event-data() -> ("NewVal"=w1127:bool)  [unwired: 1 out]
            n809 = case shown="참" w1127 {
              frame False {
              }
              frame True {
                n810 = stacked-sequence {
                  frame #0 {
                    n811 = local write "Handle"(u8 15 ("Handle")) -> ()
                    n812 = local write "Data(h)"("DYSKIMr" ("Data(h)")) -> ()
                  }
                  frame #1 {
                    n813 = control-ref of="Send"() -> (w1131:refnum<vi>)
                    n814 = property class="Bool (엄격한)"(reference=w1131, "Value"=TRUE ("값(신호)")) -> ()  [unwired: 1 in, 2 out]
                  }
                  frame #2 {
                    n815 = Wait (ms)(milliseconds to wait=u32 200 ("대기 시간(ms)")) -> ()  [unwired: 1 out]
                  }
                  frame #3 {
                    n816 = control-ref of="Comm con 1"() -> (w1133:refnum<vi>)
                    n817 = property class="Bool (엄격한)"(reference=w1133, "Val(Sgnl)"=FALSE ("값(신호)")) -> ()  [unwired: 1 in, 2 out]
                  }
                  frame #4 {
                    n818 = control-ref of="PWR OFF"() -> (w1135:refnum<vi>)
                    n819 = property class="Bool (엄격한)"(reference=w1135, "Val(Sgnl)"=FALSE ("값(신호)")) -> ()  [unwired: 1 in, 2 out]
                  }
                }
              }
            }
          }
          event Key Down {
            # "Ctrl + 1"
            n820 = event-data() -> ("Char"=w1144:i16, "VKey"=w1142:T28, "Mods"=w1146:cluster{"Num Pad":bool, "Menu Key":bool})  [unwired: 6 out]
            n821 = Unbundle By Name(w1146) -> ("Menu Key"=w1138:bool)
            n822 = Equal?(x=eventvkey."ASCII" ("V 키"), y=w1142) -> (x = y?=w1140:bool)
            n823 = Equal?(x=i16 49 ("문자"), y=w1144) -> (x = y?=w1141:bool)
            n824 = And(x=w1141, y=w1140) -> (x .and. y?=w1139:bool)
            n825 = And(x=w1139, y=w1138) -> (x .and. y?=w1137:bool)
            n826 = case shown="참" w1137 {
              frame False {
              }
              frame True {
                n827 = local write "Maximize window"(TRUE ("창크게")) -> ()
              }
            }
          }
          event "Comm con 1": Value Change {
            n828 = event-data() -> ("NewVal"=w1148:bool)  [unwired: 6 out]
            n829 = case shown="참" w1148 {
              frame False {
                # "BLE Close"
                n830 = local write "Port open 1"(FALSE) -> ()
                n831 = local write "Port close 1"(TRUE) -> ()
              }
              frame True {
                # "BLE Open"
                n832 = local write "Port open 1"(TRUE) -> ()
                n833 = local write "Port close 1"(FALSE) -> ()
              }
            }
          }
          event "Setting load": Value Change {
            n834 = event-data() -> ("NewVal"=w1153:bool)  [unwired: 6 out]
            n835 = case shown="참" w1153 {
              frame False {
              }
              frame True {
                n836 = local write "Setting load(led)"(TRUE ("Power On Flag")) -> ()
              }
            }
          }
          event "Data Logging": Value Change {
            n837 = event-data() -> ("OldVal"=w1155:bool)  [unwired: 6 out]
            n838 = stacked-sequence {
              seq-local: [w1158 _ _] -> [_ w1163 _]
              tunnel: w1155 -> [w1159 _ _]
              frame #0 {
                n839 = Equal?(x=w1159, y=FALSE) -> (x = y?=w1158:bool)
                n840 = case shown="거짓" w1158 {
                  tunnel: [File_Control_mode."Close" ("Mode") File_Control_mode."Open" ("Mode")] -> w1157
                  frame False {
                  }
                  frame True {
                  }
                }
                n841 = control-ref of="Log no"() -> (w1156:refnum<vi>)
                n842 = call "File_Interface.vi"("Mode"=w1157, "Log no"=w1156) -> ()  [unwired: 9 in, 1 out]
              }
              frame #1 {
                n843 = control-ref of="File Path Done"() -> (w1164:refnum<vi>)
                n844 = property class="Bool (엄격한)"(reference=w1164, "Value"=w1163) -> ()  [unwired: 1 in, 2 out]
              }
              frame #2 {
                n845 = Tick Count (ms)() -> (millisecond timer value=w1165:u32)
                n846 = local write "Timer-ble log"(w1165) -> ()
              }
            }
          }
          event Panel Close? {
            n847 = event-data() -> ()  [unwired: 5 out]
            n848 = stacked-sequence {
              frame #0 {
                n849 = local read "Disconnection ocurrence"() -> (w1168:refnum<k4>)
                n850 = Set Occurrence(w1168) -> ()
              }
              frame #1 {
                n851 = Wait (ms)(milliseconds to wait=u32 500 ("대기 시간(ms)")) -> ()  [unwired: 1 out]
              }
              frame #2 {
                n852 = local read "Disconnection ocurrence"() -> (w1170:refnum<k4>)
                n853 = Set Occurrence(w1170) -> ()
              }
            }
            n854 = local write "stop"(TRUE ("stop")) -> ()
            n855 = event-data("Discard?"=TRUE ("stop")) -> ()  [unwired: 1 in, 1 out]
          }
        }
        n856 = local read "stop"() -> (w1126:bool)
      }
      n857 = while {
        stop <- w1109 stop-if-true
        # "Load test-one time"
        n858 = stacked-sequence {
          frame #0 {
            n859 = local read "Force Set"() -> (w1111:bool)
            n860 = case shown="참" w1111 {
              frame False {
              }
              frame True {
                n861 = stacked-sequence {
                  frame #0 {
                    n862 = local read "Port-FTS"() -> (w1115:refnum<visa-resource-name>)
                    n863 = local read "Load(lb)"() -> (w1114:dbl)
                    n864 = call "_Serial_Mark10-Control (Press Config).vi"("FTS Operation state"=T27 "Start pressure control" ("FTS 제어 상태"), "Press Setting(lb)"=w1114, "Serial Port"=w1115) -> ("Communication is normal"=w1113:bool)  [unwired: 2 out]
                    n865 = case shown="거짓" w1113 {
                      frame False {
                        n866 = One Button Dialog(message="Can't find equipment!" ("메시지")) -> ()  [unwired: 1 in, 1 out]
                      }
                      frame True {
                      }
                    }
                  }
                  frame #1 {
                    n867 = local write "Force Set"(FALSE ("Force Set")) -> ()
                  }
                }
              }
            }
          }
          frame #1 {
            n868 = local read "Head Up"() -> (w1118:bool)
            n869 = case shown="참" w1118 {
              frame False {
              }
              frame True {
                n870 = stacked-sequence {
                  frame #0 {
                    n871 = local read "Port-FTS"() -> (w1122:refnum<visa-resource-name>)
                    n872 = local read "Load(lb)"() -> (w1121:dbl)
                    n873 = call "_Serial_Mark10-Control (Press Config).vi"("FTS Operation state"=T27 "Move Header Up", "Press Setting(lb)"=w1121, "Serial Port"=w1122) -> ("Communication is normal"=w1120:bool)  [unwired: 2 out]
                    n874 = case shown="거짓" w1120 {
                      frame False {
                        n875 = One Button Dialog(message="Can't find equipment!" ("메시지")) -> ()  [unwired: 1 in, 1 out]
                      }
                      frame True {
                      }
                    }
                  }
                  frame #1 {
                    n876 = local write "Head Up"(FALSE ("Force Set")) -> ()
                  }
                }
              }
            }
          }
        }
        n877 = Wait Until Next ms Multiple(millisecond multiple=u32 300 ("ms 배수")) -> ()  [unwired: 1 out]
        n878 = local read "stop"() -> (w1109:bool)
      }
      n879 = while {
        stop <- w1104 stop-if-true
        # "test-LED blink"
        n880 = local read "Force Set"() -> (w1102:bool)
        n881 = local read "Test Start"() -> (w1103:bool)
        n882 = local read "Head Up"() -> (w1100:bool)
        n883 = Compound Arithmetic op=OR ("복합 연산")(w1103, w1102, w1100) -> (w1101:bool)
        n884 = case shown="참" w1101 {
          frame False {
            n885 = local write "FTS Testing"(FALSE ("FTS 시험 진행")) -> ()
          }
          frame True {
            n886 = local read "FTS Testing"() -> (w1108:bool)
            n887 = Not(x=w1108) -> (.not. x?=w1107:bool)
            n888 = local write "FTS Testing"(w1107) -> ()
          }
        }
        n889 = Wait Until Next ms Multiple(millisecond multiple=u32 300 ("ms 배수")) -> ()  [unwired: 1 out]
        n890 = local read "stop"() -> (w1104:bool)
      }
      n891 = while {
        i -> [w1171]
        stop <- w1173 stop-if-true
        n892 = stacked-sequence {
          tunnel: w1171 -> [_ w1248 _ _ _ _ _ _ _ _ _ _ _ _ _ _]
          frame #0 {
            # "Connection of Communication - BLE"
            n893 = local read "Port close 1"() -> (w1175:bool)
            n894 = local read "Port open 1"() -> (w1174:bool)
            n895 = case shown="참" w1174 {
              frame False {
              }
              frame True {
                # "Connection of Communication"
                n896 = stacked-sequence {
                  frame #0 {
                    # "BLE Buffer Clear"
                    # "Initialize"
                    n897 = call "SUB-BLE Rx data Clear.vi"() -> ()  [unwired: 6 in]
                    n898 = Tick Count (ms)() -> (millisecond timer value=w1177:u32)
                    n899 = local write "ACT-Comm"(TRUE ("ACT-RS422")) -> ()
                    n900 = local write "Full ROM data"(FALSE ("Full ROM data")) -> ()
                    n901 = local write "Port open 1"(FALSE) -> ()
                    n902 = Initialize Array(T19 {"RxOK"=FALSE, "ROM Data"=[], "Index"=0} ("클러스터"), 9 ("차원 크기")) -> (w1181:T12)
                    n903 = local write "Data trx(led)"(TRUE ("Rx")) -> ()
                    n904 = local write "Rx ROM-log"("" ("문자열-Rx ROM")) -> ()
                    n905 = local write "Timer-ble log"(w1177) -> ()
                    n906 = local write "ROM Data"(w1181) -> ()
                    n907 = local write "status string"("Communication connection attempt.." ("status string")) -> ()
                  }
                  frame #1 {
                    n908 = local read "Port-set 1"() -> (w1187:refnum<visa-resource-name>)
                    n909 = call "_Serial Port-Initialize.vi"("baud rate"=u32 115200, "Serial Port"=w1187) -> ("Serial Port 2"=w1189:refnum<visa-resource-name>, "Normal"=w1191:bool)  [unwired: 2 in]
                    n910 = local write "Port-act 1"(w1187) -> ()
                    n911 = call "SUB_Write_GEN4_Init_data_V2_0_1.vi"("Port-act 1"=w1187, "Mode"=enum16{"Save Flash", "Visa save"}."Visa save") -> ()  [unwired: 25 in, 1 out]
                    n912 = VISA Close(VISA resource name=w1189) -> (error out=w1188:errorcluster)  [unwired: 1 in]
                    n913 = case shown="참" w1191 {
                      tunnel: w1187 -> [_ w1200]
                      tunnel: w1188 -> [_ _]
                      frame False {
                        n914 = local write "Comm con status 1"(FALSE ("Connected")) -> ()
                        n915 = local write "Comm con 1"(FALSE ("보드 통신 연결 1")) -> ()
                        n916 = local write "Rx-mon"(TRUE ("수신 실패(T) 2")) -> ()
                        n917 = local write "RxD"("Can not find COM port" ("status string")) -> ()
                      }
                      frame True {
                        n918 = call "SUB-BLE SCAN.vi"("Port-set 1"=w1200) -> ("Device Name"=→"Device Name":string, "Connection Status"=w1196:T6, "Connected"=w1199:bool)  [unwired: 2 in]
                        "Connection Status" <- w1196
                        n919 = Not(x=w1199) -> (.not. x?=w1198:bool)
                        n920 = local write "Rx-mon"(w1198) -> ()
                        n921 = case shown="거짓" w1198 {
                          tunnel: w1196 -> [_ w1208]
                          frame True {
                            # "수신 데이터 에러 상태"
                            n922 = local read "Port-act 1"() -> (w1204:refnum<visa-resource-name>)
                            n923 = VISA Close(VISA resource name=w1204) -> ()  [unwired: 1 in, 1 out]
                            n924 = local write "Comm con status 1"(FALSE ("Connected")) -> ()
                            n925 = local write "*Board ID1"("None...." ("*Board ID")) -> ()
                            n926 = local write "Comm con 1"(FALSE ("보드 통신 연결 1")) -> ()
                            n927 = local write "Rx-mon"(TRUE ("수신 실패(T) 2")) -> ()
                          }
                          frame False {
                            w1210 = T10 {"Left Wing-A, C1/C0"=0.0, "Left Wing-B, C2/C0"=0.0, "Left Wing-C, C3/C0"=0.0, "Right Wing-A, C4/C0"=0.0, "Right Wing-B, C5/C0"=0.0, "Right Wing-C, C6/C0"=0.0} ("CDC data")
                            w1209 = T11 {"Gyroscope X"=0.0, "Gyroscope Y"=0.0, "Gyroscope Z"=0.0, "Accelerometer X"=0.0, "Accelerometer Y"=0.0, "Accelerometer Z"=0.0} ("IMU data")
                            # "Received data normal"
                            n928 = stacked-sequence {
                              tunnel: w1208 -> [_ w1225 w1227 _]
                              frame #0 {
                                # "BLE 버퍼 클리어"
                                n929 = call "SUB-BLE Rx data Clear.vi"() -> ()  [unwired: 6 in]
                                n930 = Wait Until Next ms Multiple(millisecond multiple=u32 500 ("ms 타이머 값")) -> ()  [unwired: 1 out]
                              }
                              frame #1 {
                                # "Data transmission\n- Handle/0x01"
                                n931 = local read "Port-act 1"() -> (w1224:refnum<visa-resource-name>)
                                n932 = Tick Count (ms)() -> (millisecond timer value=w1223:u32)
                                n933 = Build Array(u16 1 ("Handle"), u16 0 ("Handle")) -> (w1222:u16[])
                                n934 = local write "ms timer 4"(w1223) -> ()
                                n935 = call-poly "ble_write_by_handle.vi"("Connection Status"=w1225, "Handle"=u16 12, "data (uint8array)"=w1222, "COM Bluegiga in"=w1224) -> ()  [unwired: 6 in, 2 out]
                              }
                              frame #2 {
                                # "데이터 전송\n- 핸들/0x01"
                                n936 = local read "Port-act 1"() -> (w1232:refnum<visa-resource-name>)
                                n937 = Tick Count (ms)() -> (millisecond timer value=w1231:u32)
                                n938 = Build Array(u16 1 ("Handle"), u16 0 ("Handle")) -> (w1230:u16[])
                                n939 = local write "ms timer 4"(w1231) -> ()
                                n940 = call-poly "ble_write_by_handle.vi"("Connection Status"=w1227, "Handle"=u16 16, "data (uint8array)"=w1230, "COM Bluegiga in"=w1232) -> ()  [unwired: 6 in, 2 out]
                              }
                              frame #3 {
                                n941 = local write "Comm con status 1"(TRUE ("Connected")) -> ()
                              }
                            }
                            n942 = local write "*Board ID1"("" ("*Board ID")) -> ()
                            n943 = local write "RxD"("Connection. OK....." ("status string")) -> ()
                            n944 = local write "Setting load(led)"(FALSE ("Power On Flag")) -> ()
                            n945 = local write "Comm err cnt 1"(0 ("통신에러카운트")) -> ()
                            n946 = local write "Clear graph 1"(TRUE ("그래프 지우기")) -> ()
                            n947 = local write "Clear graph 2"(TRUE ("그래프 지우기")) -> ()
                            n948 = local write "Data Log"("" ("Data Log")) -> ()
                            n949 = local write "Data_mon(h)"("" ("Data_mon")) -> ()
                            n950 = local write "Comm con 1"(TRUE ("포트 연결")) -> ()
                            n951 = local write "CDC Offet"(w1210) -> ()
                            n952 = local write "CDC data"(w1210) -> ()
                            n953 = local write "IMU data"(w1209) -> ()
                            n954 = local write "IMU Offet"(w1209) -> ()
                          }
                        }
                      }
                    }
                  }
                  frame #2 {
                    n955 = local write "ACT-Comm"(FALSE ("ACT-RS422")) -> ()
                    n956 = local write "Data trx(led)"(FALSE ("Rx")) -> ()
                  }
                }
              }
            }
            n957 = case shown="참" w1175 {
              frame False {
              }
              frame True {
                # "END of BLE Communication"
                # "포트 닫기"
                n958 = local write "Port close 1"(FALSE ("포트닫기 1")) -> ()
                n959 = local write "Comm con status 1"(FALSE ("Connected")) -> ()
                n960 = local write "*Board ID1"("None...." ("*Board ID")) -> ()
                n961 = local write "ACT-Comm"(FALSE ("ACT-RS422")) -> ()
                n962 = local write "status string"("Close communication port." ("status string")) -> ()
                n963 = local write "Comm con 1"(FALSE ("보드 통신 연결 1")) -> ()
                n964 = local read "Port-act 1"() -> (w1236:refnum<visa-resource-name>)
                n965 = local read "Connection Status"() -> (w1241:T6)
                n966 = call "_Serial_buf clear.vi"("Serial Port"=w1236) -> ("에러 출력"=w1239:errorcluster, "Serial Port 2"=w1240:refnum<visa-resource-name>)  [unwired: 3 in]
                n967 = call "ble_disconnect_device.vi"("Connection Status"=w1241, "error in (no error)"=w1239, "COM Bluegiga in"=w1240) -> ("error out"=w1238:errorcluster, "COM Bluegiga out"=w1237:refnum<visa-resource-name>)  [unwired: 7 in]
                n968 = VISA Close(VISA resource name=w1237, error in (no error)=w1238) -> ()  [unwired: 1 out]
              }
            }
          }
          frame #1 {
            # "#BLE_Packet_data_process"
            # "BLE RX Packet data processing"
            n969 = local read "Comm con status 1"() -> (w1249:bool)
            n970 = case shown="참" w1249 {
              tunnel: w1248 -> [_ w1260]
              frame False {
              }
              frame True {
                w1252 = 80 ("y")
                n971 = call "SUB-BLE Rx data (Mon)-Classify.vi"() -> ("data out"=w1259:u8[], "Rx-set"=w1257:bool, "Rx-debug"=w1256:bool, "Rx-mon"=w1258:bool, "Packet No."=w1255:i32)  [unwired: 5 in]
                n972 = local write "Packet No."(w1255) -> ()
                n973 = stacked-sequence {
                  tunnel: w1259 -> [w1312 w1334 w1355]
                  tunnel: w1258 -> [w1311 _ _]
                  tunnel: w1257 -> [_ _ w1356]
                  tunnel: w1256 -> [_ w1335 _]
                  frame #0 {
                    # "Monitoring Data"
                    n974 = Array Subset(array=w1312, index=1 ("인덱스"), length=35 ("길이")) -> (w1264:u8[])
                    n975 = Index Array(array=w1264, index=34 ("인덱스")) -> (element=w1284:u8)
                    n976 = Index Array(array=w1264, index #1=0 ("인덱스"), index #6=5 ("인덱스"), index #11=10 ("인덱스"), index #16=15 ("인덱스"), index #21=20 ("인덱스"), index #26=25 ("인덱스"), index #31=30 ("인덱스")) -> (element #1=w1303:u8, element #2=w1302:u8, element #3=w1301:u8, element #4=w1300:u8, element #5=w1299:u8, element #6=w1298:u8, element #7=w1297:u8, element #8=w1296:u8, element #9=w1295:u8, element #10=w1294:u8, element #11=w1293:u8, element #12=w1292:u8, element #13=w1291:u8, element #14=w1290:u8, element #15=w1289:u8, element #16=w1288:u8, element #17=w1283:u8, element #18=w1279:u8, element #19=w1278:u8, element #20=w1277:u8, element #21=w1276:u8, element #22=w1275:u8, element #23=w1274:u8, element #24=w1273:u8, element #25=w1272:u8, element #26=w1271:u8, element #27=w1270:u8, element #28=w1269:u8, element #29=w1268:u8, element #30=w1267:u8, element #31=w1266:u8, element #32=w1265:u8, element #33=w1263:u8, element #34=w1262:u8)  [unwired: 27 in]
                    n977 = Compound Arithmetic op=ADD(w1303, w1302, w1301, w1300, w1299, w1298, w1297, w1296, w1295, w1294, w1293, w1292, w1291, w1290, w1289, w1288, w1283, w1279, w1278, w1277, w1276, w1275, w1274, w1273, w1272, w1271, w1270, w1269, w1268, w1267, w1266, w1265, w1263, w1262) -> (w1286:u8)
                    n978 = Subtract(x=u8 255, y=w1286) -> (x-y=w1285:u8)
                    "x-y" <- w1285
                    n979 = Equal?(x=w1285, y=w1284) -> (x = y?=w1261:bool)
                    n980 = case shown="참" w1261 {
                      tunnel: w1312 -> [_ w1314]
                      tunnel: w1311 -> [_ w1313]
                      frame False {
                      }
                      frame True {
                        n981 = case shown="참" w1313 {
                          tunnel: w1314 -> [_ w1321]
                          frame False {
                          }
                          frame True {
                            # "Monitoring data reception complete"
                            n982 = local read "ms timer"() -> (w1330:u32)
                            n983 = local write "Rx-mon"(TRUE ("Rx-mon")) -> ()
                            n984 = local write "Rx-ROM"(FALSE ("Rx-ROM")) -> ()
                            n985 = local write "Rx-debug"(FALSE ("Rx-debug")) -> ()
                            n986 = Tick Count (ms)() -> (millisecond timer value=w1329:u32)
                            n987 = call <vilib>:"Space Constant.vi"() -> ("String"=w1324:string)
                            n988 = Subtract(x=w1329, y=w1330) -> (x-y=w1327:u32)
                            n989 = local write "BLE Packet (mon)"(w1321) -> ()
                            n990 = Array To Spreadsheet String(delimiter (Tab)=w1324, array=w1321, 3:"%02X" ("포맷 문자열")) -> (spreadsheet string=w1322:string)
                            n991 = local write "ms timer"(w1329) -> ()
                            n992 = local write "status string"("Receive a monitoring data..." ("status string")) -> ()
                            n993 = Format Into String(format string="[%d ms] " ("포맷 문자열"), w1327) -> (resulting string=w1326:string)  [unwired: 2 in, 1 out]
                            n994 = local read "ms timer 2"() -> (w1318:u32)
                            n995 = Tick Count (ms)() -> (millisecond timer value=w1317:u32)
                            n996 = Concatenate Strings(w1326, w1322) -> (w1325:string)
                            n997 = Subtract(x=w1317, y=w1318) -> (x-y=w1316:u32)
                            n998 = case shown="150.." w1316 {
                              tunnel: w1325 -> [_ w1333]
                              frame 0, Default {
                              }
                              frame 150.. {
                                n999 = Tick Count (ms)() -> (millisecond timer value=w1332:u32)
                                n1000 = local write "RxD"(w1333) -> ()
                                n1001 = local write "ms timer 2"(w1332) -> ()
                              }
                            }
                          }
                        }
                      }
                    }
                  }
                  frame #1 {
                    # "Debugging Data"
                    n1002 = case shown="참" w1335 {
                      tunnel: w1334 -> [_ w1342]
                      frame False {
                      }
                      frame True {
                        # "debugging Data reception complete"
                        n1003 = local read "ms timer"() -> (w1351:u32)
                        n1004 = local write "Rx-mon"(FALSE ("Rx-mon")) -> ()
                        n1005 = local write "Rx-ROM"(FALSE ("Rx-ROM")) -> ()
                        n1006 = local write "Rx-debug"(TRUE ("Rx-debug")) -> ()
                        n1007 = Tick Count (ms)() -> (millisecond timer value=w1350:u32)
                        n1008 = call <vilib>:"Space Constant.vi"() -> ("String"=w1345:string)
                        n1009 = Subtract(x=w1350, y=w1351) -> (x-y=w1348:u32)
                        n1010 = local write "BLE Packet (mon)"(w1342) -> ()
                        n1011 = Array To Spreadsheet String(delimiter (Tab)=w1345, array=w1342, 3:"%02X" ("포맷 문자열")) -> (spreadsheet string=w1343:string)
                        n1012 = local write "ms timer"(w1350) -> ()
                        n1013 = local write "status string"("Receive a debugging data..." ("status string")) -> ()
                        n1014 = Format Into String(format string="[%d ms] " ("포맷 문자열"), w1348) -> (resulting string=w1347:string)  [unwired: 2 in, 1 out]
                        n1015 = local read "ms timer 2"() -> (w1339:u32)
                        n1016 = Tick Count (ms)() -> (millisecond timer value=w1338:u32)
                        n1017 = Concatenate Strings(w1347, w1343) -> (w1346:string)
                        n1018 = Subtract(x=w1338, y=w1339) -> (x-y=w1337:u32)
                        n1019 = case shown="150.." w1337 {
                          tunnel: w1346 -> [_ w1354]
                          frame 0, Default {
                          }
                          frame 150.. {
                            n1020 = Tick Count (ms)() -> (millisecond timer value=w1353:u32)
                            n1021 = local write "RxD"(w1354) -> ()
                            n1022 = local write "ms timer 2"(w1353) -> ()
                          }
                        }
                      }
                    }
                  }
                  frame #2 {
                    # "Init data"
                    n1023 = case shown="참" w1356 {
                      tunnel: w1355 -> [_ w1357]
                      frame False {
                      }
                      frame True {
                        n1024 = local write "Rx-mon"(FALSE ("수신 실패(T) 1")) -> ()
                        n1025 = local write "Rx-debug"(FALSE ("Rx-debug")) -> ()
                        n1026 = local write "Rx-ROM"(TRUE ("Rx-ROM")) -> ()
                        n1027 = stacked-sequence {
                          tunnel: w1357 -> [w1369 _ _]
                          frame #0 {
                            # "Check data input status"
                            n1028 = call "SUB-BLE Rx data (Mon)-ROM.vi"("data in"=w1369) -> ("data Out"=w1362:u8[], "Index"=w1361:u8)  [unwired: 3 in]
                            n1029 = property on="ROM Data" class="Arr (엄격한)"("Index Values"=u32[] [] ("인덱스 값")) -> ()  [unwired: 2 in, 2 out]
                            n1030 = for {
                              N: 9 -> [_]
                              tunnel: w1362 -> [w1397]
                              tunnel: w1361 -> [w1396]
                              tunnel: [w1395] -> w1366 mode=indexing
                              n1031 = case shown="..0" w1396 {
                                tunnel: w1397 -> [w1400 w1427 w1455 w1486 w1514 w1542 w1570 w1598 w1645]
                                tunnel: [w1398 w1426 w1454 w1482 w1510 w1538 w1566 w1594 w1622] -> w1395
                                frame ..0 {
                                n1032 = Index Array(array=w1400, index #1=0 ("인덱스"), index #6=5 ("인덱스"), index #11=10 ("인덱스"), index #16=15 ("인덱스")) -> (element #1=w1420:u8, element #2=w1419:u8, element #3=w1418:u8, element #4=w1417:u8, element #5=w1416:u8, element #6=w1415:u8, element #7=w1414:u8, element #8=w1413:u8, element #9=w1412:u8, element #10=w1411:u8, element #11=w1410:u8, element #12=w1409:u8, element #13=w1408:u8, element #14=w1407:u8, element #15=w1406:u8, element #16=w1405:u8, element #17=w1399:u8)  [unwired: 13 in]
                                n1033 = Index Array(array=w1400, index=17 ("인덱스")) -> (element=w1401:u8)
                                n1034 = Compound Arithmetic op=ADD(w1420, w1419, w1418, w1417, w1416, w1415, w1414, w1413, w1412, w1411, w1410, w1409, w1408, w1407, w1406, w1405, w1399) -> (w1403:u8)
                                n1035 = Subtract(x=u8 255, y=w1403) -> (x-y=w1402:u8)
                                n1036 = Equal?(x=w1402, y=w1401) -> (x = y?=w1398:bool)
                                }
                                frame 1 {
                                n1037 = Index Array(array=w1427, index #1=0 ("인덱스"), index #6=5 ("인덱스"), index #11=10 ("인덱스"), index #16=15 ("인덱스")) -> (element #1=w1448:u8, element #2=w1447:u8, element #3=w1446:u8, element #4=w1445:u8, element #5=w1444:u8, element #6=w1443:u8, element #7=w1442:u8, element #8=w1441:u8, element #9=w1440:u8, element #10=w1439:u8, element #11=w1438:u8, element #12=w1437:u8, element #13=w1436:u8, element #14=w1435:u8, element #15=w1434:u8, element #16=w1433:u8, element #17=w1432:u8)  [unwired: 13 in]
                                n1038 = Index Array(array=w1427, index=17 ("인덱스")) -> (element=w1431:u8)
                                n1039 = Compound Arithmetic op=ADD(w1448, w1447, w1446, w1445, w1444, w1443, w1442, w1441, w1440, w1439, w1438, w1437, w1436, w1435, w1434, w1433, w1432) -> (w1429:u8)
                                n1040 = Subtract(x=u8 255, y=w1429) -> (x-y=w1428:u8)
                                n1041 = Equal?(x=w1428, y=w1431) -> (x = y?=w1426:bool)
                                }
                                frame 2 {
                                n1042 = Index Array(array=w1455, index #1=0 ("인덱스"), index #6=5 ("인덱스"), index #11=10 ("인덱스"), index #16=15 ("인덱스")) -> (element #1=w1476:u8, element #2=w1475:u8, element #3=w1474:u8, element #4=w1473:u8, element #5=w1472:u8, element #6=w1471:u8, element #7=w1470:u8, element #8=w1469:u8, element #9=w1468:u8, element #10=w1467:u8, element #11=w1466:u8, element #12=w1465:u8, element #13=w1464:u8, element #14=w1463:u8, element #15=w1462:u8, element #16=w1461:u8, element #17=w1460:u8)  [unwired: 13 in]
                                n1043 = Index Array(array=w1455, index=17 ("인덱스")) -> (element=w1459:u8)
                                n1044 = Compound Arithmetic op=ADD(w1476, w1475, w1474, w1473, w1472, w1471, w1470, w1469, w1468, w1467, w1466, w1465, w1464, w1463, w1462, w1461, w1460) -> (w1457:u8)
                                n1045 = Subtract(x=u8 255, y=w1457) -> (x-y=w1456:u8)
                                n1046 = Equal?(x=w1456, y=w1459) -> (x = y?=w1454:bool)
                                }
                                frame 3 {
                                n1047 = Index Array(array=w1486, index #1=0 ("인덱스"), index #6=5 ("인덱스"), index #11=10 ("인덱스"), index #16=15 ("인덱스")) -> (element #1=w1504:u8, element #2=w1503:u8, element #3=w1502:u8, element #4=w1501:u8, element #5=w1500:u8, element #6=w1499:u8, element #7=w1498:u8, element #8=w1497:u8, element #9=w1496:u8, element #10=w1495:u8, element #11=w1494:u8, element #12=w1493:u8, element #13=w1492:u8, element #14=w1491:u8, element #15=w1490:u8, element #16=w1489:u8, element #17=w1488:u8)  [unwired: 13 in]
                                n1048 = Index Array(array=w1486, index=17 ("인덱스")) -> (element=w1487:u8)
                                n1049 = Compound Arithmetic op=ADD(w1504, w1503, w1502, w1501, w1500, w1499, w1498, w1497, w1496, w1495, w1494, w1493, w1492, w1491, w1490, w1489, w1488) -> (w1484:u8)
                                n1050 = Subtract(x=u8 255, y=w1484) -> (x-y=w1483:u8)
                                n1051 = Equal?(x=w1483, y=w1487) -> (x = y?=w1482:bool)
                                }
                                frame 4 {
                                n1052 = Index Array(array=w1514, index #1=0 ("인덱스"), index #6=5 ("인덱스"), index #11=10 ("인덱스"), index #16=15 ("인덱스")) -> (element #1=w1532:u8, element #2=w1531:u8, element #3=w1530:u8, element #4=w1529:u8, element #5=w1528:u8, element #6=w1527:u8, element #7=w1526:u8, element #8=w1525:u8, element #9=w1524:u8, element #10=w1523:u8, element #11=w1522:u8, element #12=w1521:u8, element #13=w1520:u8, element #14=w1519:u8, element #15=w1518:u8, element #16=w1517:u8, element #17=w1516:u8)  [unwired: 13 in]
                                n1053 = Index Array(array=w1514, index=17 ("인덱스")) -> (element=w1515:u8)
                                n1054 = Compound Arithmetic op=ADD(w1532, w1531, w1530, w1529, w1528, w1527, w1526, w1525, w1524, w1523, w1522, w1521, w1520, w1519, w1518, w1517, w1516) -> (w1512:u8)
                                n1055 = Subtract(x=u8 255, y=w1512) -> (x-y=w1511:u8)
                                n1056 = Equal?(x=w1511, y=w1515) -> (x = y?=w1510:bool)
                                }
                                frame 5 {
                                n1057 = Index Array(array=w1542, index #1=0 ("인덱스"), index #6=5 ("인덱스"), index #11=10 ("인덱스"), index #16=15 ("인덱스")) -> (element #1=w1560:u8, element #2=w1559:u8, element #3=w1558:u8, element #4=w1557:u8, element #5=w1556:u8, element #6=w1555:u8, element #7=w1554:u8, element #8=w1553:u8, element #9=w1552:u8, element #10=w1551:u8, element #11=w1550:u8, element #12=w1549:u8, element #13=w1548:u8, element #14=w1547:u8, element #15=w1546:u8, element #16=w1545:u8, element #17=w1544:u8)  [unwired: 13 in]
                                n1058 = Index Array(array=w1542, index=17 ("인덱스")) -> (element=w1543:u8)
                                n1059 = Compound Arithmetic op=ADD(w1560, w1559, w1558, w1557, w1556, w1555, w1554, w1553, w1552, w1551, w1550, w1549, w1548, w1547, w1546, w1545, w1544) -> (w1540:u8)
                                n1060 = Subtract(x=u8 255, y=w1540) -> (x-y=w1539:u8)
                                n1061 = Equal?(x=w1539, y=w1543) -> (x = y?=w1538:bool)
                                }
                                frame 6 {
                                n1062 = Index Array(array=w1570, index #1=0 ("인덱스"), index #6=5 ("인덱스"), index #11=10 ("인덱스"), index #16=15 ("인덱스")) -> (element #1=w1588:u8, element #2=w1587:u8, element #3=w1586:u8, element #4=w1585:u8, element #5=w1584:u8, element #6=w1583:u8, element #7=w1582:u8, element #8=w1581:u8, element #9=w1580:u8, element #10=w1579:u8, element #11=w1578:u8, element #12=w1577:u8, element #13=w1576:u8, element #14=w1575:u8, element #15=w1574:u8, element #16=w1573:u8, element #17=w1572:u8)  [unwired: 13 in]
                                n1063 = Index Array(array=w1570, index=17 ("인덱스")) -> (element=w1571:u8)
                                n1064 = Compound Arithmetic op=ADD(w1588, w1587, w1586, w1585, w1584, w1583, w1582, w1581, w1580, w1579, w1578, w1577, w1576, w1575, w1574, w1573, w1572) -> (w1568:u8)
                                n1065 = Subtract(x=u8 255, y=w1568) -> (x-y=w1567:u8)
                                n1066 = Equal?(x=w1567, y=w1571) -> (x = y?=w1566:bool)
                                }
                                frame 7 {
                                n1067 = Index Array(array=w1598, index #1=0 ("인덱스"), index #6=5 ("인덱스"), index #11=10 ("인덱스"), index #16=15 ("인덱스")) -> (element #1=w1616:u8, element #2=w1615:u8, element #3=w1614:u8, element #4=w1613:u8, element #5=w1612:u8, element #6=w1611:u8, element #7=w1610:u8, element #8=w1609:u8, element #9=w1608:u8, element #10=w1607:u8, element #11=w1606:u8, element #12=w1605:u8, element #13=w1604:u8, element #14=w1603:u8, element #15=w1602:u8, element #16=w1601:u8, element #17=w1600:u8)  [unwired: 13 in]
                                n1068 = Index Array(array=w1598, index=17 ("인덱스")) -> (element=w1599:u8)
                                n1069 = Compound Arithmetic op=ADD(w1616, w1615, w1614, w1613, w1612, w1611, w1610, w1609, w1608, w1607, w1606, w1605, w1604, w1603, w1602, w1601, w1600) -> (w1596:u8)
                                n1070 = Subtract(x=u8 255, y=w1596) -> (x-y=w1595:u8)
                                n1071 = Equal?(x=w1595, y=w1599) -> (x = y?=w1594:bool)
                                }
                                frame 8.. {
                                n1072 = Index Array(array=w1645, index #1=0 ("인덱스"), index #6=5 ("인덱스"), index #11=10 ("인덱스"), index #16=15 ("인덱스")) -> (element #1=w1643:u8, element #2=w1642:u8, element #3=w1641:u8, element #4=w1640:u8, element #5=w1639:u8, element #6=w1638:u8, element #7=w1637:u8, element #8=w1636:u8, element #9=w1635:u8, element #10=w1634:u8, element #11=w1633:u8, element #12=w1632:u8, element #13=w1631:u8, element #14=w1630:u8, element #15=w1629:u8, element #16=w1628:u8, element #17=w1627:u8)  [unwired: 13 in]
                                n1073 = Index Array(array=w1645, index=17 ("인덱스")) -> (element=w1626:u8)
                                n1074 = Compound Arithmetic op=ADD(w1643, w1642, w1641, w1640, w1639, w1638, w1637, w1636, w1635, w1634, w1633, w1632, w1631, w1630, w1629, w1628, w1627) -> (w1624:u8)
                                n1075 = Subtract(x=u8 255, y=w1624) -> (x-y=w1623:u8)
                                n1076 = Equal?(x=w1623, y=w1626) -> (x = y?=w1622:bool)
                                }
                              }
                            }
                            n1077 = Boolean Array To Number(Boolean array=w1366) -> (number=w1365:u32)
                            n1078 = Equal?(x=w1365, y=511) -> (x = y?=w1363:bool)
                            n1079 = case shown="참" w1363 {
                              tunnel: w1361 -> [_ w1374]
                              tunnel: w1361 -> [_ w1373]
                              tunnel: w1362 -> [_ w1372]
                              tunnel: w1361 -> [_ w1371]
                              frame False {
                                "recall-2" <- TRUE ("불리언 4")
                              }
                              frame True {
                                n1080 = local read "ROM Data"() -> (w1375:T12)
                                n1081 = Bundle By Name(cluster=T19 {"RxOK"=FALSE, "ROM Data"=[], "Index"=0} ("클러스터"), "RxOK"=TRUE ("Packet Detect"), "ROM Data"=w1372, "Index"=w1373) -> (w1377:T19)
                                n1082 = Replace Array Subset(array=w1375, new element=w1377, index=w1374) -> (w1388:T12)
                                n1083 = local read "Rx ROM-log"() -> (w1380:string)
                                n1084 = Format Into String(format string="[Packet ID]%02d  " ("포맷 문자열"), w1371) -> (resulting string=w1386:string)  [unwired: 2 in, 1 out]
                                n1085 = for {
                                tunnel: w1388 -> [w1394] mode=indexing
                                tunnel: [w1393] -> w1389 mode=indexing
                                n1086 = Unbundle By Name(w1394) -> ("RxOK"=w1393:bool)
                                }
                                n1087 = local write "ROM Data"(w1388) -> ()
                                n1088 = call <vilib>:"Space Constant.vi"() -> ("String"=w1387:string)
                                n1089 = Array To Spreadsheet String(delimiter (Tab)=w1387, array=w1372, 3:"%02X" ("포맷 문자열")) -> (spreadsheet string=w1384:string)
                                n1090 = Format Date/Time String(time format string (%c)="%H:%M:%S%3u>  " ("상태")) -> (date/time string=w1382:string)  [unwired: 2 in]
                                n1091 = Concatenate Strings(w1380, w1386, w1382, w1384) -> (w1381:string)
                                n1092 = Boolean Array To Number(Boolean array=w1389) -> (number=w1390:u32)
                                n1093 = local write "Rx ROM-log"(w1381) -> ()
                                n1094 = Equal?(x=w1390, y=u32 511) -> (x = y?=w1391:bool)
                                n1095 = local write "Full ROM data"(w1391) -> ()
                              }
                            }
                          }
                          frame #1 {
                            n1096 = control-ref of="ROM Data"() -> (w1651:refnum<vi>)
                            n1097 = control-ref of="ROM Table"() -> (w1650:refnum<vi>)
                            n1098 = call "SUB-ROM Data convert to table.vi"("ROM Table Ref"=w1650, "ROM Data Ref"=w1651) -> ()  [unwired: 2 in, 2 out]
                          }
                          frame #2 {
                            # "Setting Info Table update"
                            n1099 = property on="ROM Table" class="Tbl (엄격한)"() -> ("Column Headers[]"=w1661:string[], "Row Headers[]"=w1660:string[], "Value"=w1653:string[][])  [unwired: 2 in, 2 out]
                            n1100 = Index Array(array=w1653, index (col)=1 ("비활성화된 인덱스 (열)")) -> (element=w1657:string[])  [unwired: 1 in]
                            n1101 = for {
                              tunnel: w1657 -> [w1673] mode=indexing
                              shift-right: [w1668] -> w1655
                              shift-left: string[][] [] -> [w1667]
                              n1102 = Spreadsheet String To Array(delimiter (Tab)=" " ("구분 문자(탭)"), format string="%s" ("포맷 문자열"), spreadsheet string=w1673, array type (2D Dbl)=string[] []) -> (array=w1669:string[])
                              n1103 = Build Array (concatenate)(w1667, w1669) -> (w1668:string[][])
                            }
                            n1104 = Index Array(array=w1655, index (col)=0 ("비활성화된 인덱스 (열)")) -> (element=w1654:string[])  [unwired: 1 in]
                            n1105 = for {
                              tunnel: w1654 -> [w1666] mode=indexing
                              shift-right: [w1663] -> w1652
                              shift-left: w1653 -> [w1662]
                              i -> [w1664]
                              n1106 = Replace Array Subset(array=w1662, new element=w1666, index (row)=w1664, index (col)=1 ("비활성화된 인덱스 (열)")) -> (w1663:string[][])
                            }
                            n1107 = property on="ROM Table 2" class="Tbl (엄격한)"("Column Headers[]"=w1661, "Row Headers[]"=w1660, "Value"=w1652) -> ()  [unwired: 2 in, 2 out]
                          }
                        }
                      }
                    }
                  }
                }
                n1108 = Quotient & Remainder(x=w1260, y=w1252) -> (x-y*floor(x/y)=w1250:i32)  [unwired: 1 out]
                n1109 = Divide(x=w1252, y=2) -> (x/y=w1253:dbl)
                n1110 = Greater?(x=w1250, y=w1253) -> (0:w1251:bool)
                n1111 = local write "ACT-Comm"(w1251) -> ()
              }
            }
          }
          frame #2 {
            # "Monitoring Data"
            n1112 = local read "Rx-mon"() -> (w1674:bool)
            n1113 = case shown="참" w1674 {
              frame False {
              }
              frame True {
                # "#Processing Received Data"
                n1114 = local read "ms timer 3"() -> (w1679:u32)
                n1115 = local read "Update(ms)"() -> (w1675:u16)
                n1116 = Tick Count (ms)() -> (millisecond timer value=w1678:u32)
                n1117 = Subtract(x=w1678, y=w1679) -> (x-y=w1676:u32)
                n1118 = Greater Or Equal?(x=w1676, y=w1675) -> (x >= y?=w1677:bool)
                n1119 = case shown="참" w1677 {
                  frame False {
                  }
                  frame True {
                    n1120 = local read "BLE Packet (mon)"() -> (w1684:u8[])
                    n1121 = call "SUB-BLE Rx data (Mon)-CDC IMU.vi"("data in"=w1684) -> ("IMU data"=w1681:T11, "CDC data"=w1682:T10, "Bat"=w1680:u16, "*Board ID"=w1683:string)  [unwired: 4 in]
                    n1122 = stacked-sequence {
                      seq-local: [w1687 _ _ _ _ _] -> [_ _ w1734 _ w1765 _]
                      tunnel: w1683 -> [w1686 _ _ _ _ _]
                      tunnel: w1682 -> [_ w1705 _ _ _ _]
                      tunnel: w1681 -> [_ _ _ w1749 _ _]
                      tunnel: w1680 -> [_ _ _ _ _ w1787]
                      frame #0 {
                        # "SN"
                        n1123 = Tick Count (ms)() -> (millisecond timer value=w1685:u32)
                        n1124 = local write "ms timer 3"(w1685) -> ()
                        n1125 = local write "*Board ID1"(w1686) -> ()
                        n1126 = local read "Graph timer 1"() -> (w1688:u32)
                        n1127 = Tick Count (ms)() -> (millisecond timer value=w1689:u32)
                        n1128 = flat-sequence {
                          tunnel: w1689 -> [w1694]
                          tunnel: w1688 -> [w1691]
                          tunnel: [w1690] -> w1687
                          frame #0 {
                            n1129 = Subtract(x=w1694, y=w1691) -> (x-y=w1692:u32)
                            n1130 = local write "Graph timer 1"(w1694) -> ()
                            n1131 = Multiply(x=w1692, y=0.001 ("dt")) -> (x*y=w1690:dbl)
                          }
                        }
                      }
                      frame #1 {
                        # "CDC Data"
                        n1132 = local read "Offset Souce"() -> (w1698:enum32{"Normal", "Raw"})
                        n1133 = Unbundle By Name(w1705) -> ("Left Wing-A, C1/C0"=w1704:dbl, "Left Wing-B, C2/C0"=w1703:dbl, "Left Wing-C, C3/C0"=w1702:dbl, "Right Wing-A, C4/C0"=w1701:dbl, "Right Wing-B, C5/C0"=w1700:dbl, "Right Wing-C, C6/C0"=w1699:dbl)
                        n1134 = Equal?(x=w1698, y=enum32{"Normal", "Raw"}."Normal" ("Offset Souce")) -> (x = y?=w1696:bool)
                        n1135 = case shown="참" w1696 {
                          tunnel: [_ w1720] -> w1695
                          frame False {
                          }
                          frame True {
                            n1136 = local read "CDC Offet"() -> (w1720:T10)
                          }
                        }
                        n1137 = Unbundle By Name(w1695) -> ("Left Wing-A, C1/C0"=w1719:dbl, "Left Wing-B, C2/C0"=w1718:dbl, "Left Wing-C, C3/C0"=w1717:dbl, "Right Wing-A, C4/C0"=w1716:dbl, "Right Wing-B, C5/C0"=w1715:dbl, "Right Wing-C, C6/C0"=w1714:dbl)
                        n1138 = Subtract(x=w1704, y=w1719) -> (x-y=w1711:dbl)
                        n1139 = Subtract(x=w1703, y=w1718) -> (x-y=w1710:dbl)
                        n1140 = Subtract(x=w1702, y=w1717) -> (x-y=w1709:dbl)
                        n1141 = Subtract(x=w1701, y=w1716) -> (x-y=w1708:dbl)
                        n1142 = Subtract(x=w1700, y=w1715) -> (x-y=w1707:dbl)
                        n1143 = Subtract(x=w1699, y=w1714) -> (x-y=w1706:dbl)
                        n1144 = local read "CDC data"() -> (w1713:T10)
                        n1145 = Bundle By Name(cluster=w1713, "Left Wing-A, C1/C0"=w1711, "Left Wing-B, C2/C0"=w1710, "Left Wing-C, C3/C0"=w1709, "Right Wing-A, C4/C0"=w1708, "Right Wing-B, C5/C0"=w1707, "Right Wing-C, C6/C0"=w1706) -> (w1712:T10)
                        n1146 = local write "CDC data"(w1712) -> ()
                      }
                      frame #2 {
                        # "* Plot"
                        n1147 = local read "CDC data"() -> (w1733:T10)
                        n1148 = Unbundle By Name(w1733) -> ("Left Wing-A, C1/C0"=w1732:dbl, "Left Wing-B, C2/C0"=w1725:dbl, "Left Wing-C, C3/C0"=w1724:dbl, "Right Wing-A, C4/C0"=w1723:dbl, "Right Wing-B, C5/C0"=w1722:dbl, "Right Wing-C, C6/C0"=w1721:dbl)
                        n1149 = Build Array(w1732) -> (w1731:dbl[])
                        n1150 = Get Date/Time In Seconds() -> (seconds since 1Jan1904=w1737:timestamp)
                        n1151 = Build Array(w1725) -> (w1730:dbl[])
                        n1152 = Build Array(w1724) -> (w1729:dbl[])
                        n1153 = Build Array(w1722) -> (w1727:dbl[])
                        n1154 = Build Array(w1723) -> (w1728:dbl[])
                        n1155 = Build Array(w1721) -> (w1726:dbl[])
                        n1156 = Bundle By Name("t0"=w1737, "Y"=w1731, "dt"=w1734) -> (w1742:waveform(dbl))  [unwired: 1 in]
                        n1157 = Bundle By Name("t0"=w1737, "Y"=w1730, "dt"=w1734) -> (w1741:waveform(dbl))  [unwired: 1 in]
                        n1158 = Bundle By Name("t0"=w1737, "Y"=w1729, "dt"=w1734) -> (w1740:waveform(dbl))  [unwired: 1 in]
                        n1159 = Bundle By Name("t0"=w1737, "Y"=w1728, "dt"=w1734) -> (w1738:waveform(dbl))  [unwired: 1 in]
                        n1160 = Bundle By Name("t0"=w1737, "Y"=w1727, "dt"=w1734) -> (w1736:waveform(dbl))  [unwired: 1 in]
                        n1161 = Bundle By Name("t0"=w1737, "Y"=w1726, "dt"=w1734) -> (w1735:waveform(dbl))  [unwired: 1 in]
                        n1162 = Build Array(w1742, w1741, w1740, w1738, w1736, w1735) -> (→"CDC(PCAP02) Graph":waveform(dbl)[])
                      }
                      frame #3 {
                        # "IMU Data"
                        n1163 = local read "IMU Offet"() -> (w1764:T11)
                        n1164 = Unbundle By Name(w1749) -> ("Gyroscope X"=w1748:dbl, "Gyroscope Y"=w1747:dbl, "Gyroscope Z"=w1746:dbl, "Accelerometer X"=w1745:dbl, "Accelerometer Y"=w1744:dbl, "Accelerometer Z"=w1743:dbl)
                        n1165 = Unbundle By Name(w1764) -> ("Gyroscope X"=w1761:dbl, "Gyroscope Y"=w1760:dbl, "Gyroscope Z"=w1759:dbl, "Accelerometer X"=w1758:dbl, "Accelerometer Y"=w1757:dbl, "Accelerometer Z"=w1756:dbl)
                        n1166 = Subtract(x=w1748, y=w1761) -> (x-y=w1755:dbl)
                        n1167 = Subtract(x=w1747, y=w1760) -> (x-y=w1754:dbl)
                        n1168 = Subtract(x=w1746, y=w1759) -> (x-y=w1753:dbl)
                        n1169 = Subtract(x=w1745, y=w1758) -> (x-y=w1752:dbl)
                        n1170 = Subtract(x=w1744, y=w1757) -> (x-y=w1751:dbl)
                        n1171 = Subtract(x=w1743, y=w1756) -> (x-y=w1750:dbl)
                        n1172 = local read "IMU data"() -> (w1763:T11)
                        n1173 = Bundle By Name(cluster=w1763, "Gyroscope X"=w1755, "Gyroscope Y"=w1754, "Gyroscope Z"=w1753, "Accelerometer X"=w1752, "Accelerometer Y"=w1751, "Accelerometer Z"=w1750) -> (w1762:T11)
                        n1174 = local write "IMU data"(w1762) -> ()
                      }
                      frame #4 {
                        # "* Plot"
                        n1175 = local read "IMU data"() -> (w1778:T11)
                        n1176 = Unbundle By Name(w1778) -> ("Gyroscope X"=w1777:dbl, "Gyroscope Y"=w1770:dbl, "Gyroscope Z"=w1769:dbl, "Accelerometer X"=w1768:dbl, "Accelerometer Y"=w1767:dbl, "Accelerometer Z"=w1766:dbl)
                        n1177 = Build Array(w1777) -> (w1776:dbl[])
                        n1178 = Get Date/Time In Seconds() -> (seconds since 1Jan1904=w1781:timestamp)
                        n1179 = Build Array(w1770) -> (w1775:dbl[])
                        n1180 = Build Array(w1769) -> (w1774:dbl[])
                        n1181 = Build Array(w1767) -> (w1772:dbl[])
                        n1182 = Build Array(w1768) -> (w1773:dbl[])
                        n1183 = Build Array(w1766) -> (w1771:dbl[])
                        n1184 = Bundle By Name("t0"=w1781, "Y"=w1776, "dt"=w1765) -> (w1785:waveform(dbl))  [unwired: 1 in]
                        n1185 = Bundle By Name("t0"=w1781, "Y"=w1775, "dt"=w1765) -> (w1784:waveform(dbl))  [unwired: 1 in]
                        n1186 = Bundle By Name("t0"=w1781, "Y"=w1774, "dt"=w1765) -> (w1783:waveform(dbl))  [unwired: 1 in]
                        n1187 = Bundle By Name("t0"=w1781, "Y"=w1773, "dt"=w1765) -> (w1782:waveform(dbl))  [unwired: 1 in]
                        n1188 = Bundle By Name("t0"=w1781, "Y"=w1772, "dt"=w1765) -> (w1780:waveform(dbl))  [unwired: 1 in]
                        n1189 = Bundle By Name("t0"=w1781, "Y"=w1771, "dt"=w1765) -> (w1779:waveform(dbl))  [unwired: 1 in]
                        n1190 = Build Array(w1785, w1784, w1783, w1782, w1780, w1779) -> (→"IMU Graph":waveform(dbl)[])
                      }
                      frame #5 {
                        # "BAT raw data"
                        n1191 = local write "Bat(raw)"(w1787) -> ()
                      }
                    }
                  }
                }
              }
            }
          }
          frame #3 {
            # "Debugging data"
            n1192 = local read "Rx-debug"() -> (w1788:bool)
            n1193 = case shown="참" w1788 {
              frame False {
              }
              frame True {
                # "#Processing Received Data"
                n1194 = local read "ms timer 3"() -> (w1793:u32)
                n1195 = local read "Update(ms)"() -> (w1789:u16)
                n1196 = Tick Count (ms)() -> (millisecond timer value=w1792:u32)
                n1197 = Subtract(x=w1792, y=w1793) -> (x-y=w1790:u32)
                n1198 = Greater Or Equal?(x=w1790, y=w1789) -> (x >= y?=w1791:bool)
                n1199 = case shown="참" w1791 {
                  frame False {
                  }
                  frame True {
                    n1200 = local read "BLE Packet (mon)"() -> (w1796:u8[])
                    n1201 = call "SUB-BLE Rx data (Debug)-CDC.vi"("data in"=w1796) -> ("CDC debug"=w1794:T10, "CDC mon"=w1795:T10)  [unwired: 6 in]
                    n1202 = stacked-sequence {
                      seq-local: [w1798 _ _ _ _] -> [_ _ _ w1873 w1892]
                      seq-local: [_ _ _ w1859 _] -> [_ _ _ _ w1881]
                      seq-local: [_ _ _ w1858 _] -> [_ _ _ _ w1901]
                      seq-local: [_ _ w1832 _ _] -> [_ _ _ _ w1880]
                      tunnel: w1795 -> [_ w1810 _ _ _]
                      tunnel: w1794 -> [_ _ w1833 _ _]
                      frame #0 {
                        n1203 = Tick Count (ms)() -> (millisecond timer value=w1797:u32)
                        n1204 = local write "ms timer 3"(w1797) -> ()
                        n1205 = local read "Graph timer 1"() -> (w1799:u32)
                        n1206 = Tick Count (ms)() -> (millisecond timer value=w1800:u32)
                        n1207 = flat-sequence {
                          tunnel: w1800 -> [w1805]
                          tunnel: w1799 -> [w1802]
                          tunnel: [w1801] -> w1798
                          frame #0 {
                            n1208 = Subtract(x=w1805, y=w1802) -> (x-y=w1803:u32)
                            n1209 = local write "Graph timer 1"(w1805) -> ()
                            n1210 = Multiply(x=w1803, y=0.001 ("dt")) -> (x*y=w1801:dbl)
                          }
                        }
                      }
                      frame #1 {
                        # "CDC Data"
                        n1211 = local read "Offset Souce"() -> (w1809:enum32{"Normal", "Raw"})
                        n1212 = Unbundle By Name(w1810) -> ("Left Wing-A, C1/C0"=w1816:dbl, "Left Wing-B, C2/C0"=w1815:dbl, "Left Wing-C, C3/C0"=w1814:dbl, "Right Wing-A, C4/C0"=w1813:dbl, "Right Wing-B, C5/C0"=w1812:dbl, "Right Wing-C, C6/C0"=w1811:dbl)
                        n1213 = Equal?(x=w1809, y=enum32{"Normal", "Raw"}."Normal" ("Offset Souce")) -> (x = y?=w1807:bool)
                        n1214 = case shown="참" w1807 {
                          tunnel: [_ w1831] -> w1806
                          frame False {
                          }
                          frame True {
                            n1215 = local read "CDC Offet"() -> (w1831:T10)
                          }
                        }
                        n1216 = Unbundle By Name(w1806) -> ("Left Wing-A, C1/C0"=w1830:dbl, "Left Wing-B, C2/C0"=w1829:dbl, "Left Wing-C, C3/C0"=w1828:dbl, "Right Wing-A, C4/C0"=w1827:dbl, "Right Wing-B, C5/C0"=w1826:dbl, "Right Wing-C, C6/C0"=w1825:dbl)
                        n1217 = Subtract(x=w1816, y=w1830) -> (x-y=w1822:dbl)
                        n1218 = Subtract(x=w1815, y=w1829) -> (x-y=w1821:dbl)
                        n1219 = Subtract(x=w1814, y=w1828) -> (x-y=w1820:dbl)
                        n1220 = Subtract(x=w1813, y=w1827) -> (x-y=w1819:dbl)
                        n1221 = Subtract(x=w1812, y=w1826) -> (x-y=w1818:dbl)
                        n1222 = Subtract(x=w1811, y=w1825) -> (x-y=w1817:dbl)
                        n1223 = local read "CDC data"() -> (w1824:T10)
                        n1224 = Bundle By Name(cluster=w1824, "Left Wing-A, C1/C0"=w1822, "Left Wing-B, C2/C0"=w1821, "Left Wing-C, C3/C0"=w1820, "Right Wing-A, C4/C0"=w1819, "Right Wing-B, C5/C0"=w1818, "Right Wing-C, C6/C0"=w1817) -> (w1823:T10)
                        n1225 = local write "CDC data"(w1823) -> ()
                      }
                      frame #2 {
                        n1226 = local read "Offset Souce"() -> (w1837:enum32{"Normal", "Raw"})
                        n1227 = Unbundle By Name(w1833) -> ("Left Wing-A, C1/C0"=w1843:dbl, "Left Wing-B, C2/C0"=w1842:dbl, "Left Wing-C, C3/C0"=w1841:dbl, "Right Wing-A, C4/C0"=w1840:dbl, "Right Wing-B, C5/C0"=w1839:dbl, "Right Wing-C, C6/C0"=w1838:dbl)
                        n1228 = Equal?(x=w1837, y=enum32{"Normal", "Raw"}."Raw" ("Offset Souce")) -> (x = y?=w1835:bool)
                        n1229 = case shown="참" w1835 {
                          tunnel: [_ w1857] -> w1834
                          frame False {
                          }
                          frame True {
                            n1230 = local read "CDC Offet"() -> (w1857:T10)
                          }
                        }
                        n1231 = Unbundle By Name(w1834) -> ("Left Wing-A, C1/C0"=w1856:dbl, "Left Wing-B, C2/C0"=w1855:dbl, "Left Wing-C, C3/C0"=w1854:dbl, "Right Wing-A, C4/C0"=w1853:dbl, "Right Wing-B, C5/C0"=w1852:dbl, "Right Wing-C, C6/C0"=w1851:dbl)
                        n1232 = Subtract(x=w1843, y=w1856) -> (x-y=w1849:dbl)
                        n1233 = Subtract(x=w1842, y=w1855) -> (x-y=w1848:dbl)
                        n1234 = Subtract(x=w1841, y=w1854) -> (x-y=w1847:dbl)
                        n1235 = Subtract(x=w1840, y=w1853) -> (x-y=w1846:dbl)
                        n1236 = Subtract(x=w1839, y=w1852) -> (x-y=w1845:dbl)
                        n1237 = Subtract(x=w1838, y=w1851) -> (x-y=w1844:dbl)
                        n1238 = local read "CDC data"() -> (w1850:T10)
                        n1239 = Bundle By Name(cluster=w1850, "Left Wing-A, C1/C0"=w1849, "Left Wing-B, C2/C0"=w1848, "Left Wing-C, C3/C0"=w1847, "Right Wing-A, C4/C0"=w1846, "Right Wing-B, C5/C0"=w1845, "Right Wing-C, C6/C0"=w1844) -> (w1832:T10)
                      }
                      frame #3 {
                        # "* Plot"
                        n1240 = local read "CDC data"() -> (w1872:T10)
                        n1241 = Unbundle By Name(w1872) -> ("Left Wing-A, C1/C0"=w1871:dbl, "Left Wing-B, C2/C0"=w1864:dbl, "Left Wing-C, C3/C0"=w1863:dbl, "Right Wing-A, C4/C0"=w1862:dbl, "Right Wing-B, C5/C0"=w1861:dbl, "Right Wing-C, C6/C0"=w1860:dbl)
                        n1242 = Build Array(w1871) -> (w1870:dbl[])
                        n1243 = Get Date/Time In Seconds() -> (seconds since 1Jan1904=w1859:timestamp)
                        n1244 = Build Array(w1864) -> (w1869:dbl[])
                        n1245 = Build Array(w1863) -> (w1868:dbl[])
                        n1246 = Build Array(w1861) -> (w1866:dbl[])
                        n1247 = Build Array(w1862) -> (w1867:dbl[])
                        n1248 = Build Array(w1860) -> (w1865:dbl[])
                        n1249 = Bundle By Name("t0"=w1859, "Y"=w1870, "dt"=w1873) -> (w1879:waveform(dbl))  [unwired: 1 in]
                        n1250 = Bundle By Name("t0"=w1859, "Y"=w1869, "dt"=w1873) -> (w1878:waveform(dbl))  [unwired: 1 in]
                        n1251 = Bundle By Name("t0"=w1859, "Y"=w1868, "dt"=w1873) -> (w1877:waveform(dbl))  [unwired: 1 in]
                        n1252 = Bundle By Name("t0"=w1859, "Y"=w1867, "dt"=w1873) -> (w1876:waveform(dbl))  [unwired: 1 in]
                        n1253 = Bundle By Name("t0"=w1859, "Y"=w1866, "dt"=w1873) -> (w1875:waveform(dbl))  [unwired: 1 in]
                        n1254 = Bundle By Name("t0"=w1859, "Y"=w1865, "dt"=w1873) -> (w1874:waveform(dbl))  [unwired: 1 in]
                        n1255 = Build Array(w1879, w1878, w1877, w1876, w1875, w1874) -> (w1858:waveform(dbl)[])
                      }
                      frame #4 {
                        n1256 = Unbundle By Name(w1880) -> ("Left Wing-A, C1/C0"=w1899:dbl, "Left Wing-B, C2/C0"=w1898:dbl, "Left Wing-C, C3/C0"=w1885:dbl, "Right Wing-A, C4/C0"=w1884:dbl, "Right Wing-B, C5/C0"=w1883:dbl, "Right Wing-C, C6/C0"=w1882:dbl)
                        n1257 = Build Array(w1899) -> (w1900:dbl[])
                        n1258 = Build Array(w1884) -> (w1890:dbl[])
                        n1259 = Build Array(w1898) -> (w1897:dbl[])
                        n1260 = Build Array(w1885) -> (w1896:dbl[])
                        n1261 = Build Array(w1883) -> (w1893:dbl[])
                        n1262 = Build Array(w1882) -> (w1894:dbl[])
                        n1263 = Bundle By Name("t0"=w1881, "Y"=w1900, "dt"=w1892) -> (w1902:waveform(dbl))  [unwired: 1 in]
                        n1264 = Bundle By Name("t0"=w1881, "Y"=w1897, "dt"=w1892) -> (w1895:waveform(dbl))  [unwired: 1 in]
                        n1265 = Bundle By Name("t0"=w1881, "Y"=w1896, "dt"=w1892) -> (w1891:waveform(dbl))  [unwired: 1 in]
                        n1266 = Bundle By Name("t0"=w1881, "Y"=w1890, "dt"=w1892) -> (w1889:waveform(dbl))  [unwired: 1 in]
                        n1267 = Bundle By Name("t0"=w1881, "Y"=w1893, "dt"=w1892) -> (w1888:waveform(dbl))  [unwired: 1 in]
                        n1268 = Bundle By Name("t0"=w1881, "Y"=w1894, "dt"=w1892) -> (w1887:waveform(dbl))  [unwired: 1 in]
                        n1269 = Build Array (concatenate)(w1901, w1902, w1895, w1891, w1889, w1888, w1887) -> (w1886:waveform(dbl)[])
                        n1270 = local write "CDC(PCAP02) Graph"(w1886) -> ()
                      }
                    }
                  }
                }
              }
            }
          }
          frame #4 {
            # "Force Test"
            n1271 = local read "Comm con status 1"() -> (w1904:bool)
            n1272 = local read "FTS start"() -> (w1903:bool)
            n1273 = case shown="참" w1904 {
              tunnel: w1903 -> [_ w1908]
              frame False {
                n1274 = local write "FTS Testing"(FALSE ("FTS 시험 진행")) -> ()
                n1275 = local write "Test Start"(FALSE ("Test Start")) -> ()
                n1276 = local write "FTS comm."(FALSE ("FTS 수신 정상")) -> ()
              }
              frame True {
                n1277 = case shown="참" w1908 {
                  frame False {
                  }
                  frame True {
                    n1278 = stacked-sequence {
                      frame #0 {
                        # "Init"
                        n1279 = disable-structure shown="비활성화" {
                          frame Disabled {
                            # "170125"
                            # "Test Mode"
                            # "Calibration Mode"
                            # "가로"
                            # "세로"
                            n1280 = local read "Cal/Test select"() -> (w1923:bool)
                            n1281 = Select(t=7, s=w1923, f=5) -> (s? t:f=w1920:i32)
                            n1282 = for {
                              N: 9 -> [_]
                              tunnel: [w1927] -> w1924 mode=indexing
                              tunnel: w1920 -> [w1926]
                              # "가로"
                              n1283 = for {
                                N: w1926 -> [_]
                                tunnel: ["-"] -> w1927 mode=indexing
                              }
                            }
                            n1284 = local write "Test Data table"(w1924) -> ()
                          }
                          frame Enabled {
                          }
                        }
                        n1285 = flat-sequence {
                          frame #0 {
                          }
                          frame #1 {
                            n1286 = Wait Until Next ms Multiple(millisecond multiple=u32 100 ("ms 배수")) -> ()  [unwired: 1 out]
                            n1287 = local write "Mark10 Gauge (lb)"(0.0 ("Mark10 Gauge")) -> ()
                            n1288 = local write "FTS Testing"(TRUE ("FTS 시험 진행")) -> ()
                            n1289 = local write "FTS comm."(FALSE ("FTS 수신 정상")) -> ()
                            n1290 = local write "status string"("Force Test Mode..." ("status string")) -> ()
                            n1291 = local write "FTS OP status"(T8 "Test_Start" ("FTS OP status")) -> ()
                            n1292 = Format Date/Time String(time format string (%c)="%Y/%m/%d %H:%M:%S> Force Test Start\n" ("상태")) -> (date/time string=w1913:string)  [unwired: 2 in]
                            n1293 = local write "Test Status"(w1913) -> ()
                            n1294 = call "Sub-CDC_Data_Cluster_Buffer.vi"("Mode"=enum16{"Init", "Add", "Add Load", "Out"}."Init") -> ()  [unwired: 10 in, 1 out]
                            n1295 = local write "Load Graph"(cluster{dbl[], dbl[]} {[], []} ("Load Graph")) -> ()
                            n1296 = local write "FTS table index"(0 ("FTS table index")) -> ()
                          }
                        }
                      }
                      frame #1 {
                        # "the number of Load Test Profile"
                        # "col"
                        # "Calibration Profile Load"
                        # "170125"
                        # "#FTS_PROFILE"
                        n1297 = disable-structure shown="활성화" {
                          disable-tunnel: [w1959 w1966] -> w1943
                          frame Enabled {
                            n1298 = call <vilib>:"Application Directory.vi"() -> ("Application Directory"=w1958:path)
                            n1299 = Build Path(base path=w1958, name or relative path="Template" ("이름 또는 상대 경로")) -> (appended path=w1961:path)
                            n1300 = Build Path(base path=w1961, name or relative path="FTS Profile-OS.csv" ("이름 또는 상대 경로")) -> (appended path=w1959:path)
                          }
                          frame Disabled {
                            # "For Validation Test"
                            n1301 = call <vilib>:"Application Directory.vi"() -> ("Application Directory"=w1964:path)
                            n1302 = Build Path(base path=w1964, name or relative path="Template" ("이름 또는 상대 경로")) -> (appended path=w1963:path)
                            n1303 = call "파일 대화 상자"("start path"=w1963) -> ("selected path"=w1966:path)  [unwired: 11 in, 3 out]
                          }
                        }
                        n1304 = call "Load_Array_Data_to_File_txt.vi"("file path (use dialog)"=w1943) -> ("array"=w1936:string[][])  [unwired: 8 in, 2 out]
                        n1305 = Index Array(array=w1936, index (col)=0 ("비활성화된 인덱스 (열)")) -> (element=w1941:string[])  [unwired: 1 in]
                        n1306 = local write "Test profile"(w1936) -> ()
                        n1307 = for {
                          tunnel: w1941 -> [w1968] mode=indexing
                          tunnel: [w1968] -> w1933 mode=indexing if=w1967
                          n1308 = String Subset(string=w1968, length (rest)=4 ("길이(나머지)")) -> (substring=w1971:string)  [unwired: 1 in]
                          n1309 = To Upper Case(1:w1971) -> (0:w1970:string)
                          n1310 = Equal?(x=w1970, y="LOAD") -> (x = y?=w1967:bool)
                        }
                        n1311 = Index Array(array=w1936, index (col)=6 ("비활성화된 인덱스 (열)")) -> (element=w1935:string[])  [unwired: 1 in]
                        n1312 = for {
                          tunnel: w1935 -> [w1954] mode=indexing
                          tunnel: [w1951] -> w1934 mode=indexing if=w1951
                          n1313 = Decimal String To Number(string=w1954) -> (number=w1953:i32)  [unwired: 2 in, 1 out]
                          n1314 = Equal?(x=1, y=w1953) -> (x = y?=w1951:bool)
                        }
                        n1315 = Array Size(array=w1933) -> (size(s)=w1932:i32)
                        n1316 = Array Size(array=w1934) -> (size(s)=w1931:i32)
                        n1317 = Subtract(x=w1932, y=w1931) -> (x-y=w1930:i32)
                        n1318 = disable-structure shown="활성화" {
                          disable-tunnel: w1933 -> [w1947 w1950]
                          disable-tunnel: w1930 -> [w1946 _]
                          disable-tunnel: [w1944 w1950] -> w1929
                          frame Disabled {
                            n1319 = Insert Into Array(array=w1947, index=w1946, new element="Offset") -> (w1945:string[])
                            n1320 = Build Array (concatenate)("Offset", w1945) -> (w1944:string[])
                          }
                          frame Enabled {
                          }
                        }
                        n1321 = Array Size(array=w1929) -> (size(s)=w1938:i32)
                        n1322 = for {
                          N: 9 -> [_]
                          tunnel: [w1956] -> w1939 mode=indexing
                          tunnel: w1938 -> [w1955]
                          # "row"
                          n1323 = for {
                            N: w1955 -> [_]
                            tunnel: ["-"] -> w1956 mode=indexing
                          }
                        }
                        n1324 = local write "Test Data table"(w1939) -> ()
                        n1325 = property on="Test Data table" class="Tbl (엄격한)"("Column Headers[]"=w1929) -> ()  [unwired: 2 in, 2 out]
                      }
                      frame #2 {
                        n1326 = local read "Port-FTS"() -> (w1978:refnum<visa-resource-name>)
                        n1327 = control-ref of="Test Status"() -> (w1974:refnum<vi>)
                        n1328 = call "_Serial_Mark10-Connection_Check.vi"("Serial Port"=w1978) -> ("Normal reception"=w1977:bool, "VISA resource name out"=w1976:refnum<visa-resource-name>)  [unwired: 3 in]
                        n1329 = call "SUB-Status string update.vi"("String In"="Check Serial port of Mark-10\n" ("Force Test Status"), "Add Date"=TRUE ("날짜추가"), "reference"=w1974) -> ()  [unwired: 2 in, 1 out]
                        n1330 = case shown="거짓" w1977 {
                          tunnel: w1976 -> [_ _]
                          frame False {
                            # "Communication fail"
                            n1331 = local write "FTS OP status"(T8 "Test_End" ("FTS OP status")) -> ()
                            n1332 = One Button Dialog(message="Cannot find MARK10.\nCheck comm port." ("메시지")) -> ()  [unwired: 1 in, 1 out]
                          }
                          frame True {
                            n1333 = local read "Port-FTS"() -> (w1981:refnum<visa-resource-name>)
                            n1334 = call "_Serial_Mark10-Setup(Zero).vi"("Serial Port"=w1981) -> ()  [unwired: 4 in, 1 out]
                          }
                        }
                        n1335 = local write "FTS comm."(w1977) -> ()
                      }
                      frame #3 {
                        n1336 = while {
                          stop <- w1984 stop-if-true
                          n1337 = local read "Test profile"() -> (w1983:string[][])
                          n1338 = case shown="\"Gen_Report\"" "FTS OP status" {
                            tunnel: [w1989 _ _ _ TRUE _] -> w1984
                            tunnel: w1983 -> [_ _ w1994 w2179 _ _]
                            frame "Test_Start" {
                              n1339 = control-ref of="Test Status"() -> (w1987:refnum<vi>)
                              n1340 = local write "FTS OP status"(T8 "Check_Before_Test" ("FTS OP status")) -> ()
                              n1341 = call "SUB-Status string update.vi"("String In"="Force Test Start!\n" ("Force Test Status"), "Add Date"=TRUE ("날짜추가"), "reference"=w1987) -> ()  [unwired: 2 in, 1 out]
                              n1342 = local read "stop"() -> (w1989:bool)
                            }
                            frame "Check_Before_Test" {
                              n1343 = local read "Port-FTS"() -> (w1992:refnum<visa-resource-name>)
                              n1344 = call "_Serial_Mark10-Data reception(Gauge).vi"("Serial Port"=w1992) -> ("data(lb)"=w1991:dbl, "Normal reception"=w1993:bool)  [unwired: 2 in, 1 out]
                              n1345 = local write "Mark10 Gauge (lb)"(w1991) -> ()
                              n1346 = local write "FTS comm."(w1993) -> ()
                              n1347 = local write "FTS OP status"(T8 "Proceed-Press" ("FTS OP status")) -> ()
                            }
                            frame "Proceed-Press" {
                              n1348 = stacked-sequence {
                                tunnel: w1994 -> [_ w1999 _]
                                frame #0 {
                                n1349 = control-ref of="Test Status"() -> (w1997:refnum<vi>)
                                n1350 = local write "CDC Offet"(T10 {"Left Wing-A, C1/C0"=0.0, "Left Wing-B, C2/C0"=0.0, "Left Wing-C, C3/C0"=0.0, "Right Wing-A, C4/C0"=0.0, "Right Wing-B, C5/C0"=0.0, "Right Wing-C, C6/C0"=0.0} ("CDC Offet")) -> ()
                                n1351 = call "SUB-Status string update.vi"("String In"="Start Force test by Profile" ("Force Test Status"), "Add Date"=TRUE ("날짜추가"), "reference"=w1997) -> ()  [unwired: 2 in, 1 out]
                                }
                                frame #1 {
                                n1352 = for {
                                tunnel: w1999 -> [w2002] mode=indexing
                                i -> [w2000]
                                stop <- w2001 continue-if-true
                                n1353 = stacked-sequence {
                                seq-local: [_ w2017 _ _ _ _ _ _ _] -> [_ _ _ _ w2039 w2080 _ _ _]
                                seq-local: [w2003 _ _ _ _ _ _ _ _] -> [_ _ _ _ w2038 w2066 _ _ _]
                                seq-local: [_ _ w2024 _ _ _ _ _ _] -> [_ _ _ _ _ _ _ w2135 _]
                                tunnel: w2000 -> [w2010 _ _ _ _ _ _ w2134 _]
                                tunnel: w2002 -> [w2004 w2022 w2027 _ _ _ w2103 _ w2163]
                                tunnel: [_ w2019 _ _ _ _ _ _ _] -> w2001
                                frame #0 {
                                # "Data Aquisition?"
                                # "String for test state"
                                n1354 = Index Array(array=w2004, index=4 ("인덱스")) -> (element=w2006:string)
                                n1355 = Fract/Exp String To Number(string=w2006) -> (number=w2005:dbl)  [unwired: 3 in, 1 out]
                                n1356 = Not Equal To 0?(x=w2005) -> (x != 0?=w2003:bool)
                                n1357 = Index Array(array=w2004, index=0 ("인덱스")) -> (element=w2008:string)
                                n1358 = Increment(x=w2010) -> (x+1=w2011:i32)
                                n1359 = control-ref of="Test Status"() -> (w2014:refnum<vi>)
                                n1360 = Format Into String(format string="Force Testing-Profile(%d)...%s" ("Force Test Status"), w2011, w2008) -> (resulting string=w2013:string)  [unwired: 2 in, 1 out]
                                n1361 = call "SUB-Status string update.vi"("String In"=w2013, "Add Date"=TRUE ("날짜추가"), "reference"=w2014) -> ()  [unwired: 2 in, 1 out]
                                }
                                frame #1 {
                                # "Press"
                                n1362 = Index Array(array=w2022, index=1 ("인덱스")) -> (element=w2020:string)
                                n1363 = local read "Port-FTS"() -> (w2023:refnum<visa-resource-name>)
                                n1364 = Fract/Exp String To Number(string=w2020) -> (number=w2017:dbl)  [unwired: 3 in, 1 out]
                                n1365 = call "_Serial_Mark10-Control (Press Config).vi"("FTS Operation state"=T27 "Start pressure control", "Press Setting(lb)"=w2017, "Serial Port"=w2023) -> ("Gauge Pressure(lb)"=w2018:dbl, "Communication is normal"=w2019:bool)  [unwired: 1 out]
                                n1366 = local write "Mark10 Gauge (lb)"(w2018) -> ()
                                n1367 = local write "FTS comm."(w2019) -> ()
                                }
                                frame #2 {
                                # "Delay"
                                n1368 = Tick Count (ms)() -> (millisecond timer value=w2026:u32)
                                n1369 = Index Array(array=w2027, index=2 ("인덱스")) -> (element=w2028:string)
                                n1370 = Fract/Exp String To Number(string=w2028) -> (number=w2025:dbl)  [unwired: 3 in, 1 out]
                                n1371 = while {
                                tunnel: w2026 -> [w2036]
                                tunnel: w2025 -> [w2034]
                                tunnel: [w2030] -> w2024
                                stop <- w2033 stop-if-true
                                n1372 = Tick Count (ms)() -> (millisecond timer value=w2037:u32)
                                n1373 = Subtract(x=w2037, y=w2036) -> (x-y=w2035:u32)
                                n1374 = local read "Port-FTS"() -> (w2031:refnum<visa-resource-name>)
                                n1375 = Greater Or Equal?(x=w2035, y=w2034) -> (x >= y?=w2033:bool)
                                n1376 = call "_Serial_Mark10-Data reception(Gauge).vi"("Serial Port"=w2031) -> ("data(lb)"=w2030:dbl)  [unwired: 2 in, 2 out]
                                n1377 = local write "Mark10 Gauge (lb)"(w2030) -> ()
                                n1378 = Wait Until Next ms Multiple(millisecond multiple=u32 50 ("ms 배수")) -> ()  [unwired: 1 out]
                                }
                                }
                                frame #3 {
                                # "Clear BLE Buffer"
                                n1379 = call "SUB-BLE Rx data Clear.vi"() -> ()  [unwired: 6 in]
                                }
                                frame #4 {
                                n1380 = case shown="참" w2038 {
                                tunnel: w2039 -> [_ w2052]
                                frame False {
                                }
                                frame True {
                                # "Rescale to the number of data"
                                # "Data Aquisition Delay & Read Gauge"
                                n1381 = Equal To 0?(x=w2052) -> (x = 0?=w2048:bool)
                                n1382 = Select(t=0.5, s=w2048, f=1.0) -> (s? t:f=w2046:dbl)
                                n1383 = Select(t=50, s=w2048, f=100) -> (s? t:f=w2044:i32)
                                n1384 = Get Date/Time In Seconds() -> (seconds since 1Jan1904=w2051:timestamp)
                                n1385 = while {
                                tunnel: w2051 -> [w2057]
                                tunnel: w2046 -> [w2054]
                                tunnel: [w2053] -> w2043 mode=indexing
                                stop <- w2056 stop-if-true
                                n1386 = Get Date/Time In Seconds() -> (seconds since 1Jan1904=w2058:timestamp)
                                n1387 = Subtract(x=w2058, y=w2057) -> (x-y=w2055:dbl)
                                n1388 = Greater Or Equal?(x=w2055, y=w2054) -> (x >= y?=w2056:bool)
                                n1389 = local read "Port-FTS"() -> (w2059:refnum<visa-resource-name>)
                                n1390 = call "_Serial_Mark10-Data reception(Gauge).vi"("Serial Port"=w2059) -> ("data(lb)"=w2053:dbl)  [unwired: 2 in, 2 out]
                                }
                                n1391 = To Double Precision Float(number=w2044) -> (double precision float=w2042:dbl)
                                n1392 = call "Sub_X_Scale_Change.vi"("Target Scale"=w2042, "input"=w2043) -> ("output"=w2040:dbl[])  [unwired: 9 in]
                                n1393 = call "Sub-CDC_Data_Cluster_Buffer.vi"("Mode"=enum16{"Init", "Add", "Add Load", "Out"}."Add Load", "Input Load"=w2040) -> ()  [unwired: 9 in, 1 out]
                                }
                                }
                                }
                                frame #5 {
                                # "CDC Data acquisition"
                                n1394 = Equal To 0?(x=w2080) -> (x = 0?=w2079:bool)
                                n1395 = Select(t=50, s=w2079, f=100) -> (s? t:f=w2076:i32)
                                n1396 = for {
                                N: w2076 -> [_]
                                tunnel: [w2093] -> w2069 mode=indexing
                                tunnel: [w2092] -> w2070 mode=indexing
                                tunnel: [w2091] -> w2071 mode=indexing
                                tunnel: [w2090] -> w2072 mode=indexing
                                tunnel: [w2089] -> w2073 mode=indexing
                                tunnel: [w2088] -> w2074 mode=indexing
                                tunnel: [w2085] -> w2067 mode=indexing
                                n1397 = local read "CDC data"() -> (w2086:T10)
                                n1398 = call "SUB-BLE Rx data (Mon)-Wait.vi"("Timeout(ms)"=u16 100) -> ("RxReady"=w2094:bool)  [unwired: 4 in]
                                n1399 = case shown="참" w2094 {
                                tunnel: [w2098 w2101] -> w2087
                                tunnel: w2086 -> [w2098 _]
                                tunnel: [u16 0 ("Bat") w2099] -> w2085
                                frame False {
                                }
                                frame True {
                                n1400 = call "SUB-BLE Rx data (Mon)-Classify.vi"() -> ("data out"=w2100:u8[])  [unwired: 5 in, 4 out]
                                n1401 = call "SUB-BLE Rx data (Mon)-CDC IMU.vi"("data in"=w2100) -> ("CDC data"=w2101:T10, "Bat"=w2099:u16)  [unwired: 4 in, 2 out]
                                }
                                }
                                n1402 = Unbundle By Name(w2087) -> ("Left Wing-A, C1/C0"=w2093:dbl, "Left Wing-B, C2/C0"=w2092:dbl, "Left Wing-C, C3/C0"=w2091:dbl, "Right Wing-A, C4/C0"=w2090:dbl, "Right Wing-B, C5/C0"=w2089:dbl, "Right Wing-C, C6/C0"=w2088:dbl)
                                n1403 = Wait Until Next ms Multiple(millisecond multiple=u32 5 ("ms 배수")) -> ()  [unwired: 1 out]
                                }
                                n1404 = call-poly <vilib>:"Mean.vi"("X"=w2069) -> ("mean"=w2065:dbl)  [unwired: 1 out]
                                n1405 = call-poly <vilib>:"Mean.vi"("X"=w2070) -> ("mean"=w2064:dbl)  [unwired: 1 out]
                                n1406 = call-poly <vilib>:"Mean.vi"("X"=w2071) -> ("mean"=w2063:dbl)  [unwired: 1 out]
                                n1407 = call-poly <vilib>:"Mean.vi"("X"=w2072) -> ("mean"=w2062:dbl)  [unwired: 1 out]
                                n1408 = call-poly <vilib>:"Mean.vi"("X"=w2073) -> ("mean"=w2061:dbl)  [unwired: 1 out]
                                n1409 = call-poly <vilib>:"Mean.vi"("X"=w2074) -> ("mean"=w2060:dbl)  [unwired: 1 out]
                                n1410 = Bundle By Name(cluster=T10 {"Left Wing-A, C1/C0"=0.0, "Left Wing-B, C2/C0"=0.0, "Left Wing-C, C3/C0"=0.0, "Right Wing-A, C4/C0"=0.0, "Right Wing-B, C5/C0"=0.0, "Right Wing-C, C6/C0"=0.0} ("CDC data"), "Left Wing-A, C1/C0"=w2065, "Left Wing-B, C2/C0"=w2064, "Left Wing-C, C3/C0"=w2063, "Right Wing-A, C4/C0"=w2062, "Right Wing-B, C5/C0"=w2061, "Right Wing-C, C6/C0"=w2060) -> (w2081:T10)
                                n1411 = Bundle By Name(cluster=T30 {"LWA"=[], "LWB"=[], "LWC"=[], "RWA"=[], "RWB"=[], "RWC"=[], "Bat"=[]} ("Output CL"), "LWA"=w2069, "LWB"=w2070, "LWC"=w2071, "RWA"=w2072, "RWB"=w2073, "RWC"=w2074, "Bat"=w2067) -> (w2075:T30)
                                n1412 = local write "CDC data"(w2081) -> ()
                                n1413 = case shown="참" w2066 {
                                tunnel: w2075 -> [_ w2084]
                                frame False {
                                }
                                frame True {
                                n1414 = call "Sub-CDC_Data_Cluster_Buffer.vi"("Mode"=enum16{"Init", "Add", "Add Load", "Out"}."Add", "Input CL"=w2084) -> ()  [unwired: 9 in, 1 out]
                                }
                                }
                                }
                                frame #6 {
                                n1415 = Index Array(array=w2103, index=4 ("인덱스")) -> (element=w2105:string)
                                n1416 = Fract/Exp String To Number(string=w2105) -> (number=w2104:dbl)  [unwired: 3 in, 1 out]
                                n1417 = Not Equal To 0?(x=w2104) -> (x != 0?=w2102:bool)
                                n1418 = case shown="참" w2102 {
                                frame False {
                                }
                                frame True {
                                w2121 = i16 1 ("정밀도(6)")
                                n1419 = local read "CDC data"() -> (w2132:T10)
                                n1420 = Unbundle By Name(w2132) -> ("Left Wing-A, C1/C0"=w2116:dbl, "Left Wing-B, C2/C0"=w2117:dbl, "Left Wing-C, C3/C0"=w2118:dbl, "Right Wing-A, C4/C0"=w2114:dbl, "Right Wing-B, C5/C0"=w2113:dbl, "Right Wing-C, C6/C0"=w2112:dbl)
                                n1421 = local read "Mark10 Gauge (lb)"() -> (w2111:dbl)
                                n1422 = local read "FTS table index"() -> (w2107:i32)
                                n1423 = Compound Arithmetic op=ADD(w2118, w2117, w2116) -> (w2119:dbl)
                                n1424 = Compound Arithmetic op=ADD(w2114, w2113, w2112) -> (w2115:dbl)
                                n1425 = Number To Fractional String(number=w2116, precision (6)=w2121) -> (F-format string=w2131:string)  [unwired: 2 in]
                                n1426 = Number To Fractional String(number=w2117, precision (6)=w2121) -> (F-format string=w2130:string)  [unwired: 2 in]
                                n1427 = Number To Fractional String(number=w2111, precision (6)=i16 2 ("정밀도(6)")) -> (F-format string=w2109:string)  [unwired: 2 in]
                                n1428 = Number To Fractional String(number=w2118, precision (6)=w2121) -> (F-format string=w2129:string)  [unwired: 2 in]
                                n1429 = Number To Fractional String(number=w2119, precision (6)=w2121) -> (F-format string=w2122:string)  [unwired: 2 in]
                                n1430 = Number To Fractional String(number=w2114, precision (6)=w2121) -> (F-format string=w2128:string)  [unwired: 2 in]
                                n1431 = Number To Fractional String(number=w2113, precision (6)=w2121) -> (F-format string=w2127:string)  [unwired: 2 in]
                                n1432 = Number To Fractional String(number=w2112, precision (6)=w2121) -> (F-format string=w2126:string)  [unwired: 2 in]
                                n1433 = Number To Fractional String(number=w2115, precision (6)=w2121) -> (F-format string=w2120:string)  [unwired: 2 in]
                                n1434 = local read "Test Data table"() -> (w2123:string[][])
                                n1435 = Increment(x=w2107) -> (x+1=w2108:i32)
                                n1436 = Build Array(w2109, w2131, w2130, w2129, w2122, w2128, w2127, w2126, w2120) -> (w2125:string[])
                                n1437 = local write "FTS table index"(w2108) -> ()
                                n1438 = Replace Array Subset(array=w2123, new element=w2125, index (col)=w2107) -> (w2124:string[][])  [unwired: 1 in]
                                n1439 = local write "Test Data table"(w2124) -> ()
                                }
                                }
                                }
                                frame #7 {
                                # "Load Graph"
                                n1440 = local read "Test Data table"() -> (w2136:string[][])
                                n1441 = disable-structure shown="활성화" {
                                disable-tunnel: [w2144 w2154] -> w2133
                                disable-tunnel: w2136 -> [w2143 _]
                                disable-tunnel: w2135 -> [_ w2157]
                                disable-tunnel: w2134 -> [_ w2161]
                                frame Disabled {
                                n1442 = local read "FTS table index"() -> (w2139:i32)
                                n1443 = Decrement(x=w2139) -> (x-1=w2138:i32)
                                n1444 = Array Subset(array=w2143, index (col)=1 ("비활성화된 인덱스 (열)"), length (col)=w2138) -> (w2140:string[][])  [unwired: 2 in]
                                n1445 = Fract/Exp String To Number(string=w2140) -> (number=w2142:dbl[][])  [unwired: 3 in, 1 out]
                                n1446 = for {
                                N: 8 -> [_]
                                tunnel: [w2152] -> w2144 mode=indexing
                                tunnel: w2142 -> [w2151]
                                i -> [w2149]
                                # "Y"
                                # "X"
                                n1447 = Add(x=1, y=w2149) -> (x+y=w2147:i32)
                                n1448 = Index Array(array=w2151, index (row)=0 ("비활성화된 인덱스 (열)")) -> (element=w2146:dbl[])  [unwired: 1 in]
                                n1449 = Index Array(array=w2151, index (row)=w2147) -> (element=w2145:dbl[])  [unwired: 1 in]
                                n1450 = Bundle(w2146, w2145) -> (w2152:cluster{dbl[], dbl[]})  [unwired: 1 in]
                                }
                                }
                                frame Enabled {
                                n1451 = To Double Precision Float(number=w2161) -> (double precision float=w2159:dbl)
                                n1452 = property on="Load Graph" class="XYGraph (엄격한)"() -> ("Value"=w2153:cluster{dbl[], dbl[]})  [unwired: 2 in, 2 out]
                                n1453 = Unbundle(w2153) -> (w2160:dbl[], w2158:dbl[])
                                n1454 = Build Array (concatenate)(w2158, w2157) -> (w2155:dbl[])
                                n1455 = Build Array (concatenate)(w2160, w2159) -> (w2156:dbl[])
                                n1456 = Bundle(w2156, w2155) -> (w2154:cluster{dbl[], dbl[]})  [unwired: 1 in]
                                }
                                }
                                "Load Graph" <- w2133
                                }
                                frame #8 {
                                n1457 = Index Array(array=w2163, index=5 ("인덱스")) -> (element=w2165:string)
                                n1458 = Fract/Exp String To Number(string=w2165) -> (number=w2164:dbl)  [unwired: 3 in, 1 out]
                                n1459 = Not Equal To 0?(x=w2164) -> (x != 0?=w2162:bool)
                                n1460 = case shown="참" w2162 {
                                frame False {
                                }
                                frame True {
                                n1461 = stacked-sequence {
                                seq-local: [w2168 _] -> [_ w2174]
                                frame #0 {
                                n1462 = local read "Port-FTS"() -> (w2168:refnum<visa-resource-name>)
                                n1463 = control-ref of="Test Status"() -> (w2170:refnum<vi>)
                                n1464 = call "_Serial_Mark10-Control (Press Config).vi"("FTS Operation state"=T27 "Move Header Up", "Serial Port"=w2168) -> ("Gauge Pressure(lb)"=w2172:dbl, "Communication is normal"=w2173:bool)  [unwired: 1 in, 1 out]
                                n1465 = call "SUB-Status string update.vi"("String In"="Head Up" ("Force Test Status"), "Add Date"=TRUE ("날짜추가"), "reference"=w2170) -> ()  [unwired: 2 in, 1 out]
                                n1466 = local write "Mark10 Gauge (lb)"(w2172) -> ()
                                n1467 = local write "FTS comm."(w2173) -> ()
                                }
                                frame #1 {
                                n1468 = call "_Serial_Mark10-Setup(Zero).vi"("Serial Port"=w2174) -> ()  [unwired: 4 in, 1 out]
                                }
                                }
                                }
                                }
                                }
                                }
                                }
                                }
                                frame #2 {
                                n1469 = local write "FTS OP status"(T8 "Gen_Report" ("FTS OP status")) -> ()
                                n1470 = control-ref of="Test Status"() -> (w2177:refnum<vi>)
                                n1471 = call "SUB-Status string update.vi"("String In"="Done Force test by Profile\n" ("Force Test Status"), "Add Date"=TRUE ("날짜추가"), "reference"=w2177) -> ()  [unwired: 2 in, 1 out]
                                }
                              }
                            }
                            frame "Check_After_Test" {
                              n1472 = disable-structure shown="활성화" {
                                disable-tunnel: w2179 -> [w2181 _]
                                frame Disabled {
                                # "LAT"
                                # "CAL"
                                # "Test End & \nSave Measurement data"
                                n1473 = stacked-sequence {
                                seq-local: [_ w2207 _] -> [_ _ w2217]
                                seq-local: [w2195 _ _] -> [_ w2206 _]
                                seq-local: [w2189 _ _] -> [_ _ w2216]
                                seq-local: [w2186 _ _] -> [_ _ w2215]
                                seq-local: [w2185 _ _] -> [_ _ w2214]
                                tunnel: w2181 -> [w2188 _ _]
                                frame #0 {
                                w2203 = T33 1 items=["사용자 홈"=0, "사용자 데스크탑"=1, "사용자 문서"=2, "사용자 어플리케이션 데이터"=3, "사용자 환경"=4, "사용자 임시"=5, "퍼블릭 문서"=6, "퍼블릭 어플리케이션 데이터"=7, "퍼블릭 환경"=8, "퍼블릭 캐시"=13, "시스템 코어 라이브러리"=9, "시스템 설치된 라이브러리"=10, "어플리케이션 파일"=11, "부팅 볼륨 루트"=12] ("system directory type")
                                n1474 = local read "Test Data table"() -> (w2187:string[][])
                                n1475 = call "SUB-FTS_Result_divide.vi"("Table Value"=w2187, "Test profile"=w2188) -> ("Load Test data"=w2185:string[][], "Cal data"=w2186:string[][])  [unwired: 8 in]
                                n1476 = call "SUB-module-Current VI Path.vi"() -> ("현재 VI 경로"=w2192:path)
                                n1477 = call <vilib>:"Get System Directory.vi"("system directory type"=w2203) -> ("system directory"=w2202:path)  [unwired: 10 in]
                                n1478 = Path To String(path=w2192) -> (string=w2191:string)
                                n1479 = Path To String(path=w2202) -> (string=w2201:string)
                                n1480 = Concatenate Strings(w2191, "\\Template" ("이름 또는 상대 경로"), "\\GEN4 FTS Test Report rev2.xlsx" ("이름 또는 상대 경로")) -> (w2190:string)
                                n1481 = String To Path(string=w2190) -> (path=w2189:path)
                                n1482 = Concatenate Strings(w2201, "\\GEN4-GUI Test data" ("상태")) -> (w2195:string)
                                n1483 = String To Path(string=w2195) -> (path=w2199:path)
                                n1484 = call <vilib>:"Check if File or Folder Exists.vi"("path"=w2199) -> ("error out"=w2196:errorcluster, "file or folder exists?"=w2198:bool, "dup path"=w2197:path)  [unwired: 8 in]
                                n1485 = case shown="거짓" w2198 {
                                tunnel: w2197 -> [w2205 _]
                                tunnel: w2196 -> [w2204 _]
                                frame False {
                                n1486 = Create Folder(path (use dialog)=w2205, error in=w2204) -> ()  [unwired: 1 in, 3 out]
                                }
                                frame True {
                                }
                                }
                                }
                                frame #1 {
                                # "* Filename(rev)-date (trst name)"
                                # "파일 저장 경로"
                                n1487 = local read "Test name"() -> (w2212:string)
                                n1488 = Format Date/Time String(time format string (%c)="%Y%m%d %H%M%S" ("상태")) -> (date/time string=w2211:string)  [unwired: 2 in]
                                n1489 = Format Into String(format string="\\\\GEN4 FTS (PP3A)-%s (%s).xlsx" ("상태"), w2211, w2212) -> (resulting string=w2208:string)  [unwired: 2 in, 1 out]
                                n1490 = Concatenate Strings(w2206, w2208) -> (w2213:string)
                                n1491 = String To Path(string=w2213) -> (path=w2207:path)
                                }
                                frame #2 {
                                n1492 = call <vilib>:"New Report.vi"("window state (normal)"=T22."normal", "report type"=T21."Excel", "template (empty)"=w2216) -> ("report out"=w2220:refnum<class "NI_report.lvclass">, "error out"=w2221:errorcluster)  [unwired: 11 in]
                                n1493 = stacked-sequence {
                                tunnel: w2220 -> [w2225 w2250 w2252 w2278]
                                tunnel: w2221 -> [w2224 w2249 w2253 w2277]
                                tunnel: [w2225 _ _ _] -> w2223
                                tunnel: [w2224 _ _ _] -> w2222
                                tunnel: w2215 -> [_ _ _ w2276]
                                tunnel: w2214 -> [_ _ _ w2275]
                                frame #0 {
                                }
                                frame #1 {
                                w2228 = 11 ("column")
                                w2235 = 2 ("row")
                                w2242 = 1 items=["top", "center", "bottom"] ("vertical alignment (top)")
                                # "Date"
                                # "박스의 좌측 상단 좌표"
                                n1494 = Add(x=w2228, y=3) -> (x+y=w2226:i32)
                                n1495 = Increment(x=w2235) -> (x+1=w2230:i32)
                                n1496 = Bundle By Name(cluster=cluster{"row":i32, "column":i32} {"row"=3, "column"=10} ("start (-1, -1)"), "row"=w2230, "column"=w2226) -> (w2229:cluster{"row":i32, "column":i32})
                                n1497 = Bundle By Name(cluster=cluster{"row":i32, "column":i32} {"row"=3, "column"=10} ("start (-1, -1)"), "row"=w2230, "column"=w2228) -> (w2236:cluster{"row":i32, "column":i32})
                                n1498 = Format Date/Time String(time format string (%c)="%Y/%m/%d-%H:%M:%S" ("상태")) -> (date/time string=w2248:string)  [unwired: 2 in]
                                n1499 = call <vilib>:"Excel Easy Text.vi"("report in"=w2250, "font"=T23 {"font name"="", "font size"=11.0, "bold"=1, "italic"=0, "underline"=0, "strike through"=0, "font color"=16777216}, "text"=w2248, "start (-1, -1)"=w2236, "end (-1, -1)"=w2229, "error in (no error)"=w2249) -> ("report out"=w2246:refnum<class "NI_report.lvclass">, "next cell bottom-left"=w2244:cluster{"row":i32, "column":i32}, "next cell top-right"=w2243:cluster{"row":i32, "column":i32}, "error out"=w2245:errorcluster)  [unwired: 5 in, 1 out]
                                n1500 = Bundle By Name(cluster=cluster{"row":i32, "column":i32} {"row"=3, "column"=10} ("start (-1, -1)"), "row"=w2235, "column"=w2228) -> (w2234:cluster{"row":i32, "column":i32})
                                n1501 = call <vilib>:"Excel Set Cell Alignment.vi"("report in"=w2246, "vertical alignment (top)"=w2242, "horizontal alignment (left)"=w2242, "start (-1, -1)"=w2244, "end (-1, -1)"=w2243, "error in (no error)"=w2245) -> ("report out"=w2241:refnum<class "NI_report.lvclass">, "error out"=w2240:errorcluster)  [unwired: 8 in]
                                n1502 = call <vilib>:"Excel Set Cell Color and Border.vi"("report in"=w2241, "outside border"=T24 {"on/off"=TRUE, "weight"=2, "color"=0}, "background color (w)"=u32 16777215, "start (-1, -1)"=w2234, "end (-1, -1)"=w2229, "error in (no error)"=w2240) -> ()  [unwired: 8 in, 2 out]
                                }
                                frame #2 {
                                w2256 = 1 ("column")
                                w2263 = 4 ("row")
                                w2270 = 1 items=["top", "center", "bottom"] ("vertical alignment (top)")
                                # "Device No."
                                # "박스의 좌측 상단 좌표"
                                n1503 = local read "Test name"() -> (w2251:string)
                                n1504 = Increment(x=w2256) -> (x+1=w2255:i32)
                                n1505 = Increment(x=w2263) -> (x+1=w2258:i32)
                                n1506 = Increment(x=w2255) -> (x+1=w2257:i32)
                                n1507 = Bundle By Name(cluster=cluster{"row":i32, "column":i32} {"row"=3, "column"=10} ("start (-1, -1)"), "row"=w2258, "column"=w2257) -> (w2254:cluster{"row":i32, "column":i32})
                                n1508 = Bundle By Name(cluster=cluster{"row":i32, "column":i32} {"row"=3, "column"=10} ("start (-1, -1)"), "row"=w2258, "column"=w2256) -> (w2264:cluster{"row":i32, "column":i32})
                                n1509 = call <vilib>:"Excel Easy Text.vi"("report in"=w2252, "font"=T23 {"font name"="", "font size"=11.0, "bold"=1, "italic"=0, "underline"=0, "strike through"=0, "font color"=16777216}, "text"=w2251, "start (-1, -1)"=w2264, "end (-1, -1)"=w2254, "error in (no error)"=w2253) -> ("report out"=w2274:refnum<class "NI_report.lvclass">, "next cell bottom-left"=w2272:cluster{"row":i32, "column":i32}, "next cell top-right"=w2271:cluster{"row":i32, "column":i32}, "error out"=w2273:errorcluster)  [unwired: 5 in, 1 out]
                                n1510 = Bundle By Name(cluster=cluster{"row":i32, "column":i32} {"row"=3, "column"=10} ("start (-1, -1)"), "row"=w2263, "column"=w2256) -> (w2262:cluster{"row":i32, "column":i32})
                                n1511 = call <vilib>:"Excel Set Cell Alignment.vi"("report in"=w2274, "vertical alignment (top)"=w2270, "horizontal alignment (left)"=w2270, "start (-1, -1)"=w2272, "end (-1, -1)"=w2271, "error in (no error)"=w2273) -> ("report out"=w2269:refnum<class "NI_report.lvclass">, "error out"=w2268:errorcluster)  [unwired: 8 in]
                                n1512 = call <vilib>:"Excel Set Cell Color and Border.vi"("report in"=w2269, "outside border"=T24 {"on/off"=TRUE, "weight"=2, "color"=0}, "background color (w)"=u32 16777215, "start (-1, -1)"=w2262, "end (-1, -1)"=w2254, "error in (no error)"=w2268) -> ()  [unwired: 8 in, 2 out]
                                }
                                frame #3 {
                                n1513 = stacked-sequence {
                                seq-local: [w2280 _] -> [_ w2319]
                                seq-local: [w2279 _] -> [_ w2320]
                                tunnel: w2278 -> [w2283 _]
                                tunnel: w2277 -> [w2282 _]
                                tunnel: w2276 -> [w2281 _]
                                tunnel: w2275 -> [_ w2321]
                                frame #0 {
                                # "Cal-mode"
                                n1514 = stacked-sequence {
                                tunnel: w2283 -> [w2295 w2316]
                                tunnel: w2282 -> [w2294 w2315]
                                tunnel: w2281 -> [w2284 w2298]
                                tunnel: [_ w2297] -> w2280
                                tunnel: [_ w2296] -> w2279
                                frame #0 {
                                # "Load(lb)"
                                n1515 = Index Array(array=w2284, index (row)=0 ("인덱스 (행)")) -> (element=w2291:string[])  [unwired: 1 in]
                                n1516 = Replace Array Subset(array=w2291, new element="Offset" ("새 원소/부분배열"), index=0 ("인덱스")) -> (w2288:string[])
                                n1517 = Build Array(w2288) -> (w2287:string[][])
                                n1518 = Transpose 2D Array(2D array=w2287) -> (transposed array=w2286:string[][])
                                n1519 = call-poly <vilib>:"Excel Easy Table.vi"("report in"=w2295, "font"=T23 {"font name"="", "font size"=11.0, "bold"=0, "italic"=0, "underline"=0, "strike through"=0, "font color"=16777216}, "start (0, 0)"=cluster{"row":i32, "column":i32} {"row"=15, "column"=1}, "text data"=w2286, "error in (no error)"=w2294) -> ()  [unwired: 6 in, 5 out]
                                }
                                frame #1 {
                                # "Load(lb)"
                                n1520 = Index Array(array=w2298, index (row) #1=1 ("인덱스 (행)"), index (row) #2=2 ("인덱스 (행)"), index (row) #3=3 ("인덱스 (행)")) -> (element #1=w2309:string[], element #2=w2308:string[], element #3=w2307:string[])  [unwired: 3 in]
                                n1521 = Index Array(array=w2298, index (row) #1=5 ("인덱스 (행)"), index (row) #2=6 ("인덱스 (행)"), index (row) #3=7 ("인덱스 (행)")) -> (element #1=w2306:string[], element #2=w2305:string[], element #3=w2304:string[])  [unwired: 3 in]
                                n1522 = Build Array(w2306, w2305, w2304) -> (w2302:string[][])
                                n1523 = Build Array(w2309, w2308, w2307) -> (w2303:string[][])
                                n1524 = Build Array (concatenate)(w2303, w2302) -> (w2301:string[][])
                                n1525 = Transpose 2D Array(2D array=w2301) -> (transposed array=w2300:string[][])
                                n1526 = call-poly <vilib>:"Excel Easy Table.vi"("report in"=w2316, "font"=T23 {"font name"="", "font size"=11.0, "bold"=0, "italic"=0, "underline"=0, "strike through"=0, "font color"=16777216}, "start (0, 0)"=cluster{"row":i32, "column":i32} {"row"=15, "column"=3}, "text data"=w2300, "error in (no error)"=w2315) -> ("report out"=w2297:refnum<class "NI_report.lvclass">, "error out"=w2296:errorcluster)  [unwired: 6 in, 3 out]
                                }
                                }
                                }
                                frame #1 {
                                # "Test-mode"
                                n1527 = stacked-sequence {
                                tunnel: w2319 -> [w2333 w2352]
                                tunnel: w2320 -> [w2332 w2351]
                                tunnel: w2321 -> [w2322 w2334]
                                frame #0 {
                                # "Load(lb)"
                                n1528 = Index Array(array=w2322, index (row)=0 ("인덱스 (행)")) -> (element=w2329:string[])  [unwired: 1 in]
                                n1529 = Replace Array Subset(array=w2329, new element="Offset" ("새 원소/부분배열"), index=0 ("인덱스")) -> (w2326:string[])
                                n1530 = Build Array(w2326) -> (w2325:string[][])
                                n1531 = Transpose 2D Array(2D array=w2325) -> (transposed array=w2324:string[][])
                                n1532 = call-poly <vilib>:"Excel Easy Table.vi"("report in"=w2333, "font"=T23 {"font name"="", "font size"=11.0, "bold"=0, "italic"=0, "underline"=0, "strike through"=0, "font color"=16777216}, "start (0, 0)"=cluster{"row":i32, "column":i32} {"row"=25, "column"=1}, "text data"=w2324, "error in (no error)"=w2332) -> ()  [unwired: 6 in, 5 out]
                                }
                                frame #1 {
                                # "Load(lb)"
                                n1533 = Index Array(array=w2334, index (row) #1=1 ("인덱스 (행)"), index (row) #2=2 ("인덱스 (행)"), index (row) #3=3 ("인덱스 (행)")) -> (element #1=w2345:string[], element #2=w2344:string[], element #3=w2343:string[])  [unwired: 3 in]
                                n1534 = Index Array(array=w2334, index (row) #1=5 ("인덱스 (행)"), index (row) #2=6 ("인덱스 (행)"), index (row) #3=7 ("인덱스 (행)")) -> (element #1=w2342:string[], element #2=w2341:string[], element #3=w2340:string[])  [unwired: 3 in]
                                n1535 = Build Array(w2342, w2341, w2340) -> (w2338:string[][])
                                n1536 = Build Array(w2345, w2344, w2343) -> (w2339:string[][])
                                n1537 = Build Array (concatenate)(w2339, w2338) -> (w2337:string[][])
                                n1538 = Transpose 2D Array(2D array=w2337) -> (transposed array=w2336:string[][])
                                n1539 = call-poly <vilib>:"Excel Easy Table.vi"("report in"=w2352, "font"=T23 {"font name"="", "font size"=11.0, "bold"=0, "italic"=0, "underline"=0, "strike through"=0, "font color"=16777216}, "start (0, 0)"=cluster{"row":i32, "column":i32} {"row"=25, "column"=3}, "text data"=w2336, "error in (no error)"=w2351) -> ()  [unwired: 6 in, 5 out]
                                }
                                }
                                }
                                }
                                }
                                }
                                n1540 = call-dynamic "Save Report to File.vi"("report in"=w2223, "report file path"=w2217, "error in (no error)"=w2222) -> ()  [unwired: 11 in, 2 out]
                                }
                                }
                                n1541 = control-ref of="Test Status"() -> (w2183:refnum<vi>)
                                n1542 = call "SUB-Status string update.vi"("String In"="Result Data Process\n" ("Force Test Status"), "Add Date"=TRUE ("날짜추가"), "reference"=w2183) -> ()  [unwired: 2 in, 1 out]
                                n1543 = local write "FTS OP status"(T8 "Test_End" ("FTS OP status")) -> ()
                                }
                                frame Enabled {
                                }
                              }
                            }
                            frame "Test_End", Default {
                              # "Test_End"
                              n1544 = control-ref of="Test Status"() -> (w2358:refnum<vi>)
                              n1545 = local write "Mark10 Gauge (lb)"(0.0 ("Mark10 Gauge")) -> ()
                              n1546 = local write "Clear graph 1"(TRUE ("그래프 지우기")) -> ()
                              n1547 = call "SUB-Status string update.vi"("String In"="Test complete." ("Force Test Status"), "Add Date"=TRUE ("날짜추가"), "reference"=w2358) -> ()  [unwired: 2 in, 1 out]
                              n1548 = call <vilib>:"Beep.vi"() -> ()  [unwired: 12 in]
                              n1549 = call "SUB-BLE Rx data Clear.vi"() -> ()  [unwired: 6 in]
                            }
                            frame "Gen_Report" {
                              n1550 = control-ref of="ROM Table 2"() -> (w2367:refnum<vi>)
                              n1551 = property on="프로퍼티 노드" class="Tbl (엄격한)"(reference=w2367) -> ("Value"=w2368:string[][])  [unwired: 1 in, 2 out]
                              n1552 = local read "Test name"() -> (w2375:string)
                              n1553 = call "SUB_Parsing_from_table_to_cluster.vi"("ROM Table"=w2368) -> ("Device information"=w2366:T1)  [unwired: 10 in, 8 out]
                              n1554 = Format Date/Time String(time format string (%c)="%Y%m%d %H%M%S" ("상태")) -> (date/time string=w2374:string)  [unwired: 2 in]
                              n1555 = control-ref of="Test Status"() -> (w2377:refnum<vi>)
                              n1556 = Format Into String(format string="GEN4 FTS-%s (%s).xlsm" ("상태"), w2374, w2375) -> (resulting string=w2372:string)  [unwired: 2 in, 1 out]
                              n1557 = call "SUB-Status string update.vi"("String In"="Result Data Process\n" ("Force Test Status"), "Add Date"=TRUE ("날짜추가"), "reference"=w2377) -> ()  [unwired: 2 in, 1 out]
                              n1558 = call "Sub_Report_Generation.vi"("File Name"=w2372) -> ("error out"=w2371:errorcluster, "cal fac B"=w2361:dbl, "cal fac A"=w2362:dbl)  [unwired: 8 in]
                              "scale A" <- w2362
                              "scale B" <- w2361
                              n1559 = disable-structure shown="비활성화" {
                                frame Disabled {
                                n1560 = Multiply(y=2097152.0) -> (x*y=w2380:dbl)  [unwired: 1 in]
                                n1561 = Round Toward -Infinity(1:w2380) -> ()  [unwired: 1 out]
                                }
                                frame Enabled {
                                }
                              }
                              n1562 = case shown="에러" w2371 {
                                frame No Error {
                                }
                                frame Error {
                                n1563 = One Button Dialog(message="Report Generation Error" ("메시지")) -> ()  [unwired: 1 in, 1 out]
                                }
                              }
                              n1564 = To Unsigned Byte Integer(number=w2361) -> (unsigned 8bit integer=w2364:u8)
                              "cal factor B" <- w2364
                              n1565 = To Unsigned Byte Integer(number=w2362) -> (unsigned 8bit integer=w2365:u8)
                              "cal factor A" <- w2365
                              n1566 = Bundle By Name(cluster=w2366, "Scale A"=w2365, "Scale B"=w2364) -> (→"scale A,B":T1)
                              n1567 = local write "FTS OP status"(T8 "Test_End" ("FTS OP status")) -> ()
                            }
                          }
                        }
                      }
                      frame #4 {
                        n1568 = flat-sequence {
                          frame #0 {
                            n1569 = local write "FTS comm."(FALSE ("FTS 수신 정상")) -> ()
                            n1570 = local write "FTS Testing"(FALSE ("FTS 시험 진행")) -> ()
                            n1571 = local write "FTS start"(FALSE ("Test Start")) -> ()
                          }
                          frame #1 {
                            n1572 = Wait (ms)(milliseconds to wait=u32 1000 ("대기 시간(ms)")) -> ()  [unwired: 1 out]
                          }
                          frame #2 {
                            n1573 = local write "scale A.B Tx"(TRUE ("scale A.B")) -> ()
                          }
                        }
                      }
                    }
                  }
                }
              }
            }
          }
          frame #5 {
            # "Battery Calibration"
            n1574 = local read "Comm con status 1"() -> (w2387:bool)
            n1575 = case shown="참" w2387 {
              frame False {
              }
              frame True {
                n1576 = stacked-sequence {
                  frame #0 {
                    # "ADC Linearity Start"
                    n1577 = case shown="참" "ADC Linearity Start" {
                      frame False {
                      }
                      frame True {
                        w2390 = dbl[] []
                        n1578 = local write "battery cal complete boolean"(FALSE ("불리언 2")) -> ()
                        n1579 = while {
                          shift-right: [w2399] -> _
                          shift-left: 0.5 ("Voltage(V)") -> [w2400]
                          shift-right: [w2398] -> _
                          shift-left: w2390 -> [w2397]
                          shift-right: [w2396] -> _
                          shift-left: w2390 -> [w2395]
                          stop <- w2393 stop-if-true
                          n1580 = Wait (ms)(milliseconds to wait=u32 100 ("대기 시간(ms)")) -> ()  [unwired: 1 out]
                          n1581 = case shown="\"Measurement\"" "Linerity State" {
                            tunnel: w2400 -> [w2401 w2412 w2440]
                            tunnel: [w2401 w2420 w2440] -> w2399
                            tunnel: [w2403 w2416 _] -> w2398
                            tunnel: w2397 -> [_ w2419 _]
                            tunnel: [w2403 w2411 _] -> w2396
                            tunnel: w2395 -> [_ w2417 _]
                            tunnel: [_ _ w2439] -> w2393
                            frame "Initial", Default {
                              w2403 = dbl[] []
                              n1582 = control-ref of="Linearity monitoring graph"() -> (w2406:refnum<vi>)
                              n1583 = property class="XYGraph (엄격한)"(reference=w2406, "Value"=cluster{dbl[], dbl[]} {[], []} ("값")) -> ()  [unwired: 1 in, 2 out]
                              n1584 = control-ref of="Linerity State"() -> (w2405:refnum<vi>)
                              n1585 = property class="Enum (엄격한)"(reference=w2405, "Value"=Linerity_State."Measurement" ("Linerity State")) -> ()  [unwired: 1 in, 2 out]
                            }
                            frame "Measurement" {
                              n1586 = Greater Or Equal?(x=w2412, y=3.0) -> (x >= y?=w2413:bool)
                              n1587 = stacked-sequence {
                                tunnel: [_ _ _ w2423 _] -> w2418
                                tunnel: w2413 -> [_ _ _ _ w2434]
                                frame #0 {
                                # "Wait for 1sec to Voltage Stable"
                                }
                                frame #1 {
                                # "BLE Rx Buffer Clear"
                                n1588 = call "SUB-BLE Rx data Clear.vi"() -> ()  [unwired: 6 in]
                                }
                                frame #2 {
                                # "500ms data received (50 Packets at 10ms interval time)"
                                n1589 = Wait (ms)(milliseconds to wait=u32 500 ("대기 시간(ms)")) -> ()  [unwired: 1 out]
                                }
                                frame #3 {
                                # "Rx data & Average"
                                n1590 = for {
                                N: 50 -> [_]
                                tunnel: [w2428] -> w2426 mode=indexing
                                n1591 = call "SUB-BLE Rx data (Mon)-Wait.vi"("Timeout(ms)"=u16 100) -> ("RxReady"=w2430:bool)  [unwired: 4 in]
                                n1592 = case shown="참" w2430 {
                                tunnel: [u16 0 ("Bat") w2432] -> w2428
                                frame False {
                                }
                                frame True {
                                n1593 = call "SUB-BLE Rx data (Mon)-Classify.vi"() -> ("data out"=w2433:u8[])  [unwired: 5 in, 4 out]
                                n1594 = call "SUB-BLE Rx data (Mon)-CDC IMU.vi"("data in"=w2433) -> ("Bat"=w2432:u16)  [unwired: 4 in, 3 out]
                                }
                                }
                                }
                                n1595 = To Double Precision Float(number=w2426) -> (double precision float=w2425:dbl[])
                                n1596 = call-poly <vilib>:"Mean.vi"("X"=w2425) -> ("mean"=w2424:dbl)  [unwired: 1 out]
                                n1597 = Round Toward -Infinity(1:w2424) -> (0:w2423:dbl)
                                }
                                frame #4 {
                                n1598 = case shown="참" w2434 {
                                tunnel: [Linerity_State."End" ("Linerity State") Linerity_State."Measurement" ("Linerity State")] -> w2435
                                frame True {
                                }
                                frame False {
                                }
                                }
                                n1599 = control-ref of="Linerity State"() -> (w2436:refnum<vi>)
                                n1600 = property class="Enum (엄격한)"(reference=w2436, "Value"=w2435) -> ()  [unwired: 1 in, 2 out]
                                }
                              }
                              n1601 = Wait (ms)(milliseconds to wait=u32 1000 ("대기 시간(ms)")) -> ()  [unwired: 1 out]
                              n1602 = Add(x=w2412, y=0.5 ("x")) -> (x+y=w2420:dbl)
                              n1603 = Build Array (concatenate)(w2419, w2412) -> (w2416:dbl[])
                              n1604 = Build Array (concatenate)(w2417, w2418) -> (w2411:dbl[])
                              "battery cal value" <- w2411
                              n1605 = Bundle(w2416, w2411) -> (→"Linearity monitoring graph":cluster{dbl[], dbl[]})  [unwired: 1 in]
                              n1606 = control-ref of="Linerity State"() -> (w2408:refnum<vi>)
                              n1607 = property class="Enum (엄격한)"(reference=w2408, "Value"=Linerity_State."End" ("Linerity State")) -> ()  [unwired: 1 in, 2 out]
                              n1608 = local write "Status"("Testing.." ("문자열")) -> ()
                            }
                            frame "End" {
                              n1609 = while {
                                tunnel: [w2443] -> w2439
                                stop <- w2443 stop-if-true
                                w2443 = TRUE ("불리언 2")
                                n1610 = property on="battery cal value" class="Arr (엄격한)"() -> ("Value"=w2444:dbl[])  [unwired: 2 in, 2 out]
                                n1611 = flat-sequence {
                                tunnel: [w2464] -> w2442
                                tunnel: [w2463] -> w2441
                                tunnel: w2444 -> [w2465]
                                tunnel: w2442 -> [w2471]
                                tunnel: w2441 -> [w2470]
                                frame #0 {
                                n1612 = call-poly <vilib>:"Mean.vi"("X"=w2465) -> ("mean"=w2455:dbl)  [unwired: 1 out]
                                n1613 = Multiply(x=w2455, y=0.6) -> (x*y=w2458:dbl)
                                n1614 = Divide(x=w2458, y=0.166667) -> (x/y=w2460:dbl)
                                n1615 = Divide(x=w2460, y=4096.0) -> (x/y=w2461:dbl)
                                "x/y" <- w2461
                                n1616 = Add(x=w2461, y=0.17) -> (x+y=w2453:dbl)
                                "Battery(V)" <- w2453
                                n1617 = Divide(x=w2453, y=0.6) -> (x/y=w2451:dbl)
                                n1618 = Multiply(x=w2451, y=0.166667) -> (x*y=w2450:dbl)
                                n1619 = Multiply(x=4096.0 ("y"), y=w2450) -> (x*y=w2448:dbl)
                                n1620 = To Unsigned Word Integer(number=w2448) -> (unsigned 16bit integer=w2447:u16)
                                n1621 = Split Number(x=w2447) -> (hi(x)=w2446:u8, lo(x)=w2445:u8)
                                n1622 = To Unsigned Byte Integer(number=w2446) -> (unsigned 8bit integer=w2464:u8)
                                n1623 = To Unsigned Byte Integer(number=w2445) -> (unsigned 8bit integer=w2463:u8)
                                }
                                frame #1 {
                                n1624 = control-ref of="ROM Table 2"() -> (w2467:refnum<vi>)
                                n1625 = property on="프로퍼티 노드" class="Tbl (엄격한)"(reference=w2467) -> ("Value"=w2468:string[][])  [unwired: 1 in, 2 out]
                                n1626 = call "SUB_Parsing_from_table_to_cluster.vi"("ROM Table"=w2468) -> ("Cal information"=w2469:T14)  [unwired: 10 in, 8 out]
                                n1627 = Bundle By Name(cluster=w2469, "Voltage H 3.1V"=w2471, "Voltage L 3.1V"=w2470) -> (→"Cal information":T14)
                                }
                                frame #2 {
                                n1628 = control-ref of="Linerity State"() -> (w2475:refnum<vi>)
                                n1629 = property class="Enum (엄격한)"(reference=w2475, "Value"=Linerity_State."Initial" ("Linerity State")) -> ()  [unwired: 1 in, 2 out]
                                n1630 = local write "battery cal complete boolean"(TRUE ("불리언 2")) -> ()
                                n1631 = local write "battery cal Tx"(TRUE ("불리언 2")) -> ()
                                n1632 = local write "ADC Linearity Start"(FALSE ("ADC Linearity Start")) -> ()
                                }
                                }
                              }
                            }
                          }
                        }
                      }
                    }
                    "inspection boolean" <- "ADC Linearity Start"
                  }
                }
              }
            }
          }
          frame #6 {
            # "Read at Manual Test"
            n1633 = call "SUB-BLE Rx data (Set)-Classify.vi"() -> ("data out"=w2477:u8[], "Rx-data"=w2478:bool)  [unwired: 4 in]
            n1634 = case shown="참" w2478 {
              tunnel: w2477 -> [_ w2481]
              frame False {
              }
              frame True {
                n1635 = flat-sequence {
                  tunnel: w2481 -> [w2483]
                  tunnel: [w2483] -> w2479
                  tunnel: [w2485] -> w2480
                  tunnel: w2479 -> [w2485]
                  tunnel: w2480 -> [w2487]
                  frame #0 {
                    n1636 = local write "Data_mon(h)"("" ("Data_mon")) -> ()
                  }
                  frame #1 {
                    n1637 = Wait (ms)(milliseconds to wait=u32 20 ("대기 시간(ms)")) -> ()  [unwired: 1 out]
                  }
                  frame #2 {
                    n1638 = Byte Array To String(unsigned byte array=w2487) -> (string=→"Data_mon(h)":string)
                    n1639 = local read "Data Log"() -> (w2486:string)
                    n1640 = call <vilib>:"Space Constant.vi"() -> ("String"=w2492:string)
                    n1641 = Format Date/Time String(time format string (%c)="%H:%M:%S%3u>  " ("상태")) -> (date/time string=w2491:string)  [unwired: 2 in]
                    n1642 = Array To Spreadsheet String(delimiter (Tab)=w2492, array=w2487, 3:"%02X" ("포맷 문자열")) -> (spreadsheet string=w2489:string)
                    n1643 = Concatenate Strings(w2491, w2489, w2486) -> (w2488:string)
                    n1644 = local write "Data Log"(w2488) -> ()
                    "data out" <- w2487
                  }
                }
              }
            }
          }
          frame #7 {
            n1645 = local read "Comm con status 1"() -> (w2495:bool)
            n1646 = case shown="거짓" w2495 {
              frame False {
              }
              frame True {
              }
            }
          }
          frame #8 {
            # "Reset"
            n1647 = local read "Comm con status 1"() -> (w2501:bool)
            n1648 = local read "Clear graph 1"() -> (w2500:bool)
            n1649 = Not(x=w2501) -> (.not. x?=w2498:bool)
            n1650 = case shown="참" w2498 {
              frame False {
              }
              frame True {
                n1651 = local write "status string"("Ready (available after the communication connection)" ("status string")) -> ()
              }
            }
            n1652 = case shown="참" w2500 {
              frame False {
              }
              frame True {
                n1653 = local write "Clear graph 1"(FALSE ("그래프 지우기")) -> ()
                n1654 = call "SUB-BLE Rx data Clear.vi"() -> ()  [unwired: 6 in]
                n1655 = property on="CDC(PCAP02) Graph" class="WFChart (엄격한)"("History Data"=waveform(dbl)[][] [] ("히스토리 데이터")) -> ()  [unwired: 2 in, 2 out]
              }
            }
            n1656 = local read "Export graph 1"() -> (w2499:bool)
            n1657 = local read "Export graph2"() -> (w2497:bool)
            n1658 = local read "Clear graph 2"() -> (w2496:bool)
            n1659 = case shown="참" w2497 {
              frame False {
              }
              frame True {
                n1660 = invoke on="IMU Graph" class="WFChart (엄격한)" method="Export Data to Excel"() -> ()  [unwired: 3 in, 3 out]
                n1661 = local write "Export graph2"(FALSE ("그래프 반출")) -> ()
              }
            }
            n1662 = case shown="참" w2499 {
              frame False {
              }
              frame True {
                n1663 = invoke on="CDC(PCAP02) Graph" class="WFChart (엄격한)" method="Export Data to Excel"() -> ()  [unwired: 3 in, 3 out]
                n1664 = local write "Export graph 1"(FALSE ("그래프 반출")) -> ()
              }
            }
            n1665 = case shown="참" w2496 {
              frame False {
              }
              frame True {
                n1666 = local write "Clear graph 2"(FALSE ("그래프 지우기")) -> ()
                n1667 = call "SUB-BLE Rx data Clear.vi"() -> ()  [unwired: 6 in]
                n1668 = property on="IMU Graph" class="WFChart (엄격한)"("History Data"=waveform(dbl)[][] [] ("히스토리 데이터")) -> ()  [unwired: 2 in, 2 out]
              }
            }
          }
          frame #9 {
            # "Offset (Save)"
            n1669 = local read "Comm con status 1"() -> (w2511:bool)
            n1670 = local read "Comm con status 1"() -> (w2512:bool)
            n1671 = local read "Offset 2"() -> (w2510:bool)
            n1672 = local read "Offset 1"() -> (w2513:bool)
            n1673 = And(x=w2511, y=w2510) -> (x .and. y?=w2509:bool)
            n1674 = And(x=w2512, y=w2513) -> (x .and. y?=w2514:bool)
            n1675 = case shown="참" w2509 {
              frame False {
                n1676 = local write "Offset 2"(FALSE ("Offset 1")) -> ()
              }
              frame True {
                n1677 = local write "Offset 2"(FALSE ("Offset 1")) -> ()
                n1678 = local write "Clear graph 2"(TRUE ("그래프 지우기")) -> ()
                n1679 = for {
                  N: 50 -> [_]
                  tunnel: [w2585] -> w2563 mode=indexing
                  tunnel: [w2584] -> w2564 mode=indexing
                  tunnel: [w2583] -> w2565 mode=indexing
                  tunnel: [w2582] -> w2566 mode=indexing
                  tunnel: [w2581] -> w2567 mode=indexing
                  tunnel: [w2580] -> w2568 mode=indexing
                  n1680 = local read "IMU Offet"() -> (w2579:T11)
                  n1681 = call "SUB-BLE Rx data (Mon)-Wait.vi"("Timeout(ms)"=u16 200) -> ("RxReady"=w2586:bool)  [unwired: 4 in]
                  n1682 = case shown="참" w2586 {
                    tunnel: [w2589 w2591] -> w2578
                    tunnel: w2579 -> [w2589 _]
                    frame False {
                    }
                    frame True {
                      n1683 = call "SUB-BLE Rx data (Mon)-Classify.vi"() -> ("data out"=w2592:u8[], "Rx-mon"=w2590:bool)  [unwired: 5 in, 3 out]
                      n1684 = case shown="참" w2590 {
                        tunnel: w2592 -> [_ w2594]
                        tunnel: [_ w2593] -> w2591
                        frame False {
                        }
                        frame True {
                          n1685 = call "SUB-BLE Rx data (Mon)-CDC IMU.vi"("data in"=w2594) -> ("IMU data"=w2593:T11)  [unwired: 4 in, 3 out]
                        }
                      }
                    }
                  }
                  n1686 = Unbundle By Name(w2578) -> ("Gyroscope X"=w2585:dbl, "Gyroscope Y"=w2584:dbl, "Gyroscope Z"=w2583:dbl, "Accelerometer X"=w2582:dbl, "Accelerometer Y"=w2581:dbl, "Accelerometer Z"=w2580:dbl)
                  n1687 = Wait Until Next ms Multiple(millisecond multiple=u32 20 ("ms 배수")) -> ()  [unwired: 1 out]
                }
                n1688 = call-poly <vilib>:"Mean.vi"("X"=w2563) -> ("mean"=w2570:dbl)  [unwired: 1 out]
                n1689 = call-poly <vilib>:"Mean.vi"("X"=w2564) -> ("mean"=w2571:dbl)  [unwired: 1 out]
                n1690 = call-poly <vilib>:"Mean.vi"("X"=w2565) -> ("mean"=w2572:dbl)  [unwired: 1 out]
                n1691 = call-poly <vilib>:"Mean.vi"("X"=w2566) -> ("mean"=w2573:dbl)  [unwired: 1 out]
                n1692 = call-poly <vilib>:"Mean.vi"("X"=w2567) -> ("mean"=w2574:dbl)  [unwired: 1 out]
                n1693 = call-poly <vilib>:"Mean.vi"("X"=w2568) -> ("mean"=w2575:dbl)  [unwired: 1 out]
                n1694 = Bundle By Name(cluster=T11 {"Gyroscope X"=0.0, "Gyroscope Y"=0.0, "Gyroscope Z"=0.0, "Accelerometer X"=0.0, "Accelerometer Y"=0.0, "Accelerometer Z"=0.0} ("IMU data"), "Gyroscope X"=w2570, "Gyroscope Y"=w2571, "Gyroscope Z"=w2572, "Accelerometer X"=w2573, "Accelerometer Y"=w2574, "Accelerometer Z"=w2575) -> (w2569:T11)
                n1695 = local write "IMU Offet"(w2569) -> ()
              }
            }
            n1696 = case shown="참" w2514 {
              frame False {
                n1697 = local write "Offset 1"(FALSE ("Offset 1")) -> ()
              }
              frame True {
                n1698 = local write "Offset 1"(FALSE ("Offset 1")) -> ()
                n1699 = local write "Clear graph 1"(TRUE ("그래프 지우기")) -> ()
                n1700 = local read "Offset Souce"() -> (w2518:enum32{"Normal", "Raw"})
                n1701 = Equal?(x=w2518, y=enum32{"Normal", "Raw"}."Normal" ("Offset Souce")) -> (x = y?=w2516:bool)
                n1702 = for {
                  N: 50 -> [_]
                  tunnel: [w2544] -> w2532 mode=indexing
                  tunnel: [w2543] -> w2531 mode=indexing
                  tunnel: [w2542] -> w2530 mode=indexing
                  tunnel: [w2541] -> w2529 mode=indexing
                  tunnel: [w2540] -> w2528 mode=indexing
                  tunnel: [w2539] -> w2527 mode=indexing
                  tunnel: w2516 -> [w2536]
                  n1703 = local read "CDC Offet"() -> (w2537:T10)
                  n1704 = call "SUB-BLE Rx data (Mon)-Wait.vi"("Timeout(ms)"=u16 200) -> ("RxReady"=w2545:bool)  [unwired: 4 in]
                  n1705 = case shown="참" w2545 {
                    tunnel: [w2548 w2551] -> w2538
                    tunnel: w2537 -> [w2548 _]
                    tunnel: w2536 -> [_ w2549]
                    frame False {
                    }
                    frame True {
                      n1706 = call "SUB-BLE Rx data (Mon)-Classify.vi"() -> ("data out"=w2552:u8[], "Rx-mon"=w2550:bool)  [unwired: 5 in, 3 out]
                      n1707 = case shown="거짓" w2550 {
                        tunnel: w2552 -> [w2557 w2559]
                        tunnel: [w2556 w2558] -> w2551
                        tunnel: w2549 -> [w2555 _]
                        frame False {
                          n1708 = call "SUB-BLE Rx data (Debug)-CDC.vi"("data in"=w2557) -> ("CDC debug"=w2553:T10, "CDC mon"=w2554:T10)  [unwired: 6 in]
                          n1709 = Select(t=w2554, s=w2555, f=w2553) -> (s? t:f=w2556:T10)
                        }
                        frame True {
                          n1710 = call "SUB-BLE Rx data (Mon)-CDC IMU.vi"("data in"=w2559) -> ("CDC data"=w2558:T10)  [unwired: 4 in, 3 out]
                        }
                      }
                    }
                  }
                  n1711 = Unbundle By Name(w2538) -> ("Left Wing-A, C1/C0"=w2544:dbl, "Left Wing-B, C2/C0"=w2543:dbl, "Left Wing-C, C3/C0"=w2542:dbl, "Right Wing-A, C4/C0"=w2541:dbl, "Right Wing-B, C5/C0"=w2540:dbl, "Right Wing-C, C6/C0"=w2539:dbl)
                  n1712 = Wait Until Next ms Multiple(millisecond multiple=u32 20 ("ms 배수")) -> ()  [unwired: 1 out]
                }
                n1713 = call-poly <vilib>:"Mean.vi"("X"=w2532) -> ("mean"=w2524:dbl)  [unwired: 1 out]
                n1714 = call-poly <vilib>:"Mean.vi"("X"=w2531) -> ("mean"=w2523:dbl)  [unwired: 1 out]
                n1715 = call-poly <vilib>:"Mean.vi"("X"=w2530) -> ("mean"=w2522:dbl)  [unwired: 1 out]
                n1716 = call-poly <vilib>:"Mean.vi"("X"=w2529) -> ("mean"=w2521:dbl)  [unwired: 1 out]
                n1717 = call-poly <vilib>:"Mean.vi"("X"=w2528) -> ("mean"=w2520:dbl)  [unwired: 1 out]
                n1718 = call-poly <vilib>:"Mean.vi"("X"=w2527) -> ("mean"=w2519:dbl)  [unwired: 1 out]
                n1719 = Bundle By Name(cluster=T10 {"Left Wing-A, C1/C0"=0.0, "Left Wing-B, C2/C0"=0.0, "Left Wing-C, C3/C0"=0.0, "Right Wing-A, C4/C0"=0.0, "Right Wing-B, C5/C0"=0.0, "Right Wing-C, C6/C0"=0.0} ("CDC data"), "Left Wing-A, C1/C0"=w2524, "Left Wing-B, C2/C0"=w2523, "Left Wing-C, C3/C0"=w2522, "Right Wing-A, C4/C0"=w2521, "Right Wing-B, C5/C0"=w2520, "Right Wing-C, C6/C0"=w2519) -> (w2525:T10)
                n1720 = local write "CDC Offet"(w2525) -> ()
              }
            }
          }
          frame #10 {
            # "Logging-GUI data"
            n1721 = disable-structure shown="비활성화" {
              frame Disabled {
                n1722 = local read "Data Logging"() -> (w2595:bool)
                n1723 = case shown="참" w2595 {
                  frame False {
                    n1724 = local read "Logging No."() -> (w2597:u32)
                    n1725 = Not Equal To 0?(x=w2597) -> (x != 0?=w2596:bool)
                    n1726 = case shown="참" w2596 {
                      frame False {
                      }
                      frame True {
                        n1727 = local read "log refnum"() -> (w2599:refnum<file>)
                        n1728 = local write "Logging No."(u32 0 ("Logging No.")) -> ()
                        n1729 = Close File(refnum=w2599) -> ()  [unwired: 1 in, 2 out]
                      }
                    }
                  }
                  frame True {
                    n1730 = stacked-sequence {
                      seq-local: [w2600 _] -> [_ w2652]
                      frame #0 {
                        n1731 = local read "IMU data"() -> (w2603:T11)
                        n1732 = local read "CDC data"() -> (w2620:T10)
                        n1733 = Unbundle By Name(w2620) -> ("Left Wing-A, C1/C0"=w2617:dbl, "Left Wing-B, C2/C0"=w2616:dbl, "Left Wing-C, C3/C0"=w2615:dbl, "Right Wing-A, C4/C0"=w2614:dbl, "Right Wing-B, C5/C0"=w2613:dbl, "Right Wing-C, C6/C0"=w2612:dbl)
                        n1734 = Unbundle By Name(w2603) -> ("Gyroscope X"=w2606:dbl, "Gyroscope Y"=w2607:dbl, "Gyroscope Z"=w2608:dbl, "Accelerometer X"=w2609:dbl, "Accelerometer Y"=w2610:dbl, "Accelerometer Z"=w2611:dbl)
                        n1735 = Format Into String(format string="%.7f,%.7f,%.7f,%.7f,%.7f,%.7f," ("포맷 문자열"), initial string=",,(GUI) CDC Data," ("포맷 문자열"), w2617, w2616, w2615, w2614, w2613, w2612) -> (resulting string=w2602:string)  [unwired: 1 in, 1 out]
                        n1736 = Format Into String(format string="%.6f,%.6f,%.6f,%.6f,%.6f,%.6f," ("포맷 문자열"), initial string=",(GUI) IMU Data," ("포맷 문자열"), w2606, w2607, w2608, w2609, w2610, w2611) -> (resulting string=w2601:string)  [unwired: 1 in, 1 out]
                        n1737 = Concatenate Strings(w2602, w2601) -> (w2600:string)
                      }
                      frame #1 {
                        w2646 = T33 1 items=["사용자 홈"=0, "사용자 데스크탑"=1, "사용자 문서"=2, "사용자 어플리케이션 데이터"=3, "사용자 환경"=4, "사용자 임시"=5, "퍼블릭 문서"=6, "퍼블릭 어플리케이션 데이터"=7, "퍼블릭 환경"=8, "퍼블릭 캐시"=13, "시스템 코어 라이브러리"=9, "시스템 설치된 라이브러리"=10, "어플리케이션 파일"=11, "부팅 볼륨 루트"=12] ("system directory type")
                        # "첫행(타이틀)"
                        n1738 = local read "Log no"() -> (w2621:string)
                        n1739 = local read "Logging No."() -> (w2635:u32)
                        n1740 = Format Date/Time String(time format string (%c)="Data Logging Start...  %Y/%m/%d %H:%M:%S" ("상태")) -> (date/time string=w2626:string)  [unwired: 2 in]
                        n1741 = Format Into String(format string="\\\\GEN4 Data Logging(%s).csv" ("문자열"), w2621) -> (resulting string=w2622:string)  [unwired: 2 in, 1 out]
                        n1742 = local read "RxD"() -> (w2656:string)
                        n1743 = call <vilib>:"Get System Directory.vi"("system directory type"=w2646) -> ("system directory"=w2645:path)  [unwired: 10 in]
                        n1744 = Format Into String(format string="\\r\\n\\r\\n%s\\r\\n%s\\r\\n" ("포맷 문자열"), w2626, "No.,Time,,Type,F/W ver.,(Raw)Left Wing-A,(Raw)Left Wing-B,(Raw)Left Wing-C,(Raw)Right Wing-A,(Raw)Right Wing-B,(Raw)Right Wing-C,(Raw)CDC Status,(Raw)Gyroscope X,(Raw)Gyroscope Y,(Raw)Gyroscope Z,(Raw)Accelerometer X,(Raw)Accelerometer Y,(Raw)Accelerometer Z,,Type,(GUI)Left Wing-A,(GUI)Left Wing-B,(GUI)Left Wing-C,(GUI)Right Wing-A,(GUI)Right Wing-B,(GUI)Right Wing-C,,Type,(GUI)Gyroscope X,(GUI)Gyroscope Y,(GUI)Gyroscope Z,(GUI)Accelerometer X,(GUI)Accelerometer Y,(GUI)Accelerometer Z" ("문자열")) -> (resulting string=w2624:string)  [unwired: 2 in, 1 out]
                        n1745 = Increment(x=w2635) -> (x+1=w2651:u32)
                        n1746 = Path To String(path=w2645) -> (string=w2644:string)
                        n1747 = Equal To 0?(x=w2635) -> (x = 0?=w2633:bool)
                        n1748 = Format Date/Time String(time format string (%c)="%Y/%m/%d %H:%M:%S%3u,,RXD Raw Data," ("상태")) -> (date/time string=w2658:string)  [unwired: 2 in]
                        n1749 = Match Pattern(string=w2656, regular expression="#:" ("검색 문자열")) -> (after substring=w2654:string)  [unwired: 1 in, 3 out]
                        n1750 = Format Into String(format string="%d," ("포맷 문자열"), w2635) -> (resulting string=w2649:string)  [unwired: 2 in, 1 out]
                        n1751 = Concatenate Strings(w2644, w2622) -> (w2643:string)
                        n1752 = local write "Logging No."(w2651) -> ()
                        n1753 = String To Path(string=w2643) -> (path=w2642:path)
                        n1754 = Open/Create/Replace File(file path (use dialog)=w2642, operation (0:open)=T31."open or create" ("동작(0:open)"), access (0:read/write)=enum16{"read/write", "read-only", "write-only"}."read/write" ("접근(0:읽기/쓰기)")) -> (refnum out=w2637:refnum<file>, error out=w2636:errorcluster)  [unwired: 3 in, 1 out]
                        n1755 = Select(t=w2624, s=w2633, f="") -> (s? t:f=w2632:string)
                        n1756 = Concatenate Strings(w2649, w2658, w2654, w2652, "\r\n") -> (w2631:string)
                        n1757 = Get File Position(4:w2636, 7:w2637) -> (0:w2647:errorcluster, 2:w2634:i64, 3:w2648:refnum<file>)
                        n1758 = Concatenate Strings(w2632, w2631) -> (w2630:string)
                        n1759 = call <vilib>:"Write File+ (string).vi"("string"=w2630, "error in (no error)"=w2647, "pos offset (bytes:0)"=w2634, "refnum"=w2648) -> ("error out"=w2638:errorcluster, "dup refnum"=w2639:refnum<file>)  [unwired: 3 in, 1 out]
                        "log refnum" <- w2639
                        n1760 = disable-structure shown="비활성화" {
                          disable-tunnel: w2639 -> [w2660 _]
                          disable-tunnel: w2638 -> [w2659 _]
                          frame Disabled {
                            n1761 = Close File(refnum=w2660, error in=w2659) -> ()  [unwired: 2 out]
                          }
                          frame Enabled {
                          }
                        }
                      }
                    }
                  }
                }
              }
              frame Enabled {
              }
            }
          }
          frame #11 {
            # "Logging-BLE data"
            n1762 = disable-structure shown="비활성화" {
              disable-tunnel: [w2665 _] -> _
              frame Disabled {
                n1763 = local read "Timer-ble log"() -> (w2668:u32)
                n1764 = Tick Count (ms)() -> (millisecond timer value=w2669:u32)
                n1765 = Subtract(x=w2669, y=w2668) -> (x-y=w2667:u32)
                n1766 = Greater Or Equal?(x=w2667, y=u32 3000) -> (x >= y?=w2665:bool)
              }
              frame Enabled {
              }
            }
            n1767 = Compound Arithmetic op=AND ("복합 연산")("File Path Done", "Data Logging", "log data1") -> (w2664:bool)
            n1768 = case shown="참" w2664 {
              frame False {
              }
              frame True {
                n1769 = stacked-sequence {
                  seq-local: [w2670 _ _] -> [_ _ w2675]
                  frame #0 {
                    n1770 = local read "log ble buf"() -> (w2670:string)
                  }
                  frame #1 {
                    n1771 = Tick Count (ms)() -> (millisecond timer value=w2673:u32)
                    n1772 = local write "Timer-ble log"(w2673) -> ()
                    n1773 = local write "log data1"(FALSE ("log data1")) -> ()
                    n1774 = local write "log ble buf"("" ("log ble buf")) -> ()
                  }
                  frame #2 {
                    n1775 = String Length(string=w2675) -> (length=w2674:i32)
                    n1776 = case shown="1.." w2674 {
                      selector: w2674 -> [_ w2677]
                      tunnel: w2675 -> [_ w2679]
                      frame 0, Default {
                      }
                      frame 1.. {
                        n1777 = To Quad Integer(1:w2677) -> (0:w2676:i64)
                        n1778 = call "File_Interface.vi"("Number of byte"=w2676, "Mode"=File_Control_mode."Write", "Buffer"=w2679) -> ()  [unwired: 8 in, 1 out]
                      }
                    }
                  }
                }
              }
            }
          }
          frame #12 {
            n1779 = local write "Rx-mon"(FALSE) -> ()
            n1780 = local write "Rx-debug"(FALSE ("Rx-debug")) -> ()
          }
          frame #13 {
            # "Maximize window for debug"
            # "Maximize window"
            n1781 = local read "Maximize window"() -> (w2682:bool)
            n1782 = case shown="참" w2682 {
              frame False {
              }
              frame True {
                n1783 = First Call?() -> (First Call?: T/F=w2684:bool)
                n1784 = case shown="거짓" w2684 {
                  frame False {
                  }
                  frame True {
                    w2701 = 250  # 확장 창 크기
                    n1785 = Current VI's Path() -> (path=w2691:path)
                    n1786 = Open VI Reference(vi path=w2691) -> (vi reference=w2692:refnum<vi>, error out=w2693:errorcluster)  [unwired: 5 in]
                    n1787 = property class="VI"(reference=w2692, error in=w2693) -> (reference out=w2690:refnum<vi>, error out=w2688:errorcluster, "Front Panel.PanelBounds"=w2686:T42)
                    n1788 = Unbundle By Name(w2686) -> ("Left"=w2700:i16, "Top"=w2698:i16, "Right"=w2696:i16, "Bottom"=w2697:i16)
                    n1789 = expression code="x/2"(w2701) -> (w2695:i32)
                    n1790 = Add(x=w2696, y=w2695) -> (x+y=w2694:i32)
                    n1791 = Subtract(x=w2700, y=w2695) -> (x-y=w2699:i32)
                    n1792 = Bundle By Name(cluster=w2686, "Left"=w2699, "Top"=w2698, "Right"=w2694, "Bottom"=w2697) -> (w2685:T42)
                    n1793 = property class="VI"(reference=w2690, error in=w2688, "Front Panel.PanelBounds"=w2685) -> (reference out=w2689:refnum<vi>, error out=w2687:errorcluster)
                    n1794 = Close Reference(reference=w2689, error in (no error)=w2687) -> ()  [unwired: 1 out]
                  }
                }
                n1795 = local write "Maximize window"(FALSE ("창크게")) -> ()
              }
            }
          }
          frame #14 {
            n1796 = local read "Comm con status 1"() -> (w2703:bool)
            n1797 = case shown="참" w2703 {
              frame False {
              }
              frame True {
                n1798 = local read "ms timer 5"() -> (w2710:u32)
                n1799 = Tick Count (ms)() -> (millisecond timer value=w2709:u32)
                n1800 = Subtract(x=w2709, y=w2710) -> (x-y=w2711:u32)
                n1801 = Greater Or Equal?(x=w2711, y=u32 100) -> (x >= y?=w2707:bool)
                n1802 = case shown="참" w2707 {
                  frame False {
                  }
                  frame True {
                    n1803 = local read "Port-act 1"() -> (w2722:refnum<visa-resource-name>)
                    n1804 = property on="BLE Interval buf" class="WFChart (엄격한)"() -> ("History Data"=w2719:u32[])  [unwired: 2 in, 2 out]
                    n1805 = property on="BLE RSSI buf" class="WFChart (엄격한)"() -> ("History Data"=w2712:i16[])  [unwired: 2 in, 2 out]
                    n1806 = Tick Count (ms)() -> (millisecond timer value=w2720:u32)
                    n1807 = local write "ms timer 5"(w2720) -> ()
                    n1808 = Array Size(array=w2719) -> (size(s)=w2718:i32)
                    n1809 = Array Size(array=w2712) -> (size(s)=w2714:i32)
                    n1810 = property class="Instr"(reference=w2722) -> ("Serial Settings:Number of Bytes at Serial Port"=w2721:u32)  [unwired: 1 in, 2 out]
                    n1811 = Greater?(x=w2718, y=20) -> (0:w2717:bool)
                    n1812 = Greater?(x=w2714, y=1) -> (0:w2713:bool)
                    n1813 = case shown="참" w2717 {
                      tunnel: w2719 -> [_ w2730]
                      frame False {
                      }
                      frame True {
                        n1814 = call-poly <vilib>:"Mean.vi"("X"=w2730) -> ("mean"=w2728:dbl)  [unwired: 1 out]
                        "BLE AVG-Interval Graph" <- w2728
                        n1815 = local write "BLE Interval Time(ms)"(w2728) -> ()
                        n1816 = call "SUB-Interval_Realtime-Average.vi"("Mode"=enum16{"Add", "Reset"}."Add", "Input"=w2728) -> ("Average"=→"BLE Interval Time Avg(ms)":dbl)  [unwired: 9 in]
                      }
                    }
                    n1817 = case shown="0, 기본" w2721 {
                      frame 0, Default {
                        w2732 = T5 3 items=["System", "Persistent Store", "Attribute database", "Connection", "Attribute client", "Security Manager", "Generic Access Profile", "Hardware"] ("Command Class (System)")
                        w2735 = T4 0 items=["Command / Response"=0, "Event"=128] ("Message Type (Command / Response)")
                        # "Get Rssi"
                        n1818 = local read "Port-act 1"() -> (w2736:refnum<visa-resource-name>)
                        n1819 = Build Array(u8 0 ("Message ID (0x00)")) -> (w2733:u8[])
                        n1820 = call "ble_write_message.vi"("Command Class (System)"=w2732, "Message Type (Command / Response)"=w2735, "Payload(Empty)"=w2733, "Message ID (0x00)"=u8 1, "COM Bluegiga in"=w2736) -> ()  [unwired: 4 in, 3 out]
                      }
                      frame 1 {
                      }
                    }
                    n1821 = case shown="참" w2713 {
                      tunnel: w2712 -> [_ w2723]
                      frame False {
                      }
                      frame True {
                        n1822 = call-poly <vilib>:"Mean.vi"("X"=w2723) -> ("mean"=w2725:dbl)  [unwired: 1 out]
                        "BLE RSSI Graph" <- w2725
                        n1823 = local write "BLE RSSI (dBm)"(w2725) -> ()
                        n1824 = call "SUB-RSSI_Realtime-Average.vi"("Mode"=enum16{"Add", "Reset"}."Add", "Input"=w2725) -> ("Average"=→"BLE RSSI Avg(dBm)":dbl)  [unwired: 9 in]
                      }
                    }
                  }
                }
              }
            }
            n1825 = case shown="참" "Grahp Clear" {
              frame False {
              }
              frame True {
                n1826 = local write "BLE Interval Time(ms)"(0.0 ("BLE Interval Time(ms)")) -> ()
                n1827 = property on="BLE Interval buf" class="WFChart (엄격한)"("History Data"=u32[] [] ("히스토리 데이터")) -> ()  [unwired: 2 in, 2 out]
                n1828 = property on="BLE Interval Graph" class="WFChart (엄격한)"("History Data"=dbl[] [] ("히스토리 데이터")) -> ()  [unwired: 2 in, 2 out]
                n1829 = property on="BLE RSSI buf" class="WFChart (엄격한)"("History Data"=i16[] [] ("히스토리 데이터")) -> ()  [unwired: 2 in, 2 out]
                n1830 = local write "BLE RSSI (dBm)"(0.0 ("BLE RSSI (dBm)")) -> ()
                n1831 = property on="BLE RSSI Graph" class="WFChart (엄격한)"("History Data"=i16[] [] ("히스토리 데이터")) -> ()  [unwired: 2 in, 2 out]
                n1832 = call "SUB-BLE Rx data Clear.vi"() -> ()  [unwired: 6 in]
              }
            }
            n1833 = case shown="참" "CDC Graph plot" {
              frame False {
              }
              frame True {
                n1834 = control-ref of="CDC(PCAP02) Graph"() -> (w2706:refnum<vi>)
                n1835 = local write "Clear graph 1"(TRUE ("그래프 지우기")) -> ()
                n1836 = call "SUB-Graph plot select.vi"("CDC(PCAP02) Graph 2"=w2706) -> ()  [unwired: 3 in]
              }
            }
          }
          frame #15 {
            n1837 = case shown="거짓" "All Graph data save" {
              frame False {
              }
              frame True {
                n1838 = control-ref of="BLE AVG-Interval Graph"() -> (w2756:refnum<vi>)
                n1839 = control-ref of="BLE RSSI Graph"() -> (w2757:refnum<vi>)
                n1840 = property class="WFChart (엄격한)"(reference=w2756) -> ("History Data"=w2751:dbl[])  [unwired: 1 in, 2 out]
                n1841 = property class="WFChart (엄격한)"(reference=w2757) -> ("History Data"=w2752:dbl[])  [unwired: 1 in, 2 out]
                n1842 = Array Size(array=w2752) -> (size(s)=w2755:i32)
                n1843 = for {
                  N: w2755 -> [_]
                  tunnel: [w2760] -> w2754 mode=indexing
                  i -> [w2760]
                }
                n1844 = To Double Precision Float(number=w2754) -> (double precision float=w2753:dbl[])
                n1845 = Build Array(w2753, w2752, w2751) -> (w2750:dbl[][])
                n1846 = Transpose 2D Array(2D array=w2750) -> (transposed array=w2749:dbl[][])
                n1847 = call "Save_Array_Data_to_File.vi"("Header Array"=string[] ["Index", "RSSI(dB)", "Interval Time(ms)"], "Array"=w2749, "file path (use dialog)"="File path") -> ()  [unwired: 8 in, 1 out]
              }
            }
            n1848 = case shown="참" "Reset Avg" {
              frame False {
              }
              frame True {
                n1849 = call "SUB-RSSI_Realtime-Average.vi"("Mode"=enum16{"Add", "Reset"}."Reset") -> ("Average"=w2745:dbl)  [unwired: 10 in]
                n1850 = call "SUB-Interval_Realtime-Average.vi"("Mode"=enum16{"Add", "Reset"}."Reset") -> ("Average"=w2746:dbl)  [unwired: 10 in]
                n1851 = property on="BLE Interval Time Avg(ms)" class="DigNum (엄격한)"("Value"=w2746) -> ()  [unwired: 2 in, 2 out]
                n1852 = property on="BLE RSSI Avg(dBm)" class="DigNum (엄격한)"("Value"=w2745) -> ()  [unwired: 2 in, 2 out]
              }
            }
          }
        }
        n1853 = Wait Until Next ms Multiple(millisecond multiple=u32 4 ("ms 배수")) -> ()  [unwired: 1 out]
        n1854 = local read "stop"() -> (w1173:bool)
      }
    }
    frame #6 {
      # "Close Serial Port"
      n1855 = local read "Comm con 1"() -> (w2761:bool)
      n1856 = case shown="참" w2761 {
        frame False {
        }
        frame True {
          # "BLE 통신 종료"
          n1857 = local read "Port-act 1"() -> (w2762:refnum<visa-resource-name>)
          n1858 = local read "Connection Status"() -> (w2767:T6)
          n1859 = call "_Serial_buf clear.vi"("Serial Port"=w2762) -> ("에러 출력"=w2765:errorcluster, "Serial Port 2"=w2766:refnum<visa-resource-name>)  [unwired: 3 in]
          n1860 = call "ble_disconnect_device.vi"("Connection Status"=w2767, "error in (no error)"=w2765, "COM Bluegiga in"=w2766) -> ("error out"=w2764:errorcluster, "COM Bluegiga out"=w2763:refnum<visa-resource-name>)  [unwired: 7 in]
          n1861 = VISA Close(VISA resource name=w2763, error in (no error)=w2764) -> ()  [unwired: 1 out]
        }
      }
    }
    frame #7 {
      # "Save Program Configuration to File"
      n1862 = call <vilib>:"Open Config Data.vi"("configuration file path"=w2772) -> ("error out"=w2775:errorcluster, "refnum"=w2774:T32)  [unwired: 2 in, 7 out]
      n1863 = stacked-sequence {
        tunnel: w2774 -> [w2779 w2782 w2787 w2792 w2797]
        tunnel: w2775 -> [w2778 w2781 w2786 w2791 w2796]
        tunnel: "GUI Setting" ("section") -> [w2780 w2783 w2788 w2793 _]
        tunnel: [_ _ _ _ w2797] -> w2771
        tunnel: [_ _ _ _ w2796] -> w2770
        frame #0 {
          w2777 = "Com Port-Board1"  # Key 1
          n1864 = local read "Port-set 1"() -> (w2776:refnum<visa-resource-name>)
          n1865 = call-poly <vilib>:"Write Key.vi"("section"=w2780, "error in (no error)"=w2778, "value"=w2776, "key"=w2777, "refnum"=w2779) -> ()  [unwired: 1 in, 6 out]
        }
        frame #1 {
          w2785 = "Com Port-FTS"  # Key 1
          n1866 = local read "Port-FTS"() -> (w2784:refnum<visa-resource-name>)
          n1867 = call-poly <vilib>:"Write Key.vi"("section"=w2783, "error in (no error)"=w2781, "value"=w2784, "key"=w2785, "refnum"=w2782) -> ()  [unwired: 1 in, 6 out]
        }
        frame #2 {
          w2790 = "Logno"  # Key 1
          n1868 = local read "Log no"() -> (w2789:string)
          n1869 = call-poly <vilib>:"Write Key.vi"("section"=w2788, "error in (no error)"=w2786, "value"=w2789, "key"=w2790, "refnum"=w2787) -> ()  [unwired: 1 in, 6 out]
        }
        frame #3 {
          w2795 = "Interval(ms)"  # Key 1
          n1870 = local read "Update(ms)"() -> (w2794:u16)
          n1871 = call-poly <vilib>:"Write Key.vi"("section"=w2793, "error in (no error)"=w2791, "value"=w2794, "key"=w2795, "refnum"=w2792) -> ()  [unwired: 7 out]
        }
        frame #4 {
        }
      }
      n1872 = call <vilib>:"Close Config Data.vi"("error in (no error)"=w2770, "refnum"=w2771) -> ()  [unwired: 1 in, 9 out]
      n1873 = call "Read and Write Controls to Automatic Config File.vi"("Action"=RWC_Actions."Write", "Control References"=w2768) -> ()  [unwired: 9 in, 1 out]
    }
    frame #8 {
      # "End"
      n1874 = call "SUB-Exit.vi"() -> ()  [unwired: 4 in]
    }
  }
  n1875 = control-ref of="Log no"() -> (w2:refnum<vi>)
  n1876 = local write "Mode"(TRUE ("Mode")) -> ()
  n1877 = local write "Rx-debug"(FALSE ("Rx-debug")) -> ()
  n1878 = local write "Offset Souce"(enum32{"Normal", "Raw"}."Normal" ("Offset Souce")) -> ()
  n1879 = control-ref of="Linerity State"() -> (w3:refnum<vi>)
  n1880 = property class="Enum (엄격한)"(reference=w3, "Value"=Linerity_State."Initial" ("Linerity State")) -> ()  [unwired: 1 in, 2 out]
  n1881 = local write "Packet No."(0 ("Packet No.")) -> ()
  n1882 = property class="Str"(reference=w2, "DisabledEnum"=T15."Enabled" ("비활성화")) -> ()  [unwired: 1 in, 2 out]
